vi "Civ idle3.vi"() -> ()   [LabVIEW 2013]
uses:
  <vilib>/Analysis/Matrix/Numeric/Conversions/Matrix To Array - RM.vi
  <vilib>/Analysis/Matrix/NI_Matrix.lvlib
panel:
  out "Base dissent":dbl format="%#_4g"
  out "Gold":i64 format="%^#.4g"
  out "Dissent \nmultiplication\nmodifier":dbl
  out "SP income":dbl format="%^#.3g"
  out "EP income":dbl format="%^#.3g"
  out "Land conversion rate":dbl format="%#_4e"
  out "BP income":dbl format="%^#.3g"
  in  "Ticks/s":i32
  out "Gold upkeep":dbl format="%^#_4g"
  out "Gold income/s":dbl format="%^#_4g"
  out "BP upkeep":dbl format="%^#.3g"
  out "Trading level":i32
  out "Build points":dbl format="%^#.3g"
  in  "?":T1(tab)
  out "%Hunters":dbl format="%#_3g"
  in  "%Crafters":dbl
  in  "%Engineers":dbl
  in  "%Scientists":dbl
  in  "%Builders":dbl
  in  "%Warriors":dbl
  in  "Taxes level 0":bool
  in  "Taxes level 1":bool
  in  "Taxes level 2":bool
  in  "Taxes level 3":bool
  out "Taxation\nlevel":dbl format="%#_13g"
  in  "Taxes level 4":bool
  out "Food consumption\nmultiplier":dbl
  out "Food dissent mod":dbl
  in  "Normal food\nconsumption":bool
  in  "Highest food\nconsumption":bool
  in  "Higher food\nconsumption":bool
  in  "Taxes level 5":bool
  in  "Taxes level 6":bool
  out "Military\nScience level":i32
  out "Governance\nlevel":i32
  in  "Military science":bool
  in  "Governance":bool
  in  "Physics":bool
  in  "Construction":bool
  out "Physics level":i32
  out "Construction\nlevel":i32
  out "Economics\nlevel":i32
  in  "Economics":bool
  in  "Biology":bool
  out "Biology\nlevel":i32
  out "# of level 1 sciences":i32
  out "# of level 2 sciences":i32
  out "# of level 3 sciences":i32
  out "# of level 4 sciences":i32
  out "# of level 5 sciences":i32
  out "# of level 6 sciences":i32
  out "# of level 7 sciences":i32
  out "# of level 8 sciences":i32
  out "# of level 9 sciences":i32
  out "# of level 10 sciences":i32
  out "Production\nlevel":i32
  in  "Production":bool
  out "Level 2 science price":i32 format="%^.0g"
  out "Level 1 science price":i32 format="%^.0g"
  out "Level 6 science price":i64 format="%^#.1g"
  out "Level 5 science price":i32 format="%^.0g"
  out "Level 4 science price":i32 format="%^.0g"
  out "Level 7 science price":i64 format="%^.0g"
  out "Level 3 science price":i32 format="%^#.1g"
  out "Level 8 science price":i64 format="%^.0g"
  out "Level 9 science price":i64 format="%^#.1g"
  out "Level 10 science price":i64 format="%.0g"
  out "Spear level":i32
  out "Net level":i32
  in  "Sharpened stick":bool
  in  "Net 1":bool
  in  "Net 2":bool
  in  "Stone\nspear":bool
  in  "Bronze\nSpear":bool
  in  "Iron\nSpear":bool
  out "Construction\ntools level":i32
  in  "Stone tools":bool
  in  "Basic\nmetal\ntools":bool
  in  "Advanced\nmetal\ntools":bool
  in  "Horses":bool
  in  "Selective\nbreeding":bool
  in  "Livestock":bool
  out "Animal\ndomestication\nlevel":i32
  in  "Parchment":bool
  in  "Paper":bool
  in  "Movable typeset":bool
  out "Writing level":i32
  in  "Medicine 3":bool
  in  "Medicine 2":bool
  in  "Medicine 1":bool
  out "Medicine level":i32
  in  "Medicine 4":bool
  in  "Printing\nPress":bool
  in  "Crossbow":bool
  out "Bow level":i32
  in  "Bow 1":bool
  in  "Bow 2":bool
  in  "Longbow":bool
  in  "Farming 1":bool
  out "Farming level":i32
  in  "Farming 2":bool
  out "Sword level":i32
  in  "Steel sword":bool
  in  "Iron sword":bool
  in  "Bronze sword":bool
  out "Tax method\nlevel":i32
  in  "Income tax":bool
  in  "Sales tax":bool
  in  "Tariffs":bool
  out "Siege weapon\nlevel":i32
  in  "Trebuchet":bool
  in  "Catapult":bool
  in  "Ballista":bool
  in  "Cannon":bool
  in  "Howitzer":bool
  in  "Rocket artillery":bool
  in  "Trireme":bool
  in  "Raft":bool
  out "Boat level":i32
  out "Chariot level":i32
  in  "Reinforced\nchariot":bool
  in  "Simple\nchariot":bool
  in  "Caravan":bool
  in  "Caravel":bool
  in  "Steamship":bool
  in  "Mechanical\nTelevision":bool
  out "Optics\nlevel":i32
  in  "Telescope":bool
  in  "Light bulb":bool
  in  "Camera":bool
  in  "LCD monitor":bool
  out "Electronics\nlevel":i32
  in  "Radio":bool
  in  "Computer":bool
  out "Vehicle\nlevel":i32
  in  "Steam Powered Train":bool
  in  "Internal combustion engine (cars)":bool
  in  "Aircraft":bool
  in  "Rocket":bool
  in  "Democracy":bool
  in  "Theocracy":bool
  in  "Warrior\nSociety":bool
  in  "Democracy 2":bool
  in  "Theocracy 2":bool
  in  "Warrior\nSociety 2":bool
  in  "Kingdom":bool
  in  "Republic":bool
  in  "Confederacy":bool
  in  "Senate":bool
  in  "Caste system":bool
  in  "Feudalism":bool
  in  "Harbor level 0":bool
  in  "Harbor level 3":bool
  in  "Harbor level 2":bool
  in  "Harbor level 1":bool
  out "Brick house level":i32
  out "Road level":i32
  out "Hut level":i32
  in  "Hut level 0":bool
  in  "Hut level 1":bool
  in  "Hut level 2":bool
  in  "Hut level 3":bool
  out "Road invested points":dbl
  out "Hut invested points":dbl
  in  "Road level 0":bool
  in  "Road level 3":bool
  in  "Road level 2":bool
  in  "Road level 1":bool
  out "Aqueduct level":i32
  out "Circus\ninvested points":dbl
  out "Circus/arena level":i32
  out "Aqueduct\ninvested points":dbl
  out "Harbor\ninvested points":dbl
  out "Harbor level":i32
  in  "Aqueduct\nlevel 1":bool
  in  "Aqueduct\nlevel 4":bool
  in  "Aqueduct\nlevel 3":bool
  in  "Aqueduct\nlevel 2":bool
  out "School invested points":dbl
  in  "School\nlevel 1":bool
  in  "School\nlevel 2":bool
  in  "School\nlevel 3":bool
  in  "School\nlevel 0":bool
  out "School level":i32
  in  "Wall level 1":bool
  in  "Wall level 2":bool
  in  "Wall level 3":bool
  in  "Wall level 0":bool
  out "Barracks level":i32
  out "Walls level":i32
  out "Wall invested points":dbl
  out "Barracks\ninvested points":dbl
  in  "Barracks\nlevel 3":bool
  in  "Barracks\nlevel 1":bool
  in  "Barracks\nlevel 0":bool
  in  "Barracks\nlevel 2":bool
  out "University level":i32
  in  "University\nlevel 0":bool
  in  "University\nlevel 3":bool
  in  "University\nlevel 2":bool
  in  "University\nlevel 1":bool
  out "University\ninvested points":dbl
  out "Mansion level":i32
  out "Temple level":i32
  out "Mansion\ninvested points":dbl
  out "Temple\ninvested points":dbl
  in  "Temple\nlevel 0":bool
  in  "Temple\nlevel 3":bool
  in  "Temple\nlevel 2":bool
  in  "Temple\nlevel 1":bool
  in  "Make Tier 2\nproducts":bool
  out "Tier 2\nproducts\nupkeep":dbl format="%#_13g"
  out "Tier 3\nproducts\nupkeep":dbl format="%#_13g"
  out "Tier 4\nproducts\nupkeep":dbl format="%#_13g"
  out "Tier 1\nproducts":dbl format="%#_4p"
  out "Tier 2\nproducts":dbl format="%#_13g"
  out "Tier 3\nproducts":dbl format="%#_13g"
  out "Tier 4\nproducts":dbl format="%#_13g"
  out "Tier 1\nproducts\nupkeep":dbl format="%#_13g"
  in  "Make Tier3\nproducts":bool
  in  "Make Tier 4\nproducts":bool
  out "hunting b":dbl
  out "hunting a":dbl
  out "warrior a":dbl
  out "warrior b":dbl
  out "warrior c":dbl
  out "1-Dissent/100":dbl format="%#_13g"
  out "Land conv mult":dbl
  out "Warrior b Gov mult":dbl
  out "Gov Economy\nbuildings mod":dbl
  out "Dissent mult per\nmilitary building":dbl
  out "Temp land change/s":dbl
  out "Year":i32
  out "Day":i32
  out "Military Modifier":dbl format="%#_13g"
  out "Taxation\nModifier":dbl format="%#_13g"
  out "Non-land production multiplier":dbl
  out "Hut non-land prod mod":dbl
  out "Hut upkeep":dbl
  out "Hut dissent mod":dbl
  out "Road land prod mod":dbl
  out "Road upkeep":dbl
  out "Road expansion bonus":dbl
  out "Trading level no mod":i32
  out "Taxes dissent mod":dbl
  out "Barracks military bonus":dbl
  out "Barracks upkeep":dbl
  out "Wall upkeep":dbl
  out "Wall dissent mod":dbl
  out "Construction multiplier":dbl
  out "Wall warrior % equivalent":dbl
  out "Gov building\nupkeep mod":dbl
  out "School dissent mod":dbl
  out "School upkeep":dbl
  out "School engineer equivalent":dbl
  out "School SP/EP multiplier":dbl
  out "Medicine dissent mod":dbl
  out "Gov populist\nbuildings mod":dbl
  out "Gov elitist\nbuildings mod":dbl
  out "University SP multiplier":dbl
  out "University dissent mod":dbl
  out "University upkeep":dbl
  out "University scientist equivalent":dbl
  out "Food income":dbl
  out "Gold dbl":dbl format="%#_13g"
  out "Aqueduct dissent mod":dbl
  out "Aqueduct upkeep":dbl
  out "Mansion dissent mod":dbl
  out "Mansion upkeep":dbl
  out "Harbor expansion bonus":dbl
  out "Harbor upkeep":dbl
  out "Circus dissent mod":dbl
  out "Circus upkeep":dbl
  out "Temple dissent mod":dbl
  out "Temple upkeep":dbl
  out "Harbor military mod":dbl
  out "SP/EP multiplier":dbl
  out "Temple SP/EP multiplier":dbl
  out "Aqueduct food multiplier":dbl
  out "Government":string
  out "Dissent":dbl format="%#_4g"
  out "SP":dbl format="%^#.3g"
  out "EP":dbl format="%^#.3g"
  in  "Percentage or absolute":bool
  out "Engineers":i32 format="%^#.3g"
  out "Crafters":i32 format="%^#.3g"
  out "Scientists":i32 format="%^#.3g"
  in  "#Merchants":dbl
  in  "Assign Merchant":bool
  in  "#Engineers":dbl
  in  "Assign Engineer":bool
  in  "#Scientists":dbl
  in  "Assign Scientist":bool
  out "Warriors":i32 format="%^#.3g"
  in  "Assign Builder":bool
  in  "#Builders":dbl
  out "Builders":i32 format="%^#.3g"
  in  "Assign Warrior":bool
  in  "#Warriors":dbl
  out "Unassigned workers":i32
  in  "Assign Hunters":bool
  in  "#Hunters":dbl
  in  "# people":i32
  in  "Increase\nPopulation":bool
  out "Conquered\nland":dbl format="%^#.3g"
  out "Max hunters":i32 format="%^#.3g"
  out "Hunters":i32 format="%^#.3g"
  out "Food/s":dbl format="%^#_5g"
  out "Permanent\nland":dbl format="%^#.3g"
  out "People":i64 format="%^#.3g"
  in  "Stop Loop":bool
  out "Food":dbl format="%^#_5g"
  # "Produces food, but your permanent land cannot support too many hunters"
  # "Unlock after population hits 25"
  # "Conquers land, starting at 1km^2 per warrior, but has diminishing returns"
  # "Unlock after construction 1"
  # "Produces 1 BP/tick, needed for buildings\nand for building upkeep"
  # "Unlock after population hits 100"
  # "Produces 0.1 SP/tick, used for abstract research which unlock upgrades and provide bonuses"
  # "Unlock after population hits 50"
  # "Produces 0.1 EP/tick, used for designing useful tools and upgrades"
  # "Produces Products, used mostly for late game upgrades.  Production scales with permanent land"
  # "Not yet implemented"
  # "Small income from population, 8% dissent before modifiers"
  # "Medium income from population, 15% dissent before modifiers"
  # "Higher  income from population, 25% dissent before modifiers"
  # "Higher  income from population, 40% dissent before modifiers"
  # "Highest  income from population, 60% dissent before modifiers"
  # "No income from population, no dissent added"
  # "Lowest income from population, 3% dissent before modifiers"
  # "Requires Economics 1"
  # "2 food/s/person,\n-20% dissent"
  # "1 food/s/person, no dissent mod"
  # "1.5 food/s/person,\n-10% dissent"
  # "Requires Governance 2"
  # "Each level costs 1000 *10^current level SP"
  # "Reduces diminishing returns \nfrom military size, unlocks \nnew weapons/tactics"
  # "-5% dissent per level,\nunlocks new governments"
  # "Increases EP and SP generation, \nunlocks various upgrades"
  # "Decreases building upkeep costs,\nunlocks buildings"
  # "Increase gold generation,\nunlocks gold and taxation"
  # "Increase food production,\nunlocks farming and medicine"
  # "Increases production by 20%\nper tier per level"
  # "Costs 2M EP\nRequires military 4,\nWarriors are more effective"
  # "Costs 250EP\nHunters and warriors are more effective"
  # "Costs 3000EP\nRequires military 1,\nHunters and warriors are more effective"
  # "Costs 50k EP\nRequires military 2,\nWarriors are more effective"
  # "Costs 3k EP\nRequires biology 1,\nreduces dissent by 3%"
  # "Costs 30k EP\nRequires biology 2,\nreduces dissent by another 2% (5% total)"
  # "Costs 3M EP\nRequires biology 4,\nreduces dissent by another 5% (10% total)"
  # "Costs 300M EP\nRequires biology 6,\nreduces dissent by another 5% (15% total)"
  # "Costs 10k EP\nHunters can produce more food"
  # "Costs 100k EP\nHunters can produce more food"
  # "Costs 10k EP\nImproves EP and SP production by 10%"
  # "Costs 1M EP\nImproves EP and SP production by 10%"
  # "Costs 100M EP\nImproves EP and SP production by 10%"
  # "Costs 10B EP\nImproves EP and SP production by 10%"
  # "Costs 30k EP\nRequires physics 2, construction 2\nBuilders produce 0.5 more BP/tick"
  # "Costs 500k EP\nRequires physics 3,\nconstruction 3,Builders produce 0.5 more BP/tick"
  # "Costs 200M EP\nRequires physics 5,\nconstruction 5,Builders produce 1 more BP/tick"
  # "Costs 30M EP\nRequires Biology 3\nImproves warrior effectiveness,  builder BP/tick by 0.5"
  # "Costs 30k EP\nRequires Biology 1\nImproves hunter food production"
  # "Costs 1M EP\nRequires Biology 2\nImproves warrior effectiveness,  builder BP/tick by 0.5"
  # "Costs 100k EP\nRequires military 3,\nWarriors are much more effective, hunters can produce more food"
  # "Costs 300k EP\nRequires military 3, physics 3\nWarriors and Hunters are more effective"
  # "Costs 30M EP\nRequires military 5, physics 4\nWarriors are more effective"
  # "Costs 1B EP\nRequires military 6, physics 5\nWarriors are more effective"
  # "Costs 300k EP\nRequires physics 3,\nImproves trade and hunting"
  # "Costs 3M EP\nRequires physics 4, military 3\nImproves trade and warriors"
  # "Costs 10B EP\nRequires physics 7\nIncreases trade level by 2 and improves warriors"
  # "Costs 100B EP\nRequires physics 8, military 8\nIncreases trade level by 2 and improves warriors"
  # "Costs 500k EP\nRequires Military 3, Physics 3, Improves warrior effectiveness"
  # "Costs 5M EP\nRequires Military 3, Physics 4, Improves warrior effectiveness"
  # "Costs 10M EP\nRequires Economics 4, Physics 4, Increases trade level"
  # "Costs 1M EP\nRequires Military 3\nImproves warrior effectiveness"
  # "Costs 30M EP\nRequires Military 4\nImproves warrior effectiveness"
  # "Costs 1B EP\nRequires Military 6\nImproves warrior effectiveness"
  # "Costs 1M EP\nRequires Economics 3\nImproves taxation effectiveness by 50%"
  # "Costs 30M EP\nRequires Economics 4\nImproves taxation effectiveness by 50%"
  # "Costs 1B EP\nRequires Economics 6\nImproves taxation effectiveness by 50%"
  # "Costs 10M EP\nRequires Biology 3\nRenames hunters to farmers, massive improvements to food production, increases food from tribute"
  # "Costs 100M EP\nRequires Biology 4\nLarge improvements to food production, increases food from tribute"
  # "Costs 5M EP\nRequires Military 3, Physics 4, Improves\nwarrior effectiveness"
  # "Costs 30M EP\nRequires Military 3, Physics 5, Improves\nwarrior effectiveness"
  # "Costs 300M EP\nRequires Military 4, Physics 6, Improves\nwarrior effectiveness"
  # "Costs 3B EP\nRequires Military 6, Physics 7, Improves\nwarrior effectiveness"
  # "Costs 300B EP\nRequires Military 8, Physics 9, Improves\nwarrior effectiveness"
  # "Costs 3T EP\nRequires Military 9, Physics 9, Improves\nwarrior effectiveness"
  # "Internet, not sure if invention or building"
  # "Unlock sattelite network structure"
  # "Requires Governance 1"
  # "Costs 100k SP\nRequires Governance 2"
  # "Costs 5M SP\nRequires Governance 4"
  # "Reduces dissent by 5,10,15%\nImproves non-land production by 10,20,30%\nRequires Construction 1"
  # "Upkeep:        0                          0.01BP                0.03BP              0.15BP"
  # "Cost:             0                          10k   BP              30k BP            150k BP"
  # "Increases trade level by 1,2,3\nImproves land production\n by 10,20,30%\nImproves land conversion\nrate by 20,50,100%\nRequires Construction 1"
  # "Upkeep:        0                          0.02BP                0.06BP              0.2BP"
  # "Cost:             0                          50k BP              150k BP             500k BP"
  # "Improves food output\n by 10,20,30%\nReduced dissent by 2,4,6%\nRequires Construction 3"
  # "Upkeep:              0                       0.01BP                0.03BP               0.15BP"
  # "Cost:                   0                       500k BP             1.5M BP             5M BP"
  # "Increases trade level by 1,2,3\nIncreases military effectiveness (b) by 10,20,30%\nImproves land conversion\nrate by 10,25,50%\nRequires Boat level 1"
  # "Upkeep:        0                          0.04BP                0.12BP              0.4BP"
  # "Cost:             0                          500k BP              1.5M BP           5M BP"
  # "Increases military effectiveness (b) by 10,20,30%\nRequires Construction 2, Military 2"
  # "Upkeep:        0                          0.001GP             0.003GP             0.01GP"
  # "Cost:             0                          100k BP             300k BP              1M BP"
  # "Adds to the base strength of your military, giving the equivalent of 2,4,6% of your population as warriors\nReduces dissent by 5,10,15%\nRequires Construction 3, Military 2"
  # "Upkeep:        0                          0.002GP            0.006GP            0.02GP"
  # "Cost:             0                          1M BP              3M BP               10M BP"
  # "Provides a 5,10,15% bonus to SP/EP production, reduces dissent by 2,4,6%, adds 1,2,3% of population to base  engineers\nRequires Construction 2, Governance 2"
  # "Upkeep:        0                          0.001GP             0.003GP           0.01GP"
  # "Cost:             0                          200k BP             600k BP            2M BP"
  # "Provides a 15,30,45% bonus to SP production, reduces dissent by 2,4,6%, adds 2,4,6% of population to base  scientists\nRequires Construction 2, Governance 2"
  # "Upkeep:        0                          0.005GP             0.015GP          0.05GP"
  # "Cost:             0                          600k BP             2M BP             5M BP"
  # "Reduces dissent by 3,6,9%,\nRequires Construction 1"
  # "Upkeep:        0                          0.001GP             0.003GP           0.01GP"
  # "Cost:             0                          500 GP               10k GP             500k GP"
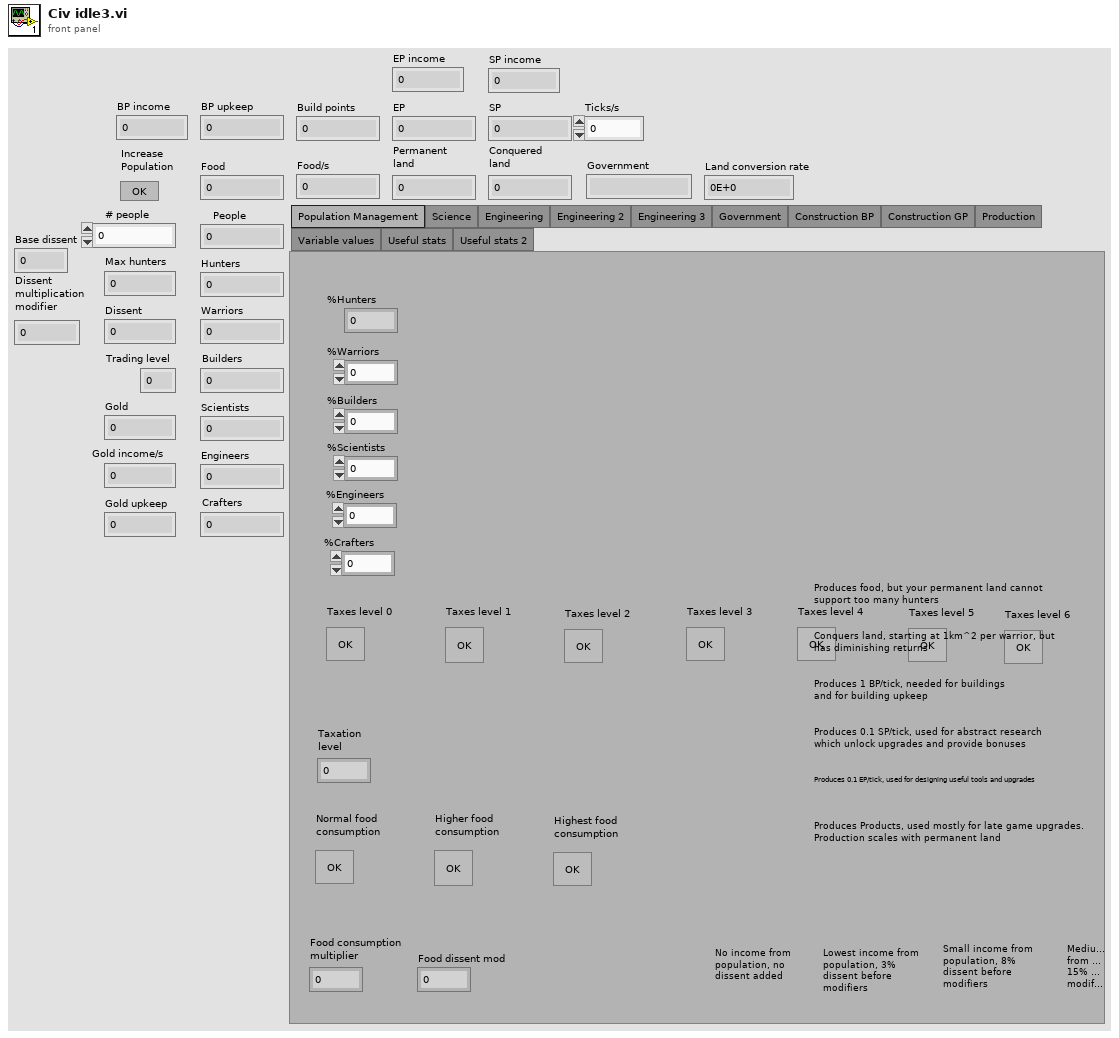
[diagram p1: front panel]
types:
  T1 = enum32{"Population Management", "Science", "Engineering", "Engineering 2", "Engineering 3", "Government", "Construction BP", "Construction GP", "Production", "Variable values", "Useful stats", "Useful stats 2"}
  T2 = typedef "NI_Matrix.lvlib/RealMatrix.ctl" = dbl[][]
diagram:
  n1 = while {
    i -> [w1979]
    stop <- "Stop Loop" stop-if-true
    w157 = 30000000 ("y")
    w166 = 30000000 ("y")
    w183 = 30000000 ("y")
    w192 = 30000000 ("y")
    w209 = 30000000 ("y")
    w224 = 30000000 ("y")
    w243 = 300000000 ("y")
    w254 = 300000000 ("y")
    w281 = 300000000 ("y")
    w292 = 30000000 ("y")
    w301 = 5000000 ("y")
    w332 = 3000000 ("y")
    w321 = 300000 ("y")
    w347 = 100000000 ("y")
    w358 = 300000000 ("y")
    w313 = 1000000000 ("y")
    w396 = 6 ("y")
    w399 = 5 ("y")
    w459 = 0 ("y")
    w458 = 3 ("y")
    w441 = 2 ("y")
    w440 = 1 ("y")
    w485 = 0 ("y")
    w486 = 3 ("y")
    w503 = 2 ("y")
    w504 = 1 ("y")
    w593 = 0 ("y")
    w592 = 3 ("y")
    w575 = 2 ("y")
    w574 = 1 ("y")
    w632 = i64 3000000000000 ("y")
    w643 = i64 300000000000 ("y")
    w664 = i64 3000000000 ("y")
    w701 = 300000000 ("y")
    w690 = 30000000 ("y")
    w681 = 5000000 ("y")
    w734 = 10000000 ("y")
    w745 = 5000000 ("y")
    w754 = 500000 ("y")
    w770 = 1000000000 ("y")
    w781 = 30000000 ("y")
    w790 = 1000000 ("y")
    w848 = 1000000000 ("y")
    w837 = 30000000 ("y")
    w828 = 1000000 ("y")
    w857 = 30000000 ("y")
    w868 = 1000000 ("y")
    w877 = 30000 ("y")
    w908 = 100000000 ("y")
    w897 = 1000000 ("y")
    w888 = 10000 ("y")
    w936 = 1 ("y")
    w928 = 2 ("y")
    w927 = 1.5 ("y")
    w971 = 0 ("y")
    w972 = 3 ("y")
    w991 = 2 ("y")
    w992 = 1 ("y")
    w1031 = 30000000 ("y")
    w1047 = 500000 ("y")
    w1065 = 3000000 ("y")
    w1076 = 30000 ("y")
    w1091 = 3000 ("y")
    w1148 = 0 ("y")
    w1147 = 3 ("y")
    w1128 = 2 ("y")
    w1127 = 1 ("y")
    w1174 = "Senate" ("y")
    w1198 = "Caste system" ("y")
    w1211 = "Feudalism" ("y")
    w1249 = "Kingdom" ("y")
    w1225 = "Republic" ("y")
    w1212 = "Confederacy" ("y")
    w1264 = 4 ("y")
    w1281 = 500000 ("y")
    w1292 = 30000 ("y")
    w1340 = 0 ("y")
    w1341 = 3 ("y")
    w1360 = 2 ("y")
    w1361 = 1 ("y")
    w1404 = 0 ("y")
    w1405 = 3 ("y")
    w1424 = 2 ("y")
    w1425 = 1 ("y")
    w1467 = 0 ("y")
    w1468 = 3 ("y")
    w1483 = 2 ("y")
    w1484 = 1 ("y")
    w1589 = 3 ("y")
    w1600 = 2 ("y")
    w1638 = 0 ("y")
    w1637 = 3 ("y")
    w1618 = 2 ("y")
    w1617 = 1 ("y")
    w1658 = 0 ("y")
    w1659 = 1 ("y")
    w1671 = 100000000 ("y")
    w1698 = 10000000 ("y")
    w1721 = 3000000 ("y")
    w1732 = 300000 ("y")
    w1764 = 300000 ("y")
    w1790 = 100000 ("y")
    w1793 = 2000000 ("y")
    w1792 = 50000 ("y")
    w1856 = "Warrior Society 2" ("y")
    w1880 = "Theocracy 2" ("y")
    w1893 = "Democracy 2" ("y")
    w1899 = "Warrior Society" ("y")
    w1912 = "Theocracy" ("y")
    w1926 = "Democracy" ("y")
    w1949 = 250 ("y")
    # "Constructions initial build"
    # "SCIENCES"
    # "GOVERNMENTS"
    # "ENGINEERING"
    n2 = local read "Food consumption\nmultiplier"() -> (w937:dbl)
    n3 = local read "Barracks\ninvested points"() -> (w1499:dbl)
    n4 = local read "Wall invested points"() -> (w1384:dbl)
    n5 = local read "Aqueduct\ninvested points"() -> (w418:dbl)
    n6 = local read "Food consumption\nmultiplier"() -> (w929:dbl)
    n7 = local read "Governance\nlevel"() -> (w934:i32)
    n8 = local read "Military\nScience level"() -> (w1326:i32)
    n9 = local read "Governance\nlevel"() -> (w942:i32)
    n10 = local read "Construction\nlevel"() -> (w1649:i32)
    n11 = local read "Construction\nlevel"() -> (w1352:i32)
    n12 = local read "Construction\nlevel"() -> (w1626:i32)
    n13 = local read "Construction\nlevel"() -> (w448:i32)
    n14 = local read "Gold dbl"() -> (w385:dbl)
    n15 = local read "Military\nScience level"() -> (w1313:i32)
    n16 = local read "Construction\nlevel"() -> (w1329:i32)
    n17 = local read "Build points"() -> (w1380:dbl)
    n18 = local read "Barracks level"() -> (w1644:i32)
    n19 = local read "Build points"() -> (w1503:dbl)
    n20 = local read "Military\nScience level"() -> (w1307:i32)
    n21 = local read "Walls level"() -> (w1334:i32)
    n22 = local read "Build points"() -> (w1643:dbl)
    n23 = local read "Build points"() -> (w1335:dbl)
    n24 = local read "Walls level"() -> (w1357:i32)
    n25 = local read "Barracks level"() -> (w1621:i32)
    n26 = local read "Build points"() -> (w422:dbl)
    n27 = Subtract(x=3000000 ("y"), y=w1384) -> (x-y=w1377:dbl)
    n28 = local read "Construction\nlevel"() -> (w469:i32)
    n29 = local read "Aqueduct level"() -> (w444:i32)
    n30 = local read "Aqueduct level"() -> (w465:i32)
    n31 = Subtract(x=300000 ("y"), y=w1499) -> (x-y=w1506:dbl)
    n32 = Greater Or Equal?(x=w942, y=2) -> (x >= y?=w944:bool)
    n33 = And(x="Normal food\nconsumption", y=w944) -> (x .and. y?=w940:bool)
    n34 = Subtract(x=10000 ("y"), y=w418) -> (x-y=w425:dbl)
    n35 = local read "Build points"() -> (w464:dbl)
    n36 = Greater Or Equal?(x=w934, y=2) -> (x >= y?=w946:bool)
    n37 = And(x="Highest food\nconsumption", y=w946) -> (x .and. y?=w932:bool)
    n38 = local read "Food consumption\nmultiplier"() -> (w918:dbl)
    n39 = local read "Ticks/s"() -> (w1255:i32)
    n40 = Not Equal?(x=w937, y=w936) -> (x != y?=w939:bool)
    n41 = And(x=w939, y=w940) -> (x .and. y?=w938:bool)
    n42 = Max & Min(x=w1377, y=0.0) -> (max(x,y)=w1382:dbl)  [unwired: 1 out]
    n43 = Greater Or Equal?(x=w1326, y=2) -> (x >= y?=w1324:bool)
    n44 = Not Equal?(x=w929, y=w928) -> (x != y?=w931:bool)
    n45 = And(x=w931, y=w932) -> (x .and. y?=w930:bool)
    n46 = local read "Aqueduct food multiplier"() -> (w471:dbl)
    n47 = Max & Min(x=w1506, y=0.0) -> (max(x,y)=w1501:dbl)  [unwired: 1 out]
    n48 = Greater Or Equal?(x=w1380, y=w1382) -> (x >= y?=w1381:bool)
    n49 = local write "Gold"(w385) -> ()
    n50 = Max & Min(x=w425, y=0.0) -> (max(x,y)=w420:dbl)  [unwired: 1 out]
    n51 = Greater Or Equal?(x=w422, y=w420) -> (x >= y?=w421:bool)
    n52 = local read "Military\nScience level"() -> (w1320:i32)
    n53 = Greater Or Equal?(x=w448, y=3) -> (x >= y?=w443:bool)
    n54 = Greater Or Equal?(x=w469, y=3) -> (x >= y?=w461:bool)
    n55 = Greater Or Equal?(x=w464, y=0) -> (x >= y?=w462:bool)
    n56 = Greater Or Equal?(x=w1503, y=w1501) -> (x >= y?=w1502:bool)
    n57 = Greater Or Equal?(x=w1649, y=2) -> (x >= y?=w1640:bool)
    n58 = Greater Or Equal?(x=w1329, y=3) -> (x >= y?=w1338:bool)
    n59 = Greater Or Equal?(x=w1643, y=0) -> (x >= y?=w1641:bool)
    n60 = Greater Or Equal?(x=w1335, y=0) -> (x >= y?=w1337:bool)
    n61 = Greater Or Equal?(x=w1352, y=3) -> (x >= y?=w1358:bool)
    n62 = Greater Or Equal?(x=w1313, y=2) -> (x >= y?=w1312:bool)
    n63 = Greater Or Equal?(x=w1626, y=2) -> (x >= y?=w1620:bool)
    n64 = Not Equal?(x=w444, y=w441) -> (x != y?=w446:bool)
    n65 = Not Equal?(x=w1644, y=w1638) -> (x != y?=w1646:bool)
    n66 = Not Equal?(x=w1334, y=w1340) -> (x != y?=w1332:bool)
    n67 = Not Equal?(x=w465, y=w459) -> (x != y?=w467:bool)
    n68 = Greater Or Equal?(x=w1307, y=2) -> (x >= y?=w1306:bool)
    n69 = Not Equal?(x=w1357, y=w1360) -> (x != y?=w1355:bool)
    n70 = Not Equal?(x=w1621, y=w1618) -> (x != y?=w1623:bool)
    n71 = for {
      N: 1 -> [_]
      tunnel: [w2874] -> w1607 mode=indexing
      n72 = local read "Production\nlevel"() -> (w2870:i32)
      n73 = local read "Permanent\nland"() -> (w2871:dbl)
      n74 = local read "Construction multiplier"() -> (w2900:dbl)
      n75 = local read "University scientist equivalent"() -> (w2887:dbl)
      n76 = local read "Taxation\nlevel"() -> (w2936:dbl)
      n77 = local read "1-Dissent/100"() -> (w2869:dbl)
      n78 = local read "Conquered\nland"() -> (w2951:dbl)
      n79 = local read "Non-land production multiplier"() -> (w2845:dbl)
      n80 = local read "Tier 2\nproducts"() -> (w2860:dbl)
      n81 = local read "Government"() -> (w2954:string)
      n82 = local read "University SP multiplier"() -> (w2884:dbl)
      n83 = local read "Economics\nlevel"() -> (w2937:i32)
      n84 = local read "SP/EP multiplier"() -> (w2893:dbl)
      n85 = local read "People"() -> (w2874:i64)
      n86 = local read "Conquered\nland"() -> (w2940:dbl)
      n87 = local read "Crafters"() -> (w2875:i32)
      n88 = local read "Economics\nlevel"() -> (w2942:i32)
      n89 = local read "Trading level"() -> (w2941:i32)
      n90 = local read "Taxation\nModifier"() -> (w2934:dbl)
      n91 = local read "Tax method\nlevel"() -> (w2878:i32)
      n92 = local read "Non-land production multiplier"() -> (w2925:dbl)
      n93 = local read "School engineer equivalent"() -> (w2896:dbl)
      n94 = local read "1-Dissent/100"() -> (w2927:dbl)
      n95 = local read "Physics level"() -> (w2928:i32)
      n96 = local read "Tier 2\nproducts\nupkeep"() -> (w2851:dbl)
      n97 = case shown="\"Imperialism\"" w2954 {
        tunnel: w2874 -> [w3002 w3009 w3029 w3047 w3055 w3074 w3085 w3107 w3122 w3144 w3157 w3177 w3190 w3219 w3231 w3244 _ _ _ _ _ _ _ _ _ _ _ _]
        tunnel: w2871 -> [_ w3019 w3030 _ _ _ _ w3112 w3121 _ w3162 _ w3192 _ _ w3246 _ _ _ _ _ _ _ _ _ _ _ _]
        tunnel: [w3005 w3016 w3022 w3044 w3058 w3067 w3087 w3104 w3120 w3133 w3150 w3171 w3186 w3207 w3227 w3239 _ _ _ _ _ _ _ _ _ _ _ _] -> w2952
        tunnel: w2951 -> [_ _ _ _ _ w3078 w3086 w3111 _ _ w3161 w3180 _ w3215 _ _ _ _ _ _ _ _ _ _ _ _ _ _]
        tunnel: [1 0.85 0.7 1 1 2 3 1.5 ("y") 1.0 ("y") 2.0 ("y") 3.0 ("y") 6.0 ("y") 0.7 ("y") 8.0 ("y") 2.0 ("y") 0.8 ("y") _ _ _ _ _ _ _ _ _ _ _ _] -> w2950
        tunnel: [1.0 2.0 4.0 1.0 1.0 0.1 0.025 1.5 ("y") 3.0 ("y") 1.0 ("y") 0.1 ("y") 0.025 ("y") 8.0 ("y") 0.015 ("y") 1.0 ("y") 8.0 ("y") _ _ _ _ _ _ _ _ _ _ _ _] -> w2949
        tunnel: [1 1 1 0.5 0.333 1 1 1.0 ("y") 0.5 ("y") 0.5 ("y") 1.0 ("y") 1.0 ("y") 1.0 ("y") 1.0 ("y") 0.5 ("y") 1.0 ("y") _ _ _ _ _ _ _ _ _ _ _ _] -> w2908
        tunnel: [1.0 ("y") 1.25 ("y") 1.5 ("y") 0.75 ("y") 0.5 ("y") 0.8 ("y") 0.7 ("y") 1.25 ("y") 2.0 ("y") 1.0 ("y") 0.5 ("y") 0.5 ("y") 2.5 ("y") 0.5 ("y") 1.0 ("y") 2.5 ("y") _ _ _ _ _ _ _ _ _ _ _ _] -> w2899
        tunnel: [1.0 ("y") 0.75 ("y") 0.5 ("y") 1.5 ("y") 2.0 ("y") 1.5 ("y") 1.5 ("y") 1.25 ("y") 0.5 ("y") 1.0 ("y") 1.5 ("y") 2.0 ("y") 0.5 ("y") 2.0 ("y") 1.0 ("y") 0.5 ("y") _ _ _ _ _ _ _ _ _ _ _ _] -> w2892
        tunnel: [1.0 ("y") 1.0 ("y") 1.0 ("y") 0.98 ("y") 0.98 ("y") 0.96 ("y") 0.96 ("y") 0.96 ("y") 1.0 ("y") 0.98 ("y") 0.96 ("y") 1.0 ("y") 1.0 ("y") 1.0 ("y") 0.98 ("y") 1.0 ("y") _ _ _ _ _ _ _ _ _ _ _ _] -> w2891
        tunnel: [1.0 ("y") _ _ _ _ _ _ 1.25 ("y") 1.5 ("y") 0.7 ("y") 0.5 ("y") 0.5 ("y") 1.0 ("y") 0.5 ("y") 0.7 ("y") 2.0 ("y") _ _ _ _ _ _ _ _ _ _ _ _] -> w2890
        frame "Tribe", Default {
          n98 = Divide(x=w3002, y=i64 4) -> (x/y=w3000:dbl)
          n99 = Subtract(x=w3000, y=i64 25) -> (x-y=w3005:dbl)
        }
        frame "Democracy" {
          n100 = Power Of X(1:w3009, 2:1.1 ("y")) -> (0:w3007:dbl)
          n101 = Square Root(x=w3019) -> (sqrt(x)=w3018:dbl)
          n102 = Divide(x=w3007, y=w3018) -> (x/y=w3017:dbl)
          n103 = Square Root(x=w3017) -> (sqrt(x)=w3021:dbl)
          n104 = Multiply(x=2, y=w3021) -> (x*y=w3016:dbl)
        }
        frame "Democracy 2" {
          n105 = Square Root(x=w3030) -> (sqrt(x)=w3034:dbl)
          n106 = Divide(x=w3029, y=w3034) -> (x/y=w3033:dbl)
          n107 = Square Root(x=w3033) -> (sqrt(x)=w3024:dbl)
          n108 = Multiply(x=w3024, y=1.9) -> (x*y=w3022:dbl)
        }
        frame "Theocracy" {
          n109 = Y-th Root of X(1:w3047, 2:i64 3 ("y")) -> (0:w3037:dbl)
          n110 = Multiply(x=w3037, y=2.0) -> (x*y=w3035:dbl)
          n111 = Add(x=w3035, y=10.0) -> (x+y=w3044:dbl)
        }
        frame "Theocracy 2" {
          n112 = Y-th Root of X(1:w3055, 2:3.5 ("y")) -> (0:w3049:dbl)
          n113 = Multiply(x=w3049, y=1.5) -> (x*y=w3050:dbl)
          n114 = Add(x=w3050, y=10.0) -> (x+y=w3058:dbl)
        }
        frame "Warrior Society" {
          n115 = Y-th Root of X(1:w3074, 2:i64 3 ("y")) -> (0:w3071:dbl)
          n116 = Y-th Root of X(1:w3078, 2:3.0 ("y")) -> (0:w3077:dbl)
          n117 = Multiply(x=3.5, y=w3071) -> (x*y=w3070:dbl)
          n118 = Add(x=w3070, y=5.0) -> (x+y=w3069:dbl)
          n119 = Multiply(x=w3077, y=2.0) -> (x*y=w3068:dbl)
          n120 = Subtract(x=w3069, y=w3068) -> (x-y=w3067:dbl)
        }
        frame "Warrior Society 2" {
          n121 = Y-th Root of X(1:w3085, 2:i64 3 ("y")) -> (0:w3095:dbl)
          n122 = Y-th Root of X(1:w3086, 2:3.0 ("y")) -> (0:w3091:dbl)
          n123 = Multiply(x=2.2, y=w3095) -> (x*y=w3096:dbl)
          n124 = Add(x=w3096, y=5.0) -> (x+y=w3097:dbl)
          n125 = Multiply(x=w3091, y=2.0) -> (x*y=w3098:dbl)
          n126 = Subtract(x=w3097, y=w3098) -> (x-y=w3087:dbl)
        }
        frame "Senate" {
          n127 = Multiply(x=w3112, y=w3111) -> (x*y=w3110:dbl)
          n128 = Power Of X(1:w3110, 2:0.3 ("y")) -> (0:w3108:dbl)
          n129 = Divide(x=w3107, y=w3108) -> (x/y=w3106:dbl)
          n130 = Y-th Root of X(1:w3106, 2:2.0 ("y")) -> (0:w3102:dbl)
          n131 = Multiply(x=1.5, y=w3102) -> (x*y=w3104:dbl)
        }
        frame "Republic" {
          n132 = Power Of X(1:w3121, 2:0.6 ("y")) -> (0:w3127:dbl)
          n133 = Divide(x=w3122, y=w3127) -> (x/y=w3126:dbl)
          n134 = Y-th Root of X(1:w3126, 2:2.0 ("y")) -> (0:w3123:dbl)
          n135 = Multiply(x=1.5, y=w3123) -> (x*y=w3120:dbl)
        }
        frame "Kingdom" {
          n136 = Power Of X(1:w3144, 2:0.25 ("y")) -> (0:w3135:dbl)
          n137 = Multiply(x=2.0, y=w3135) -> (x*y=w3133:dbl)
        }
        frame "Feudalism" {
          n138 = Multiply(x=w3162, y=w3161) -> (x*y=w3160:dbl)
          n139 = Y-th Root of X(1:w3157, 2:3.0 ("y")) -> (0:w3156:dbl)
          n140 = Y-th Root of X(1:w3160, 2:7.0 ("y")) -> (0:w3151:dbl)
          n141 = Divide(x=w3156, y=2.0) -> (x/y=w3154:dbl)
          n142 = Add(x=w3154, y=5.0) -> (x+y=w3152:dbl)
          n143 = Subtract(x=w3152, y=w3151) -> (x-y=w3150:dbl)
        }
        frame "Caste system" {
          n144 = Y-th Root of X(1:w3180, 2:3.5 ("y")) -> (0:w3167:dbl)
          n145 = Y-th Root of X(1:w3177, 2:3.5 ("y")) -> (0:w3176:dbl)
          n146 = Multiply(x=w3176, y=2.5) -> (x*y=w3174:dbl)
          n147 = Multiply(x=w3167, y=2.0) -> (x*y=w3166:dbl)
          n148 = Add(x=w3174, y=5.0) -> (x+y=w3172:dbl)
          n149 = Subtract(x=w3172, y=w3166) -> (x-y=w3171:dbl)
        }
        frame "Confederacy" {
          n150 = Power Of X(1:w3192, 2:0.55 ("y")) -> (0:w3189:dbl)
          n151 = Divide(x=w3190, y=w3189) -> (x/y=w3188:dbl)
          n152 = Square Root(x=w3188) -> (sqrt(x)=w3187:dbl)
          n153 = Multiply(x=1.7, y=w3187) -> (x*y=w3186:dbl)
        }
        frame "Imperialism" {
          n154 = Y-th Root of X(1:w3219, 2:3.75 ("y")) -> (0:w3217:dbl)
          n155 = Y-th Root of X(1:w3215, 2:3.75 ("y")) -> (0:w3213:dbl)
          n156 = Multiply(x=w3217, y=2.5) -> (x*y=w3211:dbl)
          n157 = Multiply(x=w3213, y=2.2) -> (x*y=w3210:dbl)
          n158 = Subtract(x=w3211, y=w3210) -> (x-y=w3209:dbl)
          n159 = Add(x=w3209, y=5.0) -> (x+y=w3207:dbl)
        }
        frame "Empire" {
          n160 = Y-th Root of X(1:w3231, 2:4.1 ("y")) -> (0:w3229:dbl)
          n161 = Multiply(x=w3229, y=1.5) -> (x*y=w3227:dbl)
        }
        frame "Free market capitalism" {
          n162 = Power Of X(1:w3246, 2:0.55 ("y")) -> (0:w3243:dbl)
          n163 = Divide(x=w3244, y=w3243) -> (x/y=w3242:dbl)
          n164 = Square Root(x=w3242) -> (sqrt(x)=w3241:dbl)
          n165 = Multiply(x=1.3, y=w3241) -> (x*y=w3239:dbl)
        }
        frame "Corporatism" {
        }
        frame "Fascism" {
        }
        frame "Communist dictatorship" {
        }
        frame "Socialism" {
        }
        frame "Advanced democracy?" {
        }
        frame "Advanced imperialism?" {
        }
        frame "Meritocracy" {
        }
        frame "Genetically optimized workforce" {
        }
        frame "Future democracy?" {
        }
        frame "Hivemind" {
        }
        frame "AI overlord" {
        }
        frame "Robots do all work" {
        }
      }
      n166 = Power Of X(1:w2874, 2:-0.5 ("y")) -> (0:w2872:dbl)
      n167 = Power Of X(1:1.2 ("x"), 2:w2870) -> (0:w2859:dbl)
      n168 = local read "Build points"() -> (w2902:dbl)
      n169 = local read "Build points"() -> (w2909:dbl)
      n170 = Compound Arithmetic op=MULTIPLY(w2875, w2845, w2872, w2871, w2859, w2869, 0.001 ("x")) -> (w2867:dbl)
      n171 = local read "Builders"() -> (w2911:i32)
      n172 = local read "Tier 3\nproducts"() -> (w2857:dbl)
      n173 = local read "Tier 1\nproducts"() -> (w2866:dbl)
      n174 = local read "Tier 1\nproducts\nupkeep"() -> (w2863:dbl)
      n175 = Add(x=w2867, y=w2866) -> (x+y=w2864:dbl)
      n176 = local read "Dissent"() -> (w2946:dbl)
      n177 = local read "Tier 3\nproducts\nupkeep"() -> (w2849:dbl)
      n178 = Power Of X(1:1.5 ("x"), 2:w2878) -> (0:w2876:dbl)
      n179 = local read "Tier 4\nproducts\nupkeep"() -> (w2848:dbl)
      n180 = Compound Arithmetic op=MULTIPLY(w2942, w2941, w2940, 0.001 ("value")) -> (w2907:dbl)
      n181 = local write "Dissent mult per\nmilitary building"(w2891) -> ()
      n182 = local read "Gold dbl"() -> (w2938:dbl)
      n183 = Compound Arithmetic op=MULTIPLY(w2874, w2937, w2936, w2934, 0.0005 ("value"), w2876) -> (w2906:dbl)
      n184 = local write "Gov populist\nbuildings mod"(w2899) -> ()
      n185 = local write "Gov elitist\nbuildings mod"(w2892) -> ()
      n186 = Power Of X(1:1.1 ("x"), 2:w2928) -> (0:w2913:dbl)
      n187 = Subtract(x=w2864, y=w2863) -> (x-y=w2844:dbl)
      n188 = Divide(x=w2902, y=10.0) -> (x/y=w2901:dbl)
      n189 = Compound Arithmetic op=ADD(w2938, w2907, w2906) -> (w2929:dbl)
      n190 = Divide(x=w2946, y=100.0) -> (x/y=w2948:dbl)
      n191 = local read "Dissent \nmultiplication\nmodifier"() -> (w2922:dbl)
      n192 = Compound Arithmetic op=MULTIPLY(w2913, w2927, 0.1, w2925, w2893) -> (w2914:dbl)
      n193 = Divide(x=w2914, y=w2913) -> (x/y=w2912:dbl)
      n194 = Compound Arithmetic op=MULTIPLY(w2912, 10.0 ("value"), w2911, w2900, w2893) -> (w2898:dbl)
      n195 = Add(x=w2898, y=w2909) -> (x+y=w2910:dbl)
      n196 = Less?(x=w2929, y=-50.0) -> (x < y?=w2932:bool)
      n197 = local read "Tier 4\nproducts"() -> (w2854:dbl)
      n198 = Greater?(x=w2844, y=0.0) -> (0:w2842:bool)
      n199 = Subtract(x=1.0, y=w2948) -> (x-y=w2944:dbl)
      n200 = Add(x=w2907, y=w2906) -> (x+y=w2905:dbl)
      n201 = local read "Engineers"() -> (w2895:i32)
      n202 = And(x="Make Tier 2\nproducts", y=w2842) -> (x .and. y?=w2840:bool)
      n203 = local write "Build points"(w2910) -> ()
      n204 = local write "Gold dbl"(w2929) -> ()
      n205 = local write "Gold income/s"(w2905) -> ()
      n206 = case shown="True" w2932 {
        tunnel: w2929 -> [_ w2990]
        tunnel: w2874 -> [_ w2994]
        tunnel: [0 w2991] -> w2919
        frame False {
        }
        frame True {
          n207 = Negate(x=w2990) -> (-x=w2989:dbl)
          n208 = Divide(x=w2989, y=w2994) -> (x/y=w2993:dbl)
          n209 = Max & Min(x=w2993, y=20.0) -> (min(x,y)=w2991:dbl)  [unwired: 1 out]
        }
      }
      n210 = local read "Scientists"() -> (w2888:i32)
      n211 = Less?(x=w2901, y=-50.0) -> (x < y?=w2921:bool)
      n212 = local write "1-Dissent/100"(w2944) -> ()
      n213 = local read "Taxes dissent mod"() -> (w2953:dbl)
      n214 = local write "Warrior b Gov mult"(w2950) -> ()
      n215 = Add(x=w2952, y=w2953) -> (x+y=w2829:dbl)
      n216 = case shown="True" w2840 {
        tunnel: w2844 -> [w2974 w2980]
        tunnel: w2859 -> [_ w2977]
        tunnel: [w2974 w2976] -> w2865
        tunnel: [0.0 w2975] -> w2861
        frame False {
        }
        frame True {
          n217 = Divide(x=100.0 ("y"), y=w2977) -> (x/y=w2979:dbl)
          n218 = Quotient & Remainder(x=w2980, y=w2979) -> (x-y*floor(x/y)=w2976:dbl, floor(x/y)=w2975:dbl)
        }
      }
      n219 = Add(x=w2861, y=w2860) -> (x+y=w2852:dbl)
      n220 = Subtract(x=w2852, y=w2851) -> (x-y=w2838:dbl)
      n221 = Greater?(x=w2838, y=0.0) -> (0:w2837:bool)
      n222 = And(x="Make Tier3\nproducts", y=w2837) -> (x .and. y?=w2835:bool)
      n223 = case shown="True" w2835 {
        tunnel: w2838 -> [w2966 w2972]
        tunnel: w2859 -> [_ w2969]
        tunnel: [w2966 w2968] -> w2858
        tunnel: [0.0 w2967] -> w2856
        frame False {
        }
        frame True {
          n224 = Divide(x=100.0 ("y"), y=w2969) -> (x/y=w2971:dbl)
          n225 = Quotient & Remainder(x=w2972, y=w2971) -> (x-y*floor(x/y)=w2968:dbl, floor(x/y)=w2967:dbl)
        }
      }
      n226 = local write "Tier 2\nproducts"(w2858) -> ()
      n227 = Add(x=w2856, y=w2857) -> (x+y=w2850:dbl)
      n228 = Subtract(x=w2850, y=w2849) -> (x-y=w2830:dbl)
      n229 = Greater?(x=w2830, y=0.0) -> (0:w2834:bool)
      n230 = And(x="Make Tier 4\nproducts", y=w2834) -> (x .and. y?=w2831:bool)
      n231 = case shown="True" w2831 {
        tunnel: w2830 -> [w2958 w2964]
        tunnel: w2859 -> [_ w2962]
        tunnel: [w2958 w2961] -> w2855
        tunnel: [0.0 w2960] -> w2847
        frame False {
        }
        frame True {
          n232 = Divide(x=100.0 ("y"), y=w2962) -> (x/y=w2959:dbl)
          n233 = Quotient & Remainder(x=w2964, y=w2959) -> (x-y*floor(x/y)=w2961:dbl, floor(x/y)=w2960:dbl)
        }
      }
      n234 = local write "Land conv mult"(w2949) -> ()
      n235 = Multiply(x=w2874, y=w2887) -> (x*y=w2886:dbl)
      n236 = case shown="True" w2921 {
        tunnel: w2874 -> [_ w2987]
        tunnel: [0 w2984] -> w2915
        tunnel: w2901 -> [_ w2982]
        frame False {
        }
        frame True {
          n237 = Negate(x=w2982) -> (-x=w2983:dbl)
          n238 = Divide(x=w2983, y=w2987) -> (x/y=w2986:dbl)
          n239 = Max & Min(x=w2986, y=20.0) -> (min(x,y)=w2984:dbl)  [unwired: 1 out]
        }
      }
      n240 = Add(x=w2919, y=w2915) -> (x+y=w2918:dbl)
      n241 = Multiply(x=w2829, y=w2922) -> (x*y=w2923:dbl)
      n242 = local read "EP"() -> (w2956:dbl)
      n243 = Multiply(x=w2896, y=w2874) -> (x*y=w2897:dbl)
      n244 = Subtract(x=w2847, y=w2848) -> (x-y=w2846:dbl)
      n245 = Add(x=w2846, y=w2854) -> (x+y=w2853:dbl)
      n246 = local read "SP"() -> (w2889:dbl)
      n247 = local write "Gov Economy\nbuildings mod"(w2890) -> ()
      n248 = Add(x=w2895, y=w2897) -> (x+y=w2894:dbl)
      n249 = Multiply(x=w2914, y=w2894) -> (x*y=w2883:dbl)
      n250 = local write "Gov building\nupkeep mod"(w2908) -> ()
      n251 = Max & Min(x=0.0, y=w2923) -> (max(x,y)=w2930:dbl)  [unwired: 1 out]
      n252 = Add(x=w2886, y=w2888) -> (x+y=w2885:dbl)
      n253 = Compound Arithmetic op=MULTIPLY(w2914, w2884, w2885) -> (w2882:dbl)
      n254 = Max & Min(x=w2918, y=20.0) -> (min(x,y)=w2916:dbl)  [unwired: 1 out]
      n255 = Add(x=w2916, y=w2930) -> (x+y=w2881:dbl)
      n256 = Add(x=w2956, y=w2883) -> (x+y=w2955:dbl)
      n257 = Add(x=w2889, y=w2882) -> (x+y=w2924:dbl)
      n258 = local write "Tier 3\nproducts"(w2855) -> ()
      n259 = Max & Min(x=99.0, y=w2881) -> (min(x,y)=w2879:dbl)  [unwired: 1 out]
      n260 = local write "Tier 4\nproducts"(w2853) -> ()
      n261 = local write "Tier 1\nproducts"(w2865) -> ()
      n262 = local write "BP income"(w2898) -> ()
      n263 = local write "EP"(w2955) -> ()
      n264 = local write "SP"(w2924) -> ()
      n265 = local write "SP income"(w2882) -> ()
      n266 = local write "EP income"(w2883) -> ()
      n267 = local write "Dissent"(w2879) -> ()
      n268 = Max & Min(x=w2829, y=0.0) -> (max(x,y)=→"Base dissent":dbl)  [unwired: 1 out]
    }
    n269 = case shown="True" w938 {
      tunnel: w936 -> [_ w2264]
      frame False {
      }
      frame True {
        n270 = local write "Food consumption\nmultiplier"(w2264) -> ()
        n271 = local write "Food dissent mod"(1.0 ("Taxes dissent add mod")) -> ()
      }
    }
    n272 = case shown="True" w930 {
      tunnel: w928 -> [_ w2266]
      frame False {
      }
      frame True {
        n273 = local write "Food consumption\nmultiplier"(w2266) -> ()
        n274 = local write "Food dissent mod"(0.8 ("Taxes dissent add mod")) -> ()
      }
    }
    n275 = local read "Road land prod mod"() -> (w1584:dbl)
    n276 = Max & Min(x=w1255, y=0.1) -> (max(x,y)=w1254:dbl)  [unwired: 1 out]
    n277 = local read "People"() -> (w919:i64)
    n278 = local read "hunting b"() -> (w2000:dbl)
    n279 = local read "hunting b"() -> (w1999:dbl)
    n280 = local read "Biology\nlevel"() -> (w1683:i32)
    n281 = And(x=w443, y=w421) -> (x .and. y?=w442:bool)
    n282 = And(x="Aqueduct\nlevel 3", y=w442) -> (x .and. y?=w447:bool)
    n283 = And(x=w446, y=w447) -> (x .and. y?=w445:bool)
    n284 = And(x=w461, y=w462) -> (x .and. y?=w460:bool)
    n285 = And(x="Aqueduct\nlevel 1", y=w460) -> (x .and. y?=w468:bool)
    n286 = And(x=w467, y=w468) -> (x .and. y?=w466:bool)
    n287 = case shown="True" w466 {
      tunnel: w459 -> [_ w2076]
      frame False {
      }
      frame True {
        n288 = local write "Aqueduct level"(w2076) -> ()
        n289 = local write "Aqueduct food multiplier"(1.0 ("Hut dissent add mod")) -> ()
        n290 = local write "Aqueduct dissent mod"(1.0 ("Aqueduct dissent mod")) -> ()
        n291 = local write "Aqueduct upkeep"(0.0 ("Hut non-land prod mod")) -> ()
      }
    }
    n292 = Compound Arithmetic op=AND(w1640, w1641, w1324) -> (w1639:bool)
    n293 = And(x="Barracks\nlevel 0", y=w1639) -> (x .and. y?=w1647:bool)
    n294 = And(x=w1646, y=w1647) -> (x .and. y?=w1645:bool)
    n295 = Compound Arithmetic op=AND(w1338, w1337, w1312) -> (w1339:bool)
    n296 = And(x="Wall level 0", y=w1339) -> (x .and. y?=w1331:bool)
    n297 = And(x=w1332, y=w1331) -> (x .and. y?=w1333:bool)
    n298 = Compound Arithmetic op=AND(w1358, w1381, w1306) -> (w1359:bool)
    n299 = And(x="Wall level 2", y=w1359) -> (x .and. y?=w1354:bool)
    n300 = And(x=w1355, y=w1354) -> (x .and. y?=w1356:bool)
    n301 = case shown="True" w445 {
      tunnel: w441 -> [_ w2094]
      tunnel: w420 -> [_ w2087]
      tunnel: w418 -> [_ w2086]
      frame False {
      }
      frame True {
        n302 = local read "Build points"() -> (w2093:dbl)
        n303 = Add(x=w2087, y=w2086) -> (x+y=w2089:dbl)
        n304 = local write "Aqueduct level"(w2094) -> ()
        n305 = local write "Aqueduct food multiplier"(1.2 ("Hut dissent add mod")) -> ()
        n306 = local write "Aqueduct dissent mod"(0.96 ("Hut dissent add mod")) -> ()
        n307 = local write "Aqueduct\ninvested points"(w2089) -> ()
        n308 = local write "Aqueduct upkeep"(0.03 ("Hut non-land prod mod")) -> ()
        n309 = Subtract(x=w2093, y=w2087) -> (x-y=w2092:dbl)
        n310 = local write "Build points"(w2092) -> ()
      }
    }
    n311 = local read "1-Dissent/100"() -> (w1848:dbl)
    n312 = case shown="True" w1356 {
      tunnel: w1360 -> [_ w2433]
      tunnel: w1382 -> [_ w2429]
      tunnel: w1384 -> [_ w2428]
      frame False {
      }
      frame True {
        n313 = local read "Build points"() -> (w2432:dbl)
        n314 = Add(x=w2429, y=w2428) -> (x+y=w2430:dbl)
        n315 = local write "Wall warrior % equivalent"(4.0 ("Hut dissent add mod")) -> ()
        n316 = local write "Walls level"(w2433) -> ()
        n317 = local write "Wall dissent mod"(0.9 ("Hut non-land prod mod")) -> ()
        n318 = local write "Wall invested points"(w2430) -> ()
        n319 = local write "Wall upkeep"(0.006 ("Hut non-land prod mod")) -> ()
        n320 = Subtract(x=w2432, y=w2429) -> (x-y=w2431:dbl)
        n321 = local write "Build points"(w2431) -> ()
      }
    }
    n322 = case shown="True" w1645 {
      tunnel: w1638 -> [_ w2557]
      frame False {
      }
      frame True {
        n323 = local write "Barracks level"(w2557) -> ()
        n324 = local write "Barracks military bonus"(1.0 ("Hut dissent add mod")) -> ()
        n325 = local write "Barracks upkeep"(0.0 ("Hut non-land prod mod")) -> ()
      }
    }
    n326 = case shown="True" w1333 {
      tunnel: w1340 -> [_ w2415]
      frame False {
      }
      frame True {
        n327 = local write "Wall warrior % equivalent"(0.0 ("Hut dissent add mod")) -> ()
        n328 = local write "Walls level"(w2415) -> ()
        n329 = local write "Wall dissent mod"(1.0 ("Hut non-land prod mod")) -> ()
        n330 = local write "Wall upkeep"(0.0 ("Hut non-land prod mod")) -> ()
      }
    }
    n331 = case shown="False" "Percentage or absolute" {
      frame False {
        n332 = Max & Min(x="%Scientists", y=0.0) -> (max(x,y)=w3253:dbl)  [unwired: 1 out]
        n333 = Max & Min(x="%Engineers", y=0.0) -> (max(x,y)=w3250:dbl)  [unwired: 1 out]
        n334 = Max & Min(x="%Crafters", y=0.0) -> (max(x,y)=w3247:dbl)  [unwired: 1 out]
        n335 = Max & Min(x="%Warriors", y=0.0) -> (max(x,y)=w3259:dbl)  [unwired: 1 out]
        n336 = Max & Min(x="%Builders", y=0.0) -> (max(x,y)=w3256:dbl)  [unwired: 1 out]
        n337 = Compound Arithmetic op=ADD(w3259, w3256, w3253, w3250, w3247) -> (w3262:dbl)
        n338 = Less Or Equal?(x=w3262, y=100.0) -> (x <= y?=w3264:bool)
        n339 = case shown="True" w3264 {
          tunnel: w3259 -> [_ w3292]
          tunnel: w3256 -> [_ w3291]
          tunnel: w3253 -> [_ w3290]
          tunnel: w3250 -> [_ w3289]
          tunnel: w3247 -> [_ w3288]
          frame False {
          }
          frame True {
            n340 = local read "People"() -> (w3284:i64)
            n341 = Divide(x=w3284, y=100.0) -> (x/y=w3286:dbl)
            n342 = local read "Max hunters"() -> (w3271:i32)
            n343 = Multiply(x=w3291, y=w3286) -> (x*y=w3279:dbl)
            n344 = Multiply(x=w3292, y=w3286) -> (x*y=w3268:dbl)
            n345 = Multiply(x=w3286, y=w3290) -> (x*y=w3278:dbl)
            n346 = Multiply(x=w3286, y=w3289) -> (x*y=w3277:dbl)
            n347 = Multiply(x=w3286, y=w3288) -> (x*y=w3281:dbl)
            n348 = local write "Scientists"(w3278) -> ()
            n349 = local write "Builders"(w3279) -> ()
            n350 = local write "Engineers"(w3277) -> ()
            n351 = local write "Crafters"(w3281) -> ()
            n352 = To Long Integer(number=w3277) -> (32bit integer=w3276:i32)
            n353 = To Long Integer(number=w3279) -> (32bit integer=w3274:i32)
            n354 = To Long Integer(number=w3278) -> (32bit integer=w3275:i32)
            n355 = To Long Integer(number=w3268) -> (32bit integer=w3273:i32)
            n356 = To Long Integer(number=w3281) -> (32bit integer=w3280:i32)
            n357 = Compound Arithmetic op=ADD(w3273, w3274, w3275, w3276, w3280) -> (w3285:i32)
            n358 = Subtract(x=w3284, y=w3285) -> (x-y=w3270:i64)
            n359 = Greater?(x=w3270, y=w3271) -> (0:w3272:bool)
            n360 = case shown="True" w3272 {
              tunnel: w3271 -> [_ w3297]
              tunnel: w3270 -> [w3294 w3296]
              tunnel: [w3294 w3297] -> w3265
              tunnel: [i64 0 w3295] -> w3266
              frame False {
              }
              frame True {
                n361 = Subtract(x=w3296, y=w3297) -> (x-y=w3295:i64)
              }
            }
            n362 = Divide(x=w3265, y=w3284) -> (x/y=w3283:dbl)
            n363 = Multiply(x=w3283, y=100.0) -> (x*y=→"%Hunters":dbl)
            n364 = Add(x=w3266, y=w3268) -> (x+y=w3267:dbl)
            n365 = local write "Warriors"(w3267) -> ()
            n366 = local write "Hunters"(w3265) -> ()
          }
        }
      }
      frame True {
        n367 = local read "Unassigned workers"() -> (w3361:i32)
        n368 = local read "Unassigned workers"() -> (w3370:i32)
        n369 = local read "Unassigned workers"() -> (w3335:i32)
        n370 = local read "Unassigned workers"() -> (w3325:i32)
        n371 = local read "Unassigned workers"() -> (w3354:i32)
        n372 = local read "Unassigned workers"() -> (w3315:i32)
        n373 = local read "Hunters"() -> (w3338:i32)
        n374 = local read "Scientists"() -> (w3326:i32)
        n375 = local read "Engineers"() -> (w3316:i32)
        n376 = local read "Warriors"() -> (w3340:i32)
        n377 = local read "Builders"() -> (w3339:i32)
        n378 = local read "Crafters"() -> (w3306:i32)
        n379 = Greater Or Equal?(x="#Hunters", y=0.0) -> (x >= y?=w3367:bool)
        n380 = Greater Or Equal?(x="#Scientists", y=0.0) -> (x >= y?=w3332:bool)
        n381 = Greater Or Equal?(x="#Warriors", y=0.0) -> (x >= y?=w3358:bool)
        n382 = Greater Or Equal?(x="#Engineers", y=0.0) -> (x >= y?=w3322:bool)
        n383 = Greater Or Equal?(x="#Builders", y=0.0) -> (x >= y?=w3351:bool)
        n384 = Greater Or Equal?(x="#Merchants", y=0.0) -> (x >= y?=w3312:bool)
        n385 = Add(x=w3370, y=w3338) -> (x+y=w3369:i32)
        n386 = Add(x=w3335, y=w3326) -> (x+y=w3334:i32)
        n387 = Add(x=w3361, y=w3340) -> (x+y=w3360:i32)
        n388 = Add(x=w3325, y=w3316) -> (x+y=w3324:i32)
        n389 = Add(x=w3354, y=w3339) -> (x+y=w3353:i32)
        n390 = Add(x=w3315, y=w3306) -> (x+y=w3314:i32)
        n391 = Greater Or Equal?(x=w3369, y="#Hunters") -> (x >= y?=w3366:bool)
        n392 = Greater Or Equal?(x=w3334, y="#Scientists") -> (x >= y?=w3331:bool)
        n393 = Greater Or Equal?(x=w3360, y="#Warriors") -> (x >= y?=w3357:bool)
        n394 = Greater Or Equal?(x=w3324, y="#Engineers") -> (x >= y?=w3321:bool)
        n395 = Greater Or Equal?(x=w3353, y="#Builders") -> (x >= y?=w3350:bool)
        n396 = Greater Or Equal?(x=w3314, y="#Merchants") -> (x >= y?=w3311:bool)
        n397 = And(x=w3366, y=w3367) -> (x .and. y?=w3365:bool)
        n398 = And(x=w3331, y=w3332) -> (x .and. y?=w3330:bool)
        n399 = And(x=w3357, y=w3358) -> (x .and. y?=w3356:bool)
        n400 = And(x=w3321, y=w3322) -> (x .and. y?=w3320:bool)
        n401 = And(x=w3350, y=w3351) -> (x .and. y?=w3349:bool)
        n402 = And(x=w3311, y=w3312) -> (x .and. y?=w3310:bool)
        n403 = And(x=w3365, y="Assign Hunters") -> (x .and. y?=w3363:bool)
        n404 = And(x=w3330, y="Assign Scientist") -> (x .and. y?=w3328:bool)
        n405 = And(x=w3356, y="Assign Warrior") -> (x .and. y?=w3355:bool)
        n406 = And(x=w3320, y="Assign Engineer") -> (x .and. y?=w3318:bool)
        n407 = And(x=w3349, y="Assign Builder") -> (x .and. y?=w3348:bool)
        n408 = And(x=w3310, y="Assign Merchant") -> (x .and. y?=w3308:bool)
        n409 = case shown="True" w3363 {
          tunnel: "#Hunters" -> [_ w3382]
          tunnel: [w3381 w3382] -> w3346
          tunnel: w3338 -> [w3381 _]
          frame False {
          }
          frame True {
            n410 = local write "Hunters"(w3382) -> ()
          }
        }
        n411 = case shown="True" w3328 {
          tunnel: "#Scientists" -> [_ w3376]
          tunnel: [w3375 w3376] -> w3303
          tunnel: w3326 -> [w3375 _]
          frame False {
          }
          frame True {
            n412 = local write "Scientists"(w3376) -> ()
          }
        }
        n413 = case shown="True" w3355 {
          tunnel: "#Warriors" -> [_ w3380]
          tunnel: [w3379 w3380] -> w3341
          tunnel: w3340 -> [w3379 _]
          frame False {
          }
          frame True {
            n414 = local write "Warriors"(w3380) -> ()
          }
        }
        n415 = case shown="True" w3318 {
          tunnel: "#Engineers" -> [_ w3374]
          tunnel: [w3373 w3374] -> w3302
          tunnel: w3316 -> [w3373 _]
          frame False {
          }
          frame True {
            n416 = local write "Engineers"(w3374) -> ()
          }
        }
        n417 = case shown="True" w3348 {
          tunnel: "#Builders" -> [_ w3378]
          tunnel: [w3377 w3378] -> w3304
          tunnel: w3339 -> [w3377 _]
          frame False {
          }
          frame True {
            n418 = local write "Builders"(w3378) -> ()
          }
        }
        n419 = case shown="True" w3308 {
          tunnel: "#Merchants" -> [_ w3372]
          tunnel: [w3371 w3372] -> w3301
          tunnel: w3306 -> [w3371 _]
          frame False {
          }
          frame True {
            n420 = local write "Crafters"(w3372) -> ()
          }
        }
        n421 = local read "People"() -> (w3343:i64)
        n422 = Add(x=w3302, y=w3301) -> (x+y=w3300:dbl)
        n423 = Add(x=w3304, y=w3303) -> (x+y=w3299:dbl)
        n424 = Add(x=w3346, y=w3341) -> (x+y=w3345:dbl)
        n425 = Add(x=w3299, y=w3300) -> (x+y=w3298:dbl)
        n426 = Add(x=w3345, y=w3298) -> (x+y=w3344:dbl)
        n427 = Subtract(x=w3343, y=w3344) -> (x-y=w3342:dbl)
        n428 = local write "Unassigned workers"(w3342) -> ()
      }
    }
    n429 = Reciprocal(x=w1254) -> (1/x=w1251:dbl)
    n430 = local read "Military\nScience level"() -> (w1309:i32)
    n431 = Multiply(x=w919, y=w918) -> (x*y=w916:dbl)
    n432 = local read "Permanent\nland"() -> (w1713:dbl)
    n433 = Greater Or Equal?(x=w1320, y=2) -> (x >= y?=w1318:bool)
    n434 = Compound Arithmetic op=AND(w1620, w1502, w1318) -> (w1619:bool)
    n435 = And(x="Barracks\nlevel 2", y=w1619) -> (x .and. y?=w1624:bool)
    n436 = And(x=w1623, y=w1624) -> (x .and. y?=w1622:bool)
    n437 = case shown="True" w1622 {
      tunnel: w1618 -> [_ w2573]
      tunnel: w1501 -> [_ w2569]
      tunnel: w1499 -> [_ w2568]
      frame False {
      }
      frame True {
        n438 = local read "Build points"() -> (w2572:dbl)
        n439 = Add(x=w2569, y=w2568) -> (x+y=w2570:dbl)
        n440 = local write "Barracks level"(w2573) -> ()
        n441 = local write "Barracks military bonus"(1.2 ("Hut dissent add mod")) -> ()
        n442 = local write "Barracks\ninvested points"(w2570) -> ()
        n443 = local write "Barracks upkeep"(0.003 ("Hut non-land prod mod")) -> ()
        n444 = Subtract(x=w2572, y=w2569) -> (x-y=w2571:dbl)
        n445 = local write "Build points"(w2571) -> ()
      }
    }
    n446 = local read "Food"() -> (w1998:dbl)
    n447 = local read "Hunters"() -> (w1849:i32)
    n448 = Multiply(x=w1251, y=1000.0) -> (x*y=w1253:dbl)
    n449 = local read "hunting a"() -> (w1997:dbl)
    n450 = local read "Military\nScience level"() -> (w1322:i32)
    n451 = local read "Barracks\ninvested points"() -> (w1500:dbl)
    n452 = Power Of X(1:1.05 ("x"), 2:w1683) -> (0:w473:dbl)
    n453 = local read "Wall invested points"() -> (w1383:dbl)
    n454 = Wait (ms)(milliseconds to wait=w1253) -> ()  [unwired: 1 out]
    n455 = local read "Aqueduct\ninvested points"() -> (w419:dbl)
    n456 = Greater Or Equal?(x=w1309, y=2) -> (x >= y?=w1310:bool)
    n457 = Compound Arithmetic op=MULTIPLY(w1849, w1584, w1848) -> (w1847:dbl)
    n458 = Multiply(x=w473, y=w471) -> (x*y=w472:dbl)
    n459 = local read "1-Dissent/100"() -> (w1854:dbl)
    n460 = local read "hunting a"() -> (w1855:dbl)
    n461 = local read "Barracks\ninvested points"() -> (w1492:dbl)
    n462 = local read "Wall invested points"() -> (w1391:dbl)
    n463 = local read "Aqueduct\ninvested points"() -> (w411:dbl)
    n464 = Multiply(x=w1713, y=w2000) -> (x*y=w2016:dbl)
    n465 = local read "Governance\nlevel"() -> (w921:i32)
    n466 = local read "Construction\nlevel"() -> (w1369:i32)
    n467 = Multiply(x=w1997, y=w1847) -> (x*y=w2009:dbl)
    n468 = local read "Food consumption\nmultiplier"() -> (w926:dbl)
    n469 = Multiply(x=w2016, y=5) -> (x*y=w2014:dbl)
    n470 = local read "Build points"() -> (w1509:dbl)
    n471 = local read "Build points"() -> (w1374:dbl)
    n472 = local read "Construction\nlevel"() -> (w1609:i32)
    n473 = local read "Construction\nlevel"() -> (w433:i32)
    n474 = Multiply(x=w2009, y=0.1 ("x")) -> (x*y=w2019:dbl)
    n475 = Subtract(x=100000 ("y"), y=w1500) -> (x-y=w1512:dbl)
    n476 = Subtract(x=1000000 ("y"), y=w1383) -> (x-y=w1371:dbl)
    n477 = local read "Build points"() -> (w428:dbl)
    n478 = local read "Wall warrior % equivalent"() -> (w1267:dbl)
    n479 = Multiply(x=w1855, y=w1854) -> (x*y=w1853:dbl)
    n480 = Quotient & Remainder(x=w2014, y=w1853) -> (floor(x/y)=→"Max hunters":dbl)  [unwired: 1 out]
    n481 = local read "Construction\nlevel"() -> (w1349:i32)
    n482 = Subtract(x=500 ("y"), y=w419) -> (x-y=w431:dbl)
    n483 = local read "Construction\nlevel"() -> (w1629:i32)
    n484 = local read "Build points"() -> (w1385:dbl)
    n485 = local read "Barracks level"() -> (w1614:i32)
    n486 = Divide(x=w2019, y=w1713) -> (x/y=w2018:dbl)
    n487 = local read "Walls level"() -> (w1344:i32)
    n488 = local read "Barracks level"() -> (w1634:i32)
    n489 = local read "Construction\nlevel"() -> (w451:i32)
    n490 = local read "Build points"() -> (w1498:dbl)
    n491 = local read "Walls level"() -> (w1364:i32)
    n492 = local read "Aqueduct level"() -> (w455:i32)
    n493 = Greater Or Equal?(x=w1322, y=2) -> (x >= y?=w1321:bool)
    n494 = local read "Build points"() -> (w417:dbl)
    n495 = Greater Or Equal?(x=w1609, y=2) -> (x >= y?=w1615:bool)
    n496 = Subtract(x=10000000 ("y"), y=w1391) -> (x-y=w1388:dbl)
    n497 = local read "Aqueduct level"() -> (w437:i32)
    n498 = Max & Min(x=w1512, y=0.0) -> (max(x,y)=w1507:dbl)  [unwired: 1 out]
    n499 = Max & Min(x=w1371, y=0.0) -> (max(x,y)=w1376:dbl)  [unwired: 1 out]
    n500 = Multiply(x=100, y="# people") -> (x*y=w1984:i32)
    n501 = Subtract(x=1000000 ("y"), y=w1492) -> (x-y=w1495:dbl)
    n502 = Subtract(x=w1999, y=w2018) -> (x-y=w2017:dbl)
    n503 = local read "Conquered\nland"() -> (w1712:dbl)
    n504 = Greater Or Equal?(x=w1509, y=w1507) -> (x >= y?=w1508:bool)
    n505 = Greater Or Equal?(x=w1374, y=w1376) -> (x >= y?=w1375:bool)
    n506 = Multiply(x=w2009, y=w2017) -> (x*y=w2008:dbl)
    n507 = Subtract(x=500000 ("y"), y=w411) -> (x-y=w414:dbl)
    n508 = local read "Farming level"() -> (w1681:i32)
    n509 = local read "Trading level"() -> (w1582:i32)
    n510 = Max & Min(x=w431, y=0.0) -> (max(x,y)=w426:dbl)  [unwired: 1 out]
    n511 = Greater Or Equal?(x=w428, y=w426) -> (x >= y?=w427:bool)
    n512 = local read "Road land prod mod"() -> (w1583:dbl)
    n513 = Max & Min(x=w1388, y=0.0) -> (max(x,y)=w1390:dbl)  [unwired: 1 out]
    n514 = Greater Or Equal?(x=w921, y=2) -> (x >= y?=w945:bool)
    n515 = And(x="Higher food\nconsumption", y=w945) -> (x .and. y?=w923:bool)
    n516 = Max & Min(x=w1495, y=0.0) -> (max(x,y)=w1493:dbl)  [unwired: 1 out]
    n517 = Greater Or Equal?(x=w1385, y=w1390) -> (x >= y?=w1389:bool)
    n518 = Greater Or Equal?(x=w1349, y=3) -> (x >= y?=w1343:bool)
    n519 = Max & Min(x=w414, y=0.0) -> (max(x,y)=w412:dbl)  [unwired: 1 out]
    n520 = Greater Or Equal?(x=w1498, y=w1493) -> (x >= y?=w1494:bool)
    n521 = Greater Or Equal?(x=w1369, y=3) -> (x >= y?=w1363:bool)
    n522 = Compound Arithmetic op=AND(w1615, w1508, w1321) -> (w1616:bool)
    n523 = And(x="Barracks\nlevel 1", y=w1616) -> (x .and. y?=w1611:bool)
    n524 = Compound Arithmetic op=AND(w1363, w1375, w1310) -> (w1362:bool)
    n525 = And(x="Wall level 1", y=w1362) -> (x .and. y?=w1367:bool)
    n526 = Greater Or Equal?(x=w1629, y=2) -> (x >= y?=w1635:bool)
    n527 = Greater Or Equal?(x=w417, y=w412) -> (x >= y?=w413:bool)
    n528 = Not Equal?(x=w926, y=w927) -> (x != y?=w924:bool)
    n529 = And(x=w924, y=w923) -> (x .and. y?=w925:bool)
    n530 = Greater Or Equal?(x=w451, y=3) -> (x >= y?=w456:bool)
    n531 = Not Equal?(x=w1344, y=w1341) -> (x != y?=w1346:bool)
    n532 = Not Equal?(x=w1614, y=w1617) -> (x != y?=w1612:bool)
    n533 = And(x=w1612, y=w1611) -> (x .and. y?=w1613:bool)
    n534 = Not Equal?(x=w1364, y=w1361) -> (x != y?=w1366:bool)
    n535 = And(x=w1366, y=w1367) -> (x .and. y?=w1365:bool)
    n536 = Greater Or Equal?(x=w433, y=3) -> (x >= y?=w438:bool)
    n537 = And(x=w438, y=w427) -> (x .and. y?=w439:bool)
    n538 = And(x="Aqueduct\nlevel 2", y=w439) -> (x .and. y?=w434:bool)
    n539 = Not Equal?(x=w1634, y=w1637) -> (x != y?=w1632:bool)
    n540 = Greater?(x="# people", y=0.0) -> (0:w605:bool)
    n541 = Not Equal?(x=w455, y=w458) -> (x != y?=w453:bool)
    n542 = And(x=w456, y=w413) -> (x .and. y?=w457:bool)
    n543 = And(x="Aqueduct\nlevel 4", y=w457) -> (x .and. y?=w452:bool)
    n544 = And(x=w453, y=w452) -> (x .and. y?=w454:bool)
    n545 = Not Equal?(x=w437, y=w440) -> (x != y?=w435:bool)
    n546 = And(x=w435, y=w434) -> (x .and. y?=w436:bool)
    n547 = case shown="True" w454 {
      tunnel: w458 -> [_ w2085]
      tunnel: w412 -> [_ w2078]
      tunnel: w411 -> [_ w2077]
      frame False {
      }
      frame True {
        n548 = local read "Build points"() -> (w2084:dbl)
        n549 = Add(x=w2078, y=w2077) -> (x+y=w2079:dbl)
        n550 = local write "Aqueduct level"(w2085) -> ()
        n551 = local write "Aqueduct food multiplier"(1.3 ("Hut dissent add mod")) -> ()
        n552 = local write "Aqueduct dissent mod"(0.94 ("Hut dissent add mod")) -> ()
        n553 = local write "Aqueduct\ninvested points"(w2079) -> ()
        n554 = local write "Aqueduct upkeep"(0.15 ("Hut non-land prod mod")) -> ()
        n555 = Subtract(x=w2084, y=w2078) -> (x-y=w2083:dbl)
        n556 = local write "Build points"(w2083) -> ()
      }
    }
    n557 = case shown="True" w925 {
      tunnel: w927 -> [_ w2268]
      frame False {
      }
      frame True {
        n558 = local write "Food consumption\nmultiplier"(w2268) -> ()
        n559 = local write "Food dissent mod"(0.9 ("Taxes dissent add mod")) -> ()
      }
    }
    n560 = local read "1-Dissent/100"() -> (w1851:dbl)
    n561 = local read "Military\nScience level"() -> (w1305:i32)
    n562 = Multiply(x=w1582, y=0.5) -> (x*y=w1581:dbl)
    n563 = Increment(x=w1681) -> (x+1=w1679:i32)
    n564 = local read "Military\nScience level"() -> (w1316:i32)
    n565 = case shown="True" w1613 {
      tunnel: w1617 -> [_ w2581]
      tunnel: w1500 -> [_ w2578]
      tunnel: w1507 -> [_ w2576]
      frame False {
      }
      frame True {
        n566 = local read "Build points"() -> (w2580:dbl)
        n567 = Add(x=w2576, y=w2578) -> (x+y=w2577:dbl)
        n568 = local write "Barracks level"(w2581) -> ()
        n569 = local write "Barracks military bonus"(1.1 ("Hut dissent add mod")) -> ()
        n570 = local write "Barracks\ninvested points"(w2577) -> ()
        n571 = local write "Barracks upkeep"(0.001 ("Hut non-land prod mod")) -> ()
        n572 = Subtract(x=w2580, y=w2576) -> (x-y=w2579:dbl)
        n573 = local write "Build points"(w2579) -> ()
      }
    }
    n574 = case shown="True" w1365 {
      tunnel: w1361 -> [_ w2442]
      tunnel: w1383 -> [_ w2439]
      tunnel: w1376 -> [_ w2437]
      frame False {
      }
      frame True {
        n575 = local read "Build points"() -> (w2441:dbl)
        n576 = Add(x=w2437, y=w2439) -> (x+y=w2438:dbl)
        n577 = local write "Walls level"(w2442) -> ()
        n578 = local write "Wall warrior % equivalent"(2.0 ("Hut dissent add mod")) -> ()
        n579 = local write "Wall invested points"(w2438) -> ()
        n580 = local write "Wall dissent mod"(0.95 ("Hut non-land prod mod")) -> ()
        n581 = Subtract(x=w2441, y=w2437) -> (x-y=w2440:dbl)
        n582 = local write "Wall upkeep"(0.002 ("Hut non-land prod mod")) -> ()
        n583 = local write "Build points"(w2440) -> ()
      }
    }
    n584 = local read "Warriors"() -> (w1270:i32)
    n585 = Increment(x=w1581) -> (x+1=w1680:dbl)
    n586 = local read "warrior a"() -> (w1852:dbl)
    n587 = case shown="True" w436 {
      tunnel: w440 -> [_ w2103]
      tunnel: w419 -> [_ w2097]
      tunnel: w426 -> [_ w2095]
      frame False {
      }
      frame True {
        n588 = local read "Build points"() -> (w2102:dbl)
        n589 = Add(x=w2095, y=w2097) -> (x+y=w2096:dbl)
        n590 = local write "Aqueduct level"(w2103) -> ()
        n591 = local write "Aqueduct food multiplier"(1.1 ("Hut dissent add mod")) -> ()
        n592 = local write "Aqueduct\ninvested points"(w2096) -> ()
        n593 = local write "Aqueduct dissent mod"(0.98 ("Hut dissent add mod")) -> ()
        n594 = local write "Aqueduct upkeep"(0.01 ("Hut non-land prod mod")) -> ()
        n595 = Subtract(x=w2102, y=w2095) -> (x-y=w2101:dbl)
        n596 = local write "Build points"(w2101) -> ()
      }
    }
    n597 = Compound Arithmetic op=MULTIPLY(w1712, w1679, w1680) -> (w915:dbl)
    n598 = Add(x=w2008, y=w915) -> (x+y=w914:dbl)
    n599 = Multiply(x=w472, y=w914) -> (x*y=w913:dbl)
    n600 = Subtract(x=w913, y=w916) -> (x-y=w917:dbl)
    "Food/s" <- w917
    n601 = Add(x=w1998, y=w917) -> (x+y=w1983:dbl)
    n602 = Greater?(x=w1983, y=w1984) -> (0:w1987:bool)
    n603 = Compound Arithmetic op=AND(w1987, w605, "Increase\nPopulation") -> (w1986:bool)
    n604 = case shown="False" w1986 {
      tunnel: w919 -> [_ w3426]
      tunnel: w1984 -> [_ w3424]
      tunnel: w1983 -> [w3408 w3423]
      tunnel: [w3407 w3422] -> w1981
      tunnel: "# people" -> [_ w3421]
      frame False {
        n605 = Less?(x=w3408, y=-100.0) -> (x < y?=w3410:bool)
        n606 = case shown="True" w3410 {
          tunnel: w3408 -> [w3411 w3415]
          tunnel: [w3411 w3412] -> w3407
          frame False {
          }
          frame True {
            n607 = local read "People"() -> (w3413:i64)
            n608 = Quotient & Remainder(x=w3415, y=100.0) -> (floor(x/y)=w3419:dbl)  [unwired: 1 out]
            n609 = Increment(x=w3419) -> (x+1=w3416:dbl)
            n610 = Add(x=w3413, y=w3416) -> (x+y=w3418:dbl)
            n611 = local write "People"(w3418) -> ()
            n612 = Multiply(x=w3416, y=-50.0) -> (x*y=w3414:dbl)
            n613 = Add(x=w3414, y=w3415) -> (x+y=w3412:dbl)
          }
        }
      }
      frame True {
        n614 = Add(x=w3426, y=w3421) -> (x+y=w3425:i64)
        n615 = Subtract(x=w3423, y=w3424) -> (x-y=w3422:dbl)
        n616 = local write "People"(w3425) -> ()
      }
    }
    n617 = Compound Arithmetic op=MULTIPLY(w919, 0.01 ("value"), w1267) -> (w1266:dbl)
    n618 = local write "Food income"(w913) -> ()
    n619 = Greater Or Equal?(x=w1305, y=2) -> (x >= y?=w1303:bool)
    n620 = Compound Arithmetic op=AND(w1343, w1389, w1303) -> (w1342:bool)
    n621 = And(x="Wall level 3", y=w1342) -> (x .and. y?=w1347:bool)
    n622 = And(x=w1346, y=w1347) -> (x .and. y?=w1345:bool)
    n623 = case shown="True" w1345 {
      tunnel: w1341 -> [_ w2424]
      tunnel: w1390 -> [_ w2420]
      tunnel: w1391 -> [_ w2419]
      frame False {
      }
      frame True {
        n624 = local read "Build points"() -> (w2423:dbl)
        n625 = Add(x=w2420, y=w2419) -> (x+y=w2421:dbl)
        n626 = local write "Walls level"(w2424) -> ()
        n627 = local write "Wall warrior % equivalent"(6.0 ("Hut dissent add mod")) -> ()
        n628 = local write "Wall invested points"(w2421) -> ()
        n629 = local write "Wall dissent mod"(0.85 ("Hut non-land prod mod")) -> ()
        n630 = Subtract(x=w2423, y=w2420) -> (x-y=w2422:dbl)
        n631 = local write "Wall upkeep"(0.02 ("Hut non-land prod mod")) -> ()
        n632 = local write "Build points"(w2422) -> ()
      }
    }
    n633 = Add(x=w1266, y=w1270) -> (x+y=w1269:dbl)
    n634 = Compound Arithmetic op=MULTIPLY(w1852, w1583, w1851) -> (w1850:dbl)
    n635 = Multiply(x=w1269, y=w1850) -> (x*y=w2013:dbl)
    n636 = local read "School invested points"() -> (w1104:dbl)
    n637 = Greater Or Equal?(x=w1316, y=2) -> (x >= y?=w1315:bool)
    n638 = Compound Arithmetic op=AND(w1635, w1494, w1315) -> (w1636:bool)
    n639 = And(x="Barracks\nlevel 3", y=w1636) -> (x .and. y?=w1631:bool)
    n640 = And(x=w1632, y=w1631) -> (x .and. y?=w1633:bool)
    n641 = case shown="True" w1633 {
      tunnel: w1637 -> [_ w2565]
      tunnel: w1493 -> [_ w2561]
      tunnel: w1492 -> [_ w2560]
      frame False {
      }
      frame True {
        n642 = local read "Build points"() -> (w2564:dbl)
        n643 = Add(x=w2561, y=w2560) -> (x+y=w2562:dbl)
        n644 = local write "Barracks level"(w2565) -> ()
        n645 = local write "Barracks\ninvested points"(w2562) -> ()
        n646 = local write "Barracks military bonus"(1.3 ("Hut dissent add mod")) -> ()
        n647 = local write "Barracks upkeep"(0.01 ("Hut non-land prod mod")) -> ()
        n648 = Subtract(x=w2564, y=w2561) -> (x-y=w2563:dbl)
        n649 = local write "Build points"(w2563) -> ()
      }
    }
    n650 = local read "Construction\nlevel"() -> (w1136:i32)
    n651 = local read "Construction\nlevel"() -> (w1159:i32)
    n652 = local read "Hut invested points"() -> (w1521:dbl)
    n653 = local read "School level"() -> (w1154:i32)
    n654 = for {
      tunnel: w1607 -> [w2683] mode=indexing
      # "Science prices"
      # "Construction upkeep"
      n655 = local read "# of level 1 sciences"() -> (w2637:i32)
      n656 = local read "Aqueduct upkeep"() -> (w2646:dbl)
      n657 = local read "# of level 2 sciences"() -> (w2631:i32)
      n658 = local read "# of level 3 sciences"() -> (w2629:i32)
      n659 = local read "Harbor upkeep"() -> (w2652:dbl)
      n660 = local read "Road upkeep"() -> (w2688:dbl)
      n661 = local read "Gov building\nupkeep mod"() -> (w2684:dbl)
      n662 = local read "Hut upkeep"() -> (w2689:dbl)
      n663 = local read "Barracks upkeep"() -> (w2682:dbl)
      n664 = local read "University upkeep"() -> (w2662:dbl)
      n665 = local read "School upkeep"() -> (w2663:dbl)
      n666 = local read "Temple upkeep"() -> (w2649:dbl)
      n667 = local read "Construction\nlevel"() -> (w2693:i32)
      n668 = local read "Wall upkeep"() -> (w2681:dbl)
      n669 = local read "Build points"() -> (w2699:dbl)
      n670 = Compound Arithmetic op=ADD(w2689, w2688, w2652, w2646) -> (w2687:dbl)
      n671 = Power Of 2(x=w2637) -> (2^x=w2636:dbl)
      n672 = Power Of 2(x=w2631) -> (2^x=w2632:dbl)
      n673 = Power Of 2(x=w2629) -> (2^x=w2628:dbl)
      n674 = Compound Arithmetic op=ADD(w2682, w2681, w2663, w2662, w2649) -> (w2680:dbl)
      n675 = Multiply(x=w2683, y=w2687) -> (x*y=w2686:dbl)
      n676 = Multiply(x=0.05, y=w2693) -> (x*y=w2692:dbl)
      n677 = Multiply(x=w2683, y=w2680) -> (x*y=w2679:dbl)
      n678 = Multiply(x=w2636, y=1000.0) -> (x*y=→"Level 1 science price":dbl)
      n679 = Multiply(x=w2632, y=10000.0) -> (x*y=→"Level 2 science price":dbl)
      n680 = Multiply(x=w2628, y=100000.0) -> (x*y=→"Level 3 science price":dbl)
      n681 = Subtract(x=1.0, y=w2692) -> (x-y=w2685:dbl)
      n682 = Compound Arithmetic op=MULTIPLY(w2686, w2685, w2684) -> (w2672:dbl)
      n683 = Subtract(x=w2699, y=w2672) -> (x-y=w2691:dbl)
      n684 = local read "Gold dbl"() -> (w2678:dbl)
      n685 = Compound Arithmetic op=MULTIPLY(w2685, w2684, w2679) -> (w2676:dbl)
      n686 = local write "Build points"(w2691) -> ()
      n687 = local write "BP upkeep"(w2672) -> ()
      n688 = local write "Gold upkeep"(w2676) -> ()
      n689 = Subtract(x=w2678, y=w2676) -> (x-y=w2677:dbl)
      n690 = local read "# of level 6 sciences"() -> (w2615:i32)
      n691 = local read "# of level 5 sciences"() -> (w2621:i32)
      n692 = local write "Gold dbl"(w2677) -> ()
      n693 = local read "# of level 4 sciences"() -> (w2623:i32)
      n694 = local read "Dissent mult per\nmilitary building"() -> (w2640:dbl)
      n695 = local read "School dissent mod"() -> (w2671:dbl)
      n696 = local read "Temple dissent mod"() -> (w2648:dbl)
      n697 = local read "Governance\nlevel"() -> (w2643:i32)
      n698 = local read "Barracks level"() -> (w2668:i32)
      n699 = local read "Harbor level"() -> (w2651:i32)
      n700 = local read "Walls level"() -> (w2669:i32)
      n701 = local read "Gov elitist\nbuildings mod"() -> (w2665:dbl)
      n702 = local read "University dissent mod"() -> (w2667:dbl)
      n703 = local read "Aqueduct dissent mod"() -> (w2645:dbl)
      n704 = local read "Hut dissent mod"() -> (w2690:dbl)
      n705 = local read "Gov populist\nbuildings mod"() -> (w2675:dbl)
      n706 = Power Of 2(x=w2615) -> (2^x=w2616:dbl)
      n707 = Power Of 2(x=w2621) -> (2^x=w2620:dbl)
      n708 = local read "Medicine dissent mod"() -> (w2658:dbl)
      n709 = Power Of 2(x=w2623) -> (2^x=w2624:dbl)
      n710 = Multiply(x=w2616, y=100000000.0) -> (x*y=→"Level 6 science price":dbl)
      n711 = Multiply(x=w2620, y=10000000.0) -> (x*y=→"Level 5 science price":dbl)
      n712 = Multiply(x=w2624, y=1000000.0) -> (x*y=→"Level 4 science price":dbl)
      n713 = local read "Wall dissent mod"() -> (w2670:dbl)
      n714 = Compound Arithmetic op=MULTIPLY(w2648, w2667) -> (w2666:dbl)
      n715 = Compound Arithmetic op=ADD(w2669, w2668, w2651) -> (w2639:i32)
      n716 = Compound Arithmetic op=MULTIPLY(w2690, w2671) -> (w2644:dbl)
      n717 = Power Of X(1:0.95 ("x"), 2:w2643) -> (0:w2641:dbl)
      n718 = Power Of X(1:w2666, 2:w2665) -> (0:w2664:dbl)
      n719 = Power Of X(1:w2640, 2:w2639) -> (0:w2638:dbl)
      n720 = Power Of X(1:w2644, 2:w2675) -> (0:w2674:dbl)
      n721 = local read "# of level 10 sciences"() -> (w2599:i32)
      n722 = local read "# of level 8 sciences"() -> (w2607:i32)
      n723 = local read "# of level 9 sciences"() -> (w2605:i32)
      n724 = local read "# of level 7 sciences"() -> (w2613:i32)
      n725 = local read "Writing level"() -> (w2654:i32)
      n726 = local read "Temple SP/EP multiplier"() -> (w2647:dbl)
      n727 = local read "School SP/EP multiplier"() -> (w2657:dbl)
      n728 = local read "Trading level no mod"() -> (w2698:i32)
      n729 = local read "Food dissent mod"() -> (w2661:dbl)
      n730 = Compound Arithmetic op=MULTIPLY(w2674, w2658, w2661, w2641, w2645, w2670, w2638, w2664) -> (w2673:dbl)
      n731 = local read "Hut non-land prod mod"() -> (w2660:dbl)
      n732 = local read "Harbor level"() -> (w2650:i32)
      n733 = local read "Road level"() -> (w2697:i32)
      n734 = Power Of 2(x=w2599) -> (2^x=w2600:dbl)
      n735 = Power Of 2(x=w2607) -> (2^x=w2608:dbl)
      n736 = Power Of 2(x=w2605) -> (2^x=w2604:dbl)
      n737 = local write "Dissent \nmultiplication\nmodifier"(w2673) -> ()
      n738 = Power Of 2(x=w2613) -> (2^x=w2612:dbl)
      n739 = Power Of X(1:1.1 ("x"), 2:w2654) -> (0:w2653:dbl)
      n740 = Multiply(x=w2600, y=1000000000000.0) -> (x*y=→"Level 10 science price":dbl)
      n741 = Multiply(x=w2608, y=10000000000.0) -> (x*y=→"Level 8 science price":dbl)
      n742 = Multiply(x=w2604, y=100000000000.0) -> (x*y=→"Level 9 science price":dbl)
      n743 = Multiply(x=w2612, y=1000000000.0) -> (x*y=→"Level 7 science price":dbl)
      n744 = Compound Arithmetic op=ADD(w2698, w2697, w2650) -> (w2696:i32)
      n745 = Compound Arithmetic op=MULTIPLY(w2657, w2647, w2653) -> (w2656:dbl)
      n746 = Compound Arithmetic op=ADD(w2660) -> (w2659:dbl)
      n747 = local write "Non-land production multiplier"(w2659) -> ()
      n748 = local write "SP/EP multiplier"(w2656) -> ()
      n749 = local write "Trading level"(w2696) -> ()
    }
    n750 = local read "Build points"() -> (w1108:dbl)
    n751 = local read "Road invested points"() -> (w1448:dbl)
    n752 = local read "Governance\nlevel"() -> (w1162:i32)
    n753 = local read "School level"() -> (w1131:i32)
    n754 = local read "Build points"() -> (w1153:dbl)
    n755 = Subtract(x=600000 ("y"), y=w1104) -> (x-y=w1111:dbl)
    n756 = local read "Governance\nlevel"() -> (w1168:i32)
    n757 = local read "Temple\ninvested points"() -> (w526:dbl)
    n758 = local read "Barracks military bonus"() -> (w1327:dbl)
    n759 = local read "Harbor military mod"() -> (w540:dbl)
    n760 = local read "warrior c"() -> (w1993:dbl)
    n761 = local read "Harbor\ninvested points"() -> (w552:dbl)
    n762 = local read "Warrior b Gov mult"() -> (w1778:dbl)
    n763 = local read "Economics\nlevel"() -> (w1477:i32)
    n764 = local read "Construction\nlevel"() -> (w1416:i32)
    n765 = local read "Construction\nlevel"() -> (w1652:i32)
    n766 = Max & Min(x=w1111, y=0.0) -> (max(x,y)=w1106:dbl)  [unwired: 1 out]
    n767 = local read "Construction\nlevel"() -> (w1596:i32)
    n768 = Multiply(x=w1981, y=0.999) -> (x*y=w1980:dbl)
    n769 = Add(x=w2013, y=50.0) -> (x+y=w2011:dbl)
    n770 = Greater Or Equal?(x=w1159, y=2) -> (x >= y?=w1150:bool)
    n771 = Greater Or Equal?(x=w1108, y=w1106) -> (x >= y?=w1107:bool)
    n772 = local read "Build points"() -> (w1523:dbl)
    n773 = local read "Taxation\nlevel"() -> (w1466:dbl)
    n774 = local read "Economics\nlevel"() -> (w1461:i32)
    n775 = local read "Construction\nlevel"() -> (w496:i32)
    n776 = local read "Hut level"() -> (w1657:i32)
    n777 = local read "Hut level"() -> (w1599:i32)
    n778 = Greater Or Equal?(x=w1153, y=0) -> (x >= y?=w1151:bool)
    n779 = local read "Taxation\nlevel"() -> (w1482:dbl)
    n780 = Greater Or Equal?(x=w1136, y=3) -> (x >= y?=w1130:bool)
    n781 = local write "Food"(w1980) -> ()
    n782 = Not Equal?(x=w1154, y=w1148) -> (x != y?=w1156:bool)
    n783 = Greater Or Equal?(x=w1162, y=2) -> (x >= y?=w1163:bool)
    n784 = local read "Build points"() -> (w1444:dbl)
    n785 = local read "Construction\nlevel"() -> (w1393:i32)
    n786 = Subtract(x=30000 ("y"), y=w1521) -> (x-y=w1526:dbl)
    n787 = Reciprocal(x=w1993) -> (1/x=w387:dbl)
    n788 = Greater Or Equal?(x=w1168, y=2) -> (x >= y?=w1169:bool)
    n789 = local read "Road level"() -> (w1421:i32)
    n790 = Not Equal?(x=w1131, y=w1128) -> (x != y?=w1133:bool)
    n791 = local read "Road level"() -> (w1398:i32)
    n792 = Subtract(x=150000 ("y"), y=w1448) -> (x-y=w1441:dbl)
    n793 = local read "Build points"() -> (w1399:dbl)
    n794 = local read "Construction\nlevel"() -> (w475:i32)
    n795 = local read "Conquered\nland"() -> (w381:dbl)
    n796 = local read "warrior b"() -> (w1779:dbl)
    n797 = local read "Temple level"() -> (w500:i32)
    n798 = Power Of X(1:w2011, 2:w387) -> (0:w2010:dbl)
    n799 = local read "Gold dbl"() -> (w522:dbl)
    n800 = local read "Boat level"() -> (w582:i32)
    n801 = local read "Temple level"() -> (w479:i32)
    n802 = Subtract(x=10000 ("y"), y=w526) -> (x-y=w519:dbl)
    n803 = Compound Arithmetic op=AND(w1150, w1151, w1163) -> (w1149:bool)
    n804 = And(x="School\nlevel 0", y=w1149) -> (x .and. y?=w1157:bool)
    n805 = And(x=w1156, y=w1157) -> (x .and. y?=w1155:bool)
    n806 = case shown="True" w1155 {
      tunnel: w1148 -> [_ w2336]
      frame False {
      }
      frame True {
        n807 = local write "School engineer equivalent"(0.0 ("Hut dissent add mod")) -> ()
        n808 = local write "School level"(w2336) -> ()
        n809 = local write "School SP/EP multiplier"(1.0 ("Hut non-land prod mod")) -> ()
        n810 = local write "School dissent mod"(1.0 ("Hut non-land prod mod")) -> ()
        n811 = local write "School upkeep"(0.0 ("Hut non-land prod mod")) -> ()
      }
    }
    n812 = Max & Min(x=w1526, y=0.0) -> (max(x,y)=w1520:dbl)  [unwired: 1 out]
    n813 = local read "Build points"() -> (w556:dbl)
    n814 = local read "Gold dbl"() -> (w480:dbl)
    n815 = Power Of X(1:50.0 ("x"), 2:w387) -> (0:w386:dbl)
    n816 = Greater Or Equal?(x=w1652, y=1) -> (x >= y?=w1606:bool)
    n817 = Greater Or Equal?(x=w1523, y=w1520) -> (x >= y?=w1522:bool)
    n818 = And(x="Hut level 0", y=w1606) -> (x .and. y?=w1654:bool)
    n819 = local read "Harbor level"() -> (w578:i32)
    n820 = local read "Harbor level"() -> (w599:i32)
    n821 = Greater Or Equal?(x=w1596, y=1) -> (x >= y?=w1602:bool)
    n822 = Compound Arithmetic op=AND(w1130, w1107, w1169) -> (w1129:bool)
    n823 = And(x="School\nlevel 2", y=w1129) -> (x .and. y?=w1134:bool)
    n824 = And(x=w1133, y=w1134) -> (x .and. y?=w1132:bool)
    n825 = Max & Min(x=w1441, y=0.0) -> (max(x,y)=w1446:dbl)  [unwired: 1 out]
    n826 = Subtract(x=1500000 ("y"), y=w552) -> (x-y=w559:dbl)
    n827 = Greater Or Equal?(x=w1461, y=1) -> (x >= y?=w1459:bool)
    n828 = local read "Build points"() -> (w598:dbl)
    n829 = And(x="Taxes level 0", y=w1459) -> (x .and. y?=w1463:bool)
    n830 = Greater Or Equal?(x=w1444, y=w1446) -> (x >= y?=w1445:bool)
    n831 = local read "Boat level"() -> (w603:i32)
    n832 = Not Equal?(x=w1657, y=w1658) -> (x != y?=w1655:bool)
    n833 = And(x=w1655, y=w1654) -> (x .and. y?=w1656:bool)
    n834 = Greater Or Equal?(x=w1477, y=1) -> (x >= y?=w1456:bool)
    n835 = And(x="Taxes level 2", y=w1456) -> (x .and. y?=w1479:bool)
    n836 = Not Equal?(x=w1599, y=w1600) -> (x != y?=w1597:bool)
    n837 = Subtract(x=w2010, y=w386) -> (x-y=w1775:dbl)
    n838 = Compound Arithmetic op=AND(w1597, "Hut level 2", w1602, w1522) -> (w1598:bool)
    n839 = Quotient & Remainder(x=w1979, y=365.0) -> (x-y*floor(x/y)=→"Day":dbl, floor(x/y)=→"Year":dbl)
    n840 = Greater Or Equal?(x=w1416, y=1) -> (x >= y?=w1422:bool)
    n841 = Not Equal?(x=w1466, y=w1467) -> (x != y?=w1464:bool)
    n842 = And(x=w1464, y=w1463) -> (x .and. y?=w1465:bool)
    n843 = Max & Min(x=w519, y=0.0) -> (max(x,y)=w524:dbl)  [unwired: 1 out]
    n844 = Greater Or Equal?(x=w1393, y=1) -> (x >= y?=w1402:bool)
    n845 = Greater Or Equal?(x=w1399, y=0) -> (x >= y?=w1401:bool)
    n846 = local read "Military Modifier"() -> (w1777:dbl)
    n847 = local read "Governance\nlevel"() -> (w1166:i32)
    n848 = Greater Or Equal?(x=w522, y=w524) -> (x >= y?=w523:bool)
    n849 = local read "Gov populist\nbuildings mod"() -> (w1025:dbl)
    n850 = Not Equal?(x=w1482, y=w1483) -> (x != y?=w1480:bool)
    n851 = And(x=w1480, y=w1479) -> (x .and. y?=w1481:bool)
    n852 = case shown="True" w1598 {
      tunnel: w1600 -> [_ w2554]
      tunnel: w1521 -> [_ w2549]
      tunnel: w1520 -> [_ w2548]
      tunnel: w1025 -> [_ w2544]
      frame False {
      }
      frame True {
        n853 = local read "Build points"() -> (w2553:dbl)
        n854 = Multiply(x=w2544, y=0.2) -> (x*y=w2546:dbl)
        n855 = Add(x=w2548, y=w2549) -> (x+y=w2550:dbl)
        n856 = local write "Hut level"(w2554) -> ()
        n857 = Increment(x=w2546) -> (x+1=w2547:dbl)
        n858 = local write "Hut upkeep"(0.03 ("Hut dissent add mod")) -> ()
        n859 = local write "Hut non-land prod mod"(w2547) -> ()
        n860 = Subtract(x=w2553, y=w2548) -> (x-y=w2552:dbl)
        n861 = local write "Hut invested points"(w2550) -> ()
        n862 = local write "Hut dissent mod"(0.9 ("Hut dissent add mod")) -> ()
        n863 = local write "Build points"(w2552) -> ()
      }
    }
    n864 = Greater Or Equal?(x=w496, y=1) -> (x >= y?=w501:bool)
    n865 = Max & Min(x=w559, y=0.0) -> (max(x,y)=w554:dbl)  [unwired: 1 out]
    n866 = Not Equal?(x=w1421, y=w1424) -> (x != y?=w1419:bool)
    n867 = Greater Or Equal?(x=w475, y=1) -> (x >= y?=w483:bool)
    n868 = case shown="True" w1656 {
      tunnel: w1658 -> [_ w2585]
      frame False {
      }
      frame True {
        n869 = local write "Hut non-land prod mod"(1.0 ("Hut non-land prod mod")) -> ()
        n870 = local write "Hut dissent mod"(1.0 ("Hut dissent add mod")) -> ()
        n871 = local write "Hut level"(w2585) -> ()
        n872 = local write "Hut upkeep"(0.0 ("Hut dissent add mod")) -> ()
      }
    }
    n873 = Greater Or Equal?(x=w480, y=0) -> (x >= y?=w482:bool)
    n874 = Not Equal?(x=w1398, y=w1404) -> (x != y?=w1396:bool)
    n875 = Greater Or Equal?(x=w556, y=w554) -> (x >= y?=w555:bool)
    n876 = local read "Gov populist\nbuildings mod"() -> (w1024:dbl)
    n877 = case shown="True" w1132 {
      tunnel: w1128 -> [_ w2362]
      tunnel: w1106 -> [_ w2358]
      tunnel: w1104 -> [_ w2357]
      tunnel: w1024 -> [_ w2350]
      frame False {
      }
      frame True {
        n878 = Multiply(x=w2350, y=0.1) -> (x*y=w2353:dbl)
        n879 = Increment(x=w2353) -> (x+1=w2352:dbl)
        n880 = local read "Build points"() -> (w2361:dbl)
        n881 = Add(x=w2358, y=w2357) -> (x+y=w2359:dbl)
        n882 = local write "School engineer equivalent"(0.02 ("Hut dissent add mod")) -> ()
        n883 = local write "School level"(w2362) -> ()
        n884 = local write "School dissent mod"(0.96 ("Hut non-land prod mod")) -> ()
        n885 = local write "School SP/EP multiplier"(w2352) -> ()
        n886 = local write "School invested points"(w2359) -> ()
        n887 = local write "School upkeep"(0.003 ("Hut non-land prod mod")) -> ()
        n888 = Subtract(x=w2361, y=w2358) -> (x-y=w2360:dbl)
        n889 = local write "Build points"(w2360) -> ()
      }
    }
    n890 = Greater Or Equal?(x=w582, y=1) -> (x >= y?=w577:bool)
    n891 = case shown="True" w1465 {
      tunnel: w1467 -> [_ w2475]
      frame False {
      }
      frame True {
        n892 = local write "Taxation\nlevel"(w2475) -> ()
        n893 = local write "Taxes dissent mod"(0.0 ("Taxes dissent add mod")) -> ()
      }
    }
    n894 = case shown="True" w1481 {
      tunnel: w1483 -> [_ w2479]
      frame False {
      }
      frame True {
        n895 = local write "Taxation\nlevel"(w2479) -> ()
        n896 = local write "Taxes dissent mod"(8.0 ("Taxes dissent add mod")) -> ()
      }
    }
    n897 = Not Equal?(x=w500, y=w503) -> (x != y?=w498:bool)
    n898 = Greater Or Equal?(x=w603, y=1) -> (x >= y?=w595:bool)
    n899 = Greater Or Equal?(x=w598, y=0) -> (x >= y?=w596:bool)
    n900 = Not Equal?(x=w479, y=w485) -> (x != y?=w477:bool)
    n901 = Compound Arithmetic op=MULTIPLY(w1777, w540, w1327, w1778, w1779, 0.064789, 2.0 ("y"), w1775) -> (w1776:dbl)
    n902 = Add(x=w1776, y=w381) -> (x+y=w1992:dbl)
    n903 = local read "School invested points"() -> (w1105:dbl)
    n904 = And(x=w1422, y=w1445) -> (x .and. y?=w1423:bool)
    n905 = And(x="Road level 2", y=w1423) -> (x .and. y?=w1418:bool)
    n906 = And(x=w1419, y=w1418) -> (x .and. y?=w1420:bool)
    n907 = case shown="True" w1420 {
      tunnel: w1424 -> [_ w2464]
      tunnel: w1446 -> [_ w2457]
      tunnel: w1448 -> [_ w2456]
      frame False {
      }
      frame True {
        n908 = local read "Build points"() -> (w2463:dbl)
        n909 = Add(x=w2457, y=w2456) -> (x+y=w2459:dbl)
        n910 = local write "Road level"(w2464) -> ()
        n911 = local write "Road expansion bonus"(0.5 ("Hut dissent add mod")) -> ()
        n912 = local write "Road land prod mod"(1.2 ("Hut dissent add mod")) -> ()
        n913 = local write "Road invested points"(w2459) -> ()
        n914 = local write "Road upkeep"(0.06 ("Hut non-land prod mod")) -> ()
        n915 = Subtract(x=w2463, y=w2457) -> (x-y=w2462:dbl)
        n916 = local write "Build points"(w2462) -> ()
      }
    }
    n917 = And(x=w1402, y=w1401) -> (x .and. y?=w1403:bool)
    n918 = And(x="Road level 0", y=w1403) -> (x .and. y?=w1395:bool)
    n919 = And(x=w1396, y=w1395) -> (x .and. y?=w1397:bool)
    n920 = case shown="True" w1397 {
      tunnel: w1404 -> [_ w2446]
      frame False {
      }
      frame True {
        n921 = local write "Road level"(w2446) -> ()
        n922 = local write "Road expansion bonus"(0.0 ("Hut dissent add mod")) -> ()
        n923 = local write "Road land prod mod"(1.0 ("Hut dissent add mod")) -> ()
        n924 = local write "Road upkeep"(0.0 ("Hut non-land prod mod")) -> ()
      }
    }
    n925 = Not Equal?(x=w578, y=w575) -> (x != y?=w580:bool)
    n926 = Not Equal?(x=w599, y=w593) -> (x != y?=w601:bool)
    n927 = Greater Or Equal?(x=w1166, y=2) -> (x >= y?=w1165:bool)
    n928 = And(x=w501, y=w523) -> (x .and. y?=w502:bool)
    n929 = And(x="Temple\nlevel 2", y=w502) -> (x .and. y?=w497:bool)
    n930 = And(x=w498, y=w497) -> (x .and. y?=w499:bool)
    n931 = case shown="True" w499 {
      tunnel: w503 -> [_ w2125]
      tunnel: w524 -> [_ w2118]
      tunnel: w526 -> [_ w2117]
      frame False {
      }
      frame True {
        n932 = local read "Build points"() -> (w2124:dbl)
        n933 = Add(x=w2118, y=w2117) -> (x+y=w2120:dbl)
        n934 = local write "Temple level"(w2125) -> ()
        n935 = local write "Temple SP/EP multiplier"(1.0 ("Hut dissent add mod")) -> ()
        n936 = local write "Temple dissent mod"(0.94 ("Hut dissent add mod")) -> ()
        n937 = local write "Temple\ninvested points"(w2120) -> ()
        n938 = local write "Temple upkeep"(0.003 ("Hut non-land prod mod")) -> ()
        n939 = Subtract(x=w2124, y=w2118) -> (x-y=w2123:dbl)
        n940 = local write "Build points"(w2123) -> ()
      }
    }
    n941 = And(x=w483, y=w482) -> (x .and. y?=w484:bool)
    n942 = And(x="Temple\nlevel 0", y=w484) -> (x .and. y?=w476:bool)
    n943 = And(x=w477, y=w476) -> (x .and. y?=w478:bool)
    n944 = case shown="True" w478 {
      tunnel: w485 -> [_ w2107]
      frame False {
      }
      frame True {
        n945 = local write "Temple level"(w2107) -> ()
        n946 = local write "Temple SP/EP multiplier"(1.0 ("Hut dissent add mod")) -> ()
        n947 = local write "Temple dissent mod"(1.0 ("Hut dissent add mod")) -> ()
        n948 = local write "Temple upkeep"(0.0 ("Hut non-land prod mod")) -> ()
      }
    }
    n949 = local read "School invested points"() -> (w1097:dbl)
    n950 = And(x=w577, y=w555) -> (x .and. y?=w576:bool)
    n951 = And(x="Harbor level 2", y=w576) -> (x .and. y?=w581:bool)
    n952 = And(x=w580, y=w581) -> (x .and. y?=w579:bool)
    n953 = case shown="True" w579 {
      tunnel: w575 -> [_ w2156]
      tunnel: w554 -> [_ w2149]
      tunnel: w552 -> [_ w2148]
      frame False {
      }
      frame True {
        n954 = local read "Build points"() -> (w2155:dbl)
        n955 = Add(x=w2149, y=w2148) -> (x+y=w2151:dbl)
        n956 = local write "Harbor level"(w2156) -> ()
        n957 = local write "Harbor expansion bonus"(0.25 ("Hut dissent add mod")) -> ()
        n958 = local write "Harbor military mod"(1.2 ("Hut dissent add mod")) -> ()
        n959 = local write "Harbor\ninvested points"(w2151) -> ()
        n960 = local write "Harbor upkeep"(0.12 ("Hut non-land prod mod")) -> ()
        n961 = Subtract(x=w2155, y=w2149) -> (x-y=w2154:dbl)
        n962 = local write "Build points"(w2154) -> ()
      }
    }
    n963 = local read "Permanent\nland"() -> (w2004:dbl)
    n964 = And(x=w595, y=w596) -> (x .and. y?=w594:bool)
    n965 = And(x="Harbor level 0", y=w594) -> (x .and. y?=w602:bool)
    n966 = And(x=w601, y=w602) -> (x .and. y?=w600:bool)
    n967 = case shown="True" w600 {
      tunnel: w593 -> [_ w2138]
      frame False {
      }
      frame True {
        n968 = local write "Harbor level"(w2138) -> ()
        n969 = local write "Harbor expansion bonus"(0.0 ("Hut dissent add mod")) -> ()
        n970 = local write "Harbor military mod"(1.0 ("Hut dissent add mod")) -> ()
        n971 = local write "Harbor upkeep"(0.0 ("Hut non-land prod mod")) -> ()
      }
    }
    n972 = local read "People"() -> (w2006:i64)
    n973 = local read "Construction\nlevel"() -> (w1119:i32)
    n974 = local read "Road invested points"() -> (w1447:dbl)
    n975 = local read "Build points"() -> (w1114:dbl)
    n976 = local read "Hut invested points"() -> (w1527:dbl)
    n977 = local read "Harbor expansion bonus"() -> (w539:dbl)
    n978 = Subtract(x=200000 ("y"), y=w1105) -> (x-y=w1117:dbl)
    n979 = local read "Temple\ninvested points"() -> (w525:dbl)
    n980 = local read "Road expansion bonus"() -> (w1586:dbl)
    n981 = local read "Hut invested points"() -> (w1514:dbl)
    n982 = Divide(x=w2006, y=w2004) -> (x/y=w2005:dbl)
    n983 = Divide(x=w381, y=w2004) -> (x/y=w2003:dbl)
    n984 = local read "Construction\nlevel"() -> (w1139:i32)
    n985 = local read "School level"() -> (w1124:i32)
    n986 = local read "Road invested points"() -> (w1455:dbl)
    n987 = local read "Build points"() -> (w1103:dbl)
    n988 = local read "School level"() -> (w1144:i32)
    n989 = local read "Harbor\ninvested points"() -> (w553:dbl)
    n990 = local read "Temple\ninvested points"() -> (w533:dbl)
    n991 = local read "Economics\nlevel"() -> (w1490:i32)
    n992 = Subtract(x=2000000 ("y"), y=w1097) -> (x-y=w1100:dbl)
    n993 = Square(x=w2005) -> (x^2=w2002:dbl)
    n994 = Square(x=w2003) -> (x^2=w2001:dbl)
    n995 = Max & Min(x=w1117, y=0.0) -> (max(x,y)=w1112:dbl)  [unwired: 1 out]
    n996 = Greater Or Equal?(x=w1114, y=w1112) -> (x >= y?=w1113:bool)
    n997 = local read "Construction\nlevel"() -> (w1433:i32)
    n998 = local read "Harbor\ninvested points"() -> (w545:dbl)
    n999 = local read "Land conv mult"() -> (w384:dbl)
    n1000 = local read "Build points"() -> (w1438:dbl)
    n1001 = local read "Construction\nlevel"() -> (w1664:i32)
    n1002 = local read "Economics\nlevel"() -> (w1474:i32)
    n1003 = local read "Construction\nlevel"() -> (w511:i32)
    n1004 = local read "Construction\nlevel"() -> (w1593:i32)
    n1005 = Max & Min(x=w1100, y=0.0) -> (max(x,y)=w1098:dbl)  [unwired: 1 out]
    n1006 = Subtract(x=50000 ("y"), y=w1447) -> (x-y=w1435:dbl)
    n1007 = local read "Build points"() -> (w1660:dbl)
    n1008 = Greater Or Equal?(x=w1119, y=2) -> (x >= y?=w1125:bool)
    n1009 = Compound Arithmetic op=AND(w1125, w1113, w1165) -> (w1126:bool)
    n1010 = And(x="School\nlevel 1", y=w1126) -> (x .and. y?=w1121:bool)
    n1011 = local read "Taxation\nlevel"() -> (w1485:dbl)
    n1012 = local read "Taxation\nlevel"() -> (w1469:dbl)
    n1013 = local read "Hut level"() -> (w1661:i32)
    n1014 = Greater Or Equal?(x=w1103, y=w1098) -> (x >= y?=w1099:bool)
    n1015 = local read "Build points"() -> (w1519:dbl)
    n1016 = local read "Construction\nlevel"() -> (w1413:i32)
    n1017 = Greater Or Equal?(x=w1139, y=3) -> (x >= y?=w1145:bool)
    n1018 = local read "Gold dbl"() -> (w516:dbl)
    n1019 = local read "Build points"() -> (w1449:dbl)
    n1020 = Subtract(x=10000 ("y"), y=w1527) -> (x-y=w1529:dbl)
    n1021 = Not Equal?(x=w1124, y=w1127) -> (x != y?=w1122:bool)
    n1022 = And(x=w1122, y=w1121) -> (x .and. y?=w1123:bool)
    n1023 = local read "Road level"() -> (w1408:i32)
    n1024 = Multiply(x=w2002, y=w2001) -> (x*y=w1990:dbl)
    n1025 = Subtract(x=500 ("y"), y=w525) -> (x-y=w513:dbl)
    n1026 = local read "Hut level"() -> (w1590:i32)
    n1027 = Subtract(x=150000 ("y"), y=w1514) -> (x-y=w1516:dbl)
    n1028 = Not Equal?(x=w1144, y=w1147) -> (x != y?=w1142:bool)
    n1029 = local read "Build points"() -> (w562:dbl)
    n1030 = local read "Construction\nlevel"() -> (w493:i32)
    n1031 = local read "Road level"() -> (w1428:i32)
    n1032 = Subtract(x=500000 ("y"), y=w1455) -> (x-y=w1452:dbl)
    n1033 = local read "Boat level"() -> (w567:i32)
    n1034 = local read "Temple level"() -> (w489:i32)
    n1035 = Max & Min(x=w1435, y=0.0) -> (max(x,y)=w1440:dbl)  [unwired: 1 out]
    n1036 = Subtract(x=500000 ("y"), y=w553) -> (x-y=w565:dbl)
    n1037 = local read "Gold dbl"() -> (w527:dbl)
    n1038 = local read "Temple level"() -> (w507:i32)
    n1039 = Greater Or Equal?(x=w1438, y=w1440) -> (x >= y?=w1439:bool)
    n1040 = Subtract(x=500000 ("y"), y=w533) -> (x-y=w530:dbl)
    n1041 = Y-th Root of X(1:w1992, 2:4.0 ("y")) -> (0:w1989:dbl)
    n1042 = Multiply(x=w1990, y=w1989) -> (x*y=w1925:dbl)
    n1043 = Max & Min(x=w1529, y=0.0) -> (max(x,y)=w1528:dbl)  [unwired: 1 out]
    n1044 = local read "Governance\nlevel"() -> (w1170:i32)
    n1045 = local read "Build points"() -> (w551:dbl)
    n1046 = local read "Harbor level"() -> (w589:i32)
    n1047 = Max & Min(x=w513, y=0.0) -> (max(x,y)=w518:dbl)  [unwired: 1 out]
    n1048 = Max & Min(x=w1516, y=0.0) -> (max(x,y)=w1513:dbl)  [unwired: 1 out]
    n1049 = Greater Or Equal?(x=w1660, y=w1528) -> (x >= y?=w1603:bool)
    n1050 = Greater Or Equal?(x=w1664, y=1) -> (x >= y?=w1604:bool)
    n1051 = local read "Harbor level"() -> (w571:i32)
    n1052 = Greater Or Equal?(x=w516, y=w518) -> (x >= y?=w517:bool)
    n1053 = Greater Or Equal?(x=w1519, y=w1513) -> (x >= y?=w1515:bool)
    n1054 = Max & Min(x=w1452, y=0.0) -> (max(x,y)=w1454:dbl)  [unwired: 1 out]
    n1055 = local read "Boat level"() -> (w585:i32)
    n1056 = Greater Or Equal?(x=w1593, y=1) -> (x >= y?=w1587:bool)
    n1057 = Subtract(x=5000000 ("y"), y=w545) -> (x-y=w548:dbl)
    n1058 = Greater Or Equal?(x=w1490, y=1) -> (x >= y?=w1458:bool)
    n1059 = Greater Or Equal?(x=w1474, y=1) -> (x >= y?=w1457:bool)
    n1060 = And(x="Taxes level 1", y=w1458) -> (x .and. y?=w1488:bool)
    n1061 = And(x="Taxes level 3", y=w1457) -> (x .and. y?=w1472:bool)
    n1062 = Greater Or Equal?(x=w1449, y=w1454) -> (x >= y?=w1453:bool)
    n1063 = Not Equal?(x=w1661, y=w1659) -> (x != y?=w1663:bool)
    n1064 = Increment(x=w1586) -> (x+1=w1585:dbl)
    n1065 = Max & Min(x=w565, y=0.0) -> (max(x,y)=w560:dbl)  [unwired: 1 out]
    n1066 = Compound Arithmetic op=AND(w1663, "Hut level 1", w1604, w1603) -> (w1662:bool)
    n1067 = Greater Or Equal?(x=w1413, y=1) -> (x >= y?=w1407:bool)
    n1068 = Increment(x=w539) -> (x+1=w538:dbl)
    n1069 = Compound Arithmetic op=MULTIPLY(w538, w1585, w384, w1925, 1e-05 ("y")) -> (w382:dbl)
    "Land conversion rate" <- w382
    n1070 = Add(x=w1713, y=w382) -> (x+y=w1996:dbl)
    n1071 = local write "Permanent\nland"(w1996) -> ()
    n1072 = Not Equal?(x=w1590, y=w1589) -> (x != y?=w1592:bool)
    n1073 = Compound Arithmetic op=AND(w1592, "Hut level 3", w1587, w1515) -> (w1591:bool)
    n1074 = Greater Or Equal?(x=w562, y=w560) -> (x >= y?=w561:bool)
    n1075 = Not Equal?(x=w1485, y=w1484) -> (x != y?=w1487:bool)
    n1076 = And(x=w1487, y=w1488) -> (x .and. y?=w1486:bool)
    n1077 = Not Equal?(x=w1469, y=w1468) -> (x != y?=w1471:bool)
    n1078 = And(x=w1471, y=w1472) -> (x .and. y?=w1470:bool)
    n1079 = Max & Min(x=w530, y=0.0) -> (max(x,y)=w532:dbl)  [unwired: 1 out]
    n1080 = Greater Or Equal?(x=w1433, y=1) -> (x >= y?=w1427:bool)
    n1081 = And(x=w1427, y=w1439) -> (x .and. y?=w1426:bool)
    n1082 = And(x="Road level 1", y=w1426) -> (x .and. y?=w1431:bool)
    n1083 = Greater Or Equal?(x=w527, y=w532) -> (x >= y?=w531:bool)
    n1084 = case shown="True" w1470 {
      tunnel: w1468 -> [_ w2477]
      frame False {
      }
      frame True {
        n1085 = local write "Taxation\nlevel"(w2477) -> ()
        n1086 = local write "Taxes dissent mod"(15.0 ("Taxes dissent add mod")) -> ()
      }
    }
    n1087 = case shown="True" w1123 {
      tunnel: w1127 -> [_ w2375]
      tunnel: w1105 -> [_ w2372]
      tunnel: w1112 -> [_ w2370]
      tunnel: w1024 -> [_ w2363]
      frame False {
      }
      frame True {
        n1088 = Multiply(x=w2363, y=0.05) -> (x*y=w2365:dbl)
        n1089 = Increment(x=w2365) -> (x+1=w2366:dbl)
        n1090 = local read "Build points"() -> (w2374:dbl)
        n1091 = Add(x=w2370, y=w2372) -> (x+y=w2371:dbl)
        n1092 = local write "School level"(w2375) -> ()
        n1093 = local write "School engineer equivalent"(0.01 ("Hut dissent add mod")) -> ()
        n1094 = local write "School SP/EP multiplier"(w2366) -> ()
        n1095 = local write "School invested points"(w2371) -> ()
        n1096 = local write "School dissent mod"(0.98 ("Hut non-land prod mod")) -> ()
        n1097 = Subtract(x=w2374, y=w2370) -> (x-y=w2373:dbl)
        n1098 = local write "School upkeep"(0.001 ("Hut non-land prod mod")) -> ()
        n1099 = local write "Build points"(w2373) -> ()
      }
    }
    n1100 = Not Equal?(x=w1408, y=w1405) -> (x != y?=w1410:bool)
    n1101 = Greater Or Equal?(x=w493, y=1) -> (x >= y?=w488:bool)
    n1102 = And(x=w1407, y=w1453) -> (x .and. y?=w1406:bool)
    n1103 = And(x="Road level 3", y=w1406) -> (x .and. y?=w1411:bool)
    n1104 = And(x=w1410, y=w1411) -> (x .and. y?=w1409:bool)
    n1105 = case shown="True" w1662 {
      tunnel: w1659 -> [_ w2597]
      tunnel: w1528 -> [_ w2592]
      tunnel: w1527 -> [_ w2593]
      tunnel: w1025 -> [_ w2587]
      frame False {
      }
      frame True {
        n1106 = local read "Build points"() -> (w2596:dbl)
        n1107 = Multiply(x=0.1, y=w2587) -> (x*y=w2588:dbl)
        n1108 = local write "Hut level"(w2597) -> ()
        n1109 = Add(x=w2592, y=w2593) -> (x+y=w2591:dbl)
        n1110 = Increment(x=w2588) -> (x+1=w2590:dbl)
        n1111 = local write "Hut upkeep"(0.01 ("Hut dissent add mod")) -> ()
        n1112 = Subtract(x=w2596, y=w2592) -> (x-y=w2595:dbl)
        n1113 = local write "Hut non-land prod mod"(w2590) -> ()
        n1114 = local write "Build points"(w2595) -> ()
        n1115 = local write "Hut invested points"(w2591) -> ()
        n1116 = local write "Hut dissent mod"(0.95 ("Hut dissent add mod")) -> ()
      }
    }
    n1117 = Subtract(x=w1992, y=w382) -> (x-y=w1897:dbl)
    n1118 = case shown="True" w1591 {
      tunnel: w1589 -> [_ w2542]
      tunnel: w1514 -> [_ w2537]
      tunnel: w1513 -> [_ w2536]
      tunnel: w1025 -> [_ w2532]
      frame False {
      }
      frame True {
        n1119 = Multiply(x=w2532, y=0.3) -> (x*y=w2534:dbl)
        n1120 = Increment(x=w2534) -> (x+1=w2535:dbl)
        n1121 = local read "Build points"() -> (w2541:dbl)
        n1122 = Add(x=w2536, y=w2537) -> (x+y=w2538:dbl)
        n1123 = local write "Hut non-land prod mod"(w2535) -> ()
        n1124 = local write "Hut level"(w2542) -> ()
        n1125 = local write "Hut upkeep"(0.15 ("Hut dissent add mod")) -> ()
        n1126 = Subtract(x=w2541, y=w2536) -> (x-y=w2540:dbl)
        n1127 = local write "Hut invested points"(w2538) -> ()
        n1128 = local write "Build points"(w2540) -> ()
        n1129 = local write "Hut dissent mod"(0.85 ("Hut dissent add mod")) -> ()
      }
    }
    n1130 = Max & Min(x=w548, y=0.0) -> (max(x,y)=w546:dbl)  [unwired: 1 out]
    n1131 = Not Equal?(x=w1428, y=w1425) -> (x != y?=w1430:bool)
    n1132 = And(x=w1430, y=w1431) -> (x .and. y?=w1429:bool)
    n1133 = Greater Or Equal?(x=w511, y=1) -> (x >= y?=w506:bool)
    n1134 = And(x=w506, y=w517) -> (x .and. y?=w505:bool)
    n1135 = And(x="Temple\nlevel 1", y=w505) -> (x .and. y?=w510:bool)
    n1136 = Greater Or Equal?(x=w551, y=w546) -> (x >= y?=w547:bool)
    n1137 = case shown="True" w1486 {
      tunnel: w1484 -> [_ w2481]
      frame False {
      }
      frame True {
        n1138 = local write "Taxation\nlevel"(w2481) -> ()
        n1139 = local write "Taxes dissent mod"(3.0 ("Taxes dissent add mod")) -> ()
      }
    }
    n1140 = Not Equal?(x=w489, y=w486) -> (x != y?=w491:bool)
    n1141 = Greater Or Equal?(x=w585, y=1) -> (x >= y?=w590:bool)
    n1142 = And(x=w488, y=w531) -> (x .and. y?=w487:bool)
    n1143 = And(x="Temple\nlevel 3", y=w487) -> (x .and. y?=w492:bool)
    n1144 = And(x=w491, y=w492) -> (x .and. y?=w490:bool)
    n1145 = Not Equal?(x=w507, y=w504) -> (x != y?=w509:bool)
    n1146 = And(x=w509, y=w510) -> (x .and. y?=w508:bool)
    n1147 = Greater Or Equal?(x=w1170, y=2) -> (x >= y?=w1172:bool)
    n1148 = Compound Arithmetic op=AND(w1145, w1099, w1172) -> (w1146:bool)
    n1149 = And(x="School\nlevel 3", y=w1146) -> (x .and. y?=w1141:bool)
    n1150 = And(x=w1142, y=w1141) -> (x .and. y?=w1143:bool)
    n1151 = case shown="True" w1143 {
      tunnel: w1147 -> [_ w2349]
      tunnel: w1098 -> [_ w2345]
      tunnel: w1097 -> [_ w2344]
      tunnel: w1024 -> [_ w2337]
      frame False {
      }
      frame True {
        n1152 = Multiply(x=w2337, y=0.15) -> (x*y=w2340:dbl)
        n1153 = local read "Build points"() -> (w2348:dbl)
        n1154 = Add(x=w2345, y=w2344) -> (x+y=w2346:dbl)
        n1155 = Increment(x=w2340) -> (x+1=w2339:dbl)
        n1156 = local write "School level"(w2349) -> ()
        n1157 = local write "School engineer equivalent"(0.03 ("Hut dissent add mod")) -> ()
        n1158 = local write "School invested points"(w2346) -> ()
        n1159 = local write "School SP/EP multiplier"(w2339) -> ()
        n1160 = local write "School dissent mod"(0.94 ("Hut non-land prod mod")) -> ()
        n1161 = Subtract(x=w2348, y=w2345) -> (x-y=w2347:dbl)
        n1162 = local write "School upkeep"(0.01 ("Hut non-land prod mod")) -> ()
        n1163 = local write "Build points"(w2347) -> ()
      }
    }
    n1164 = Greater Or Equal?(x=w567, y=1) -> (x >= y?=w572:bool)
    n1165 = And(x=w572, y=w561) -> (x .and. y?=w573:bool)
    n1166 = case shown="True" w1409 {
      tunnel: w1405 -> [_ w2455]
      tunnel: w1454 -> [_ w2448]
      tunnel: w1455 -> [_ w2447]
      frame False {
      }
      frame True {
        n1167 = local read "Build points"() -> (w2454:dbl)
        n1168 = Add(x=w2448, y=w2447) -> (x+y=w2449:dbl)
        n1169 = local write "Road level"(w2455) -> ()
        n1170 = local write "Road expansion bonus"(1.0 ("Hut dissent add mod")) -> ()
        n1171 = local write "Road land prod mod"(1.3 ("Hut dissent add mod")) -> ()
        n1172 = local write "Road invested points"(w2449) -> ()
        n1173 = local write "Road upkeep"(0.2 ("Hut non-land prod mod")) -> ()
        n1174 = Subtract(x=w2454, y=w2448) -> (x-y=w2453:dbl)
        n1175 = local write "Build points"(w2453) -> ()
      }
    }
    n1176 = And(x="Harbor level 1", y=w573) -> (x .and. y?=w568:bool)
    n1177 = case shown="True" w1429 {
      tunnel: w1425 -> [_ w2473]
      tunnel: w1447 -> [_ w2467]
      tunnel: w1440 -> [_ w2465]
      frame False {
      }
      frame True {
        n1178 = local read "Build points"() -> (w2472:dbl)
        n1179 = Add(x=w2465, y=w2467) -> (x+y=w2466:dbl)
        n1180 = local write "Road level"(w2473) -> ()
        n1181 = local write "Road expansion bonus"(0.2 ("Hut dissent add mod")) -> ()
        n1182 = local write "Road land prod mod"(1.1 ("Hut dissent add mod")) -> ()
        n1183 = local write "Road invested points"(w2466) -> ()
        n1184 = local write "Road upkeep"(0.02 ("Hut non-land prod mod")) -> ()
        n1185 = Subtract(x=w2472, y=w2465) -> (x-y=w2471:dbl)
        n1186 = local write "Build points"(w2471) -> ()
      }
    }
    n1187 = Not Equal?(x=w589, y=w592) -> (x != y?=w587:bool)
    n1188 = And(x=w590, y=w547) -> (x .and. y?=w591:bool)
    n1189 = And(x="Harbor level 3", y=w591) -> (x .and. y?=w586:bool)
    n1190 = And(x=w587, y=w586) -> (x .and. y?=w588:bool)
    n1191 = case shown="True" w490 {
      tunnel: w486 -> [_ w2116]
      tunnel: w532 -> [_ w2109]
      tunnel: w533 -> [_ w2108]
      frame False {
      }
      frame True {
        n1192 = local read "Build points"() -> (w2115:dbl)
        n1193 = Add(x=w2109, y=w2108) -> (x+y=w2110:dbl)
        n1194 = local write "Temple level"(w2116) -> ()
        n1195 = local write "Temple SP/EP multiplier"(1.0 ("Hut dissent add mod")) -> ()
        n1196 = local write "Temple dissent mod"(0.91 ("Hut dissent add mod")) -> ()
        n1197 = local write "Temple\ninvested points"(w2110) -> ()
        n1198 = local write "Temple upkeep"(0.01 ("Hut non-land prod mod")) -> ()
        n1199 = Subtract(x=w2115, y=w2109) -> (x-y=w2114:dbl)
        n1200 = local write "Build points"(w2114) -> ()
      }
    }
    n1201 = Not Equal?(x=w571, y=w574) -> (x != y?=w569:bool)
    n1202 = And(x=w569, y=w568) -> (x .and. y?=w570:bool)
    n1203 = case shown="True" w508 {
      tunnel: w504 -> [_ w2134]
      tunnel: w525 -> [_ w2128]
      tunnel: w518 -> [_ w2126]
      frame False {
      }
      frame True {
        n1204 = local read "Build points"() -> (w2133:dbl)
        n1205 = Add(x=w2126, y=w2128) -> (x+y=w2127:dbl)
        n1206 = local write "Temple level"(w2134) -> ()
        n1207 = local write "Temple SP/EP multiplier"(1.0 ("Hut dissent add mod")) -> ()
        n1208 = local write "Temple\ninvested points"(w2127) -> ()
        n1209 = local write "Temple dissent mod"(0.97 ("Hut dissent add mod")) -> ()
        n1210 = local write "Temple upkeep"(0.001 ("Hut non-land prod mod")) -> ()
        n1211 = Subtract(x=w2133, y=w2126) -> (x-y=w2132:dbl)
        n1212 = local write "Build points"(w2132) -> ()
      }
    }
    n1213 = Multiply(x=w1897, y=0.01) -> (x*y=w1896:dbl)
    n1214 = case shown="True" w588 {
      tunnel: w592 -> [_ w2147]
      tunnel: w546 -> [_ w2140]
      tunnel: w545 -> [_ w2139]
      frame False {
      }
      frame True {
        n1215 = local read "Build points"() -> (w2146:dbl)
        n1216 = Add(x=w2140, y=w2139) -> (x+y=w2141:dbl)
        n1217 = local write "Harbor level"(w2147) -> ()
        n1218 = local write "Harbor expansion bonus"(0.5 ("Hut dissent add mod")) -> ()
        n1219 = local write "Harbor military mod"(1.3 ("Hut dissent add mod")) -> ()
        n1220 = local write "Harbor\ninvested points"(w2141) -> ()
        n1221 = local write "Harbor upkeep"(0.4 ("Hut non-land prod mod")) -> ()
        n1222 = Subtract(x=w2146, y=w2140) -> (x-y=w2145:dbl)
        n1223 = local write "Build points"(w2145) -> ()
      }
    }
    n1224 = Multiply(x=0.99, y=w1897) -> (x*y=w1995:dbl)
    n1225 = case shown="True" w570 {
      tunnel: w574 -> [_ w2165]
      tunnel: w553 -> [_ w2159]
      tunnel: w560 -> [_ w2157]
      frame False {
      }
      frame True {
        n1226 = local read "Build points"() -> (w2164:dbl)
        n1227 = Add(x=w2157, y=w2159) -> (x+y=w2158:dbl)
        n1228 = local write "Harbor level"(w2165) -> ()
        n1229 = local write "Harbor expansion bonus"(0.1 ("Hut dissent add mod")) -> ()
        n1230 = local write "Harbor military mod"(1.1 ("Hut dissent add mod")) -> ()
        n1231 = local write "Harbor\ninvested points"(w2158) -> ()
        n1232 = local write "Harbor upkeep"(0.04 ("Hut non-land prod mod")) -> ()
        n1233 = Subtract(x=w2164, y=w2157) -> (x-y=w2163:dbl)
        n1234 = local write "Build points"(w2163) -> ()
      }
    }
    n1235 = Add(x=w1896, y=w382) -> (x+y=w1895:dbl)
    n1236 = Subtract(x=w1776, y=w1895) -> (x-y=w1894:dbl)
    n1237 = local write "Temp land change/s"(w1894) -> ()
    n1238 = local write "Conquered\nland"(w1995) -> ()
    n1239 = local read "University\ninvested points"() -> (w1015:dbl)
    n1240 = local read "Military\nScience level"() -> (w215:i32)
    n1241 = local read "Economics\nlevel"() -> (w1258:i32)
    n1242 = local read "Military\nScience level"() -> (w218:i32)
    n1243 = local read "Physics level"() -> (w231:i32)
    n1244 = local read "Military\nScience level"() -> (w310:i32)
    n1245 = local read "Taxation\nlevel"() -> (w1263:dbl)
    n1246 = local read "Physics level"() -> (w269:i32)
    n1247 = local read "Construction\nlevel"() -> (w983:i32)
    n1248 = local read "Physics level"() -> (w202:i32)
    n1249 = local read "Physics level"() -> (w150:i32)
    n1250 = local read "Construction\nlevel"() -> (w960:i32)
    n1251 = local read "University level"() -> (w965:i32)
    n1252 = local read "Build points"() -> (w1011:dbl)
    n1253 = local read "University level"() -> (w988:i32)
    n1254 = local read "Governance\nlevel"() -> (w957:i32)
    n1255 = local read "Physics level"() -> (w176:i32)
    n1256 = local read "Build points"() -> (w966:dbl)
    n1257 = local read "Physics level"() -> (w173:i32)
    n1258 = local read "Military\nScience level"() -> (w1770:i32)
    n1259 = local read "Physics level"() -> (w199:i32)
    n1260 = Subtract(x=600000 ("y"), y=w1015) -> (x-y=w1008:dbl)
    n1261 = local read "Governance\nlevel"() -> (w951:i32)
    n1262 = local read "Vehicle\nlevel"() -> (w160:i32)
    n1263 = local read "Electronics\nlevel"() -> (w221:i32)
    n1264 = local read "Electronics\nlevel"() -> (w212:i32)
    n1265 = local read "Electronics\nlevel"() -> (w295:i32)
    n1266 = Greater Or Equal?(x=w1258, y=1) -> (x >= y?=w1265:bool)
    n1267 = And(x="Taxes level 4", y=w1265) -> (x .and. y?=w1260:bool)
    n1268 = local read "Vehicle\nlevel"() -> (w186:i32)
    n1269 = local read "Vehicle\nlevel"() -> (w163:i32)
    n1270 = local read "Vehicle\nlevel"() -> (w189:i32)
    n1271 = Not Equal?(x=w1263, y=w1264) -> (x != y?=w1261:bool)
    n1272 = And(x=w1261, y=w1260) -> (x .and. y?=w1262:bool)
    n1273 = local read "Biology\nlevel"() -> (w1694:i32)
    n1274 = local read "Physics level"() -> (w1736:i32)
    n1275 = Greater Or Equal?(x=w231, y=5.0) -> (x >= y?=w232:bool)
    n1276 = Max & Min(x=w1008, y=0.0) -> (max(x,y)=w1013:dbl)  [unwired: 1 out]
    n1277 = local read "Physics level"() -> (w317:i32)
    n1278 = Greater Or Equal?(x=w202, y=5.0) -> (x >= y?=w201:bool)
    n1279 = Greater Or Equal?(x=w1011, y=w1013) -> (x >= y?=w1012:bool)
    n1280 = Greater Or Equal?(x=w269, y=5.0) -> (x >= y?=w268:bool)
    n1281 = Greater Or Equal?(x=w218, y=3.0) -> (x >= y?=w217:bool)
    n1282 = Greater Or Equal?(x=w960, y=2) -> (x >= y?=w969:bool)
    n1283 = Greater Or Equal?(x=w966, y=0) -> (x >= y?=w968:bool)
    n1284 = case shown="True" w1262 {
      tunnel: w1264 -> [_ w2401]
      frame False {
      }
      frame True {
        n1285 = local write "Taxation\nlevel"(w2401) -> ()
        n1286 = local write "Taxes dissent mod"(25.0 ("Taxes dissent add mod")) -> ()
      }
    }
    n1287 = Greater Or Equal?(x=w150, y=5.0) -> (x >= y?=w149:bool)
    n1288 = Greater Or Equal?(x=w983, y=3) -> (x >= y?=w989:bool)
    n1289 = Greater Or Equal?(x=w957, y=2) -> (x >= y?=w956:bool)
    n1290 = Greater Or Equal?(x=w215, y=3.0) -> (x >= y?=w216:bool)
    n1291 = Greater Or Equal?(x=w310, y=3.0) -> (x >= y?=w311:bool)
    n1292 = Not Equal?(x=w965, y=w971) -> (x != y?=w963:bool)
    n1293 = Greater Or Equal?(x=w951, y=2) -> (x >= y?=w950:bool)
    n1294 = Greater Or Equal?(x=w176, y=5.0) -> (x >= y?=w175:bool)
    n1295 = Not Equal?(x=w988, y=w991) -> (x != y?=w986:bool)
    n1296 = Greater Or Equal?(x=w173, y=5.0) -> (x >= y?=w174:bool)
    n1297 = local read "EP"() -> (w158:dbl)
    n1298 = Greater Or Equal?(x=w199, y=5.0) -> (x >= y?=w200:bool)
    n1299 = local read "EP"() -> (w223:dbl)
    n1300 = local read "EP"() -> (w184:dbl)
    n1301 = local read "Governance\nlevel"() -> (w1923:i32)
    n1302 = local read "EP"() -> (w165:dbl)
    n1303 = local read "# of level 10 sciences"() -> (w1553:i32)
    n1304 = local read "EP"() -> (w210:dbl)
    n1305 = local read "EP"() -> (w191:dbl)
    n1306 = local read "# of level 5 sciences"() -> (w1558:i32)
    n1307 = local read "# of level 6 sciences"() -> (w1557:i32)
    n1308 = local read "# of level 7 sciences"() -> (w1556:i32)
    n1309 = local read "# of level 8 sciences"() -> (w1555:i32)
    n1310 = local read "# of level 9 sciences"() -> (w1554:i32)
    n1311 = local read "EP"() -> (w293:dbl)
    n1312 = local read "# of level 1 sciences"() -> (w1562:i32)
    n1313 = local read "# of level 2 sciences"() -> (w1561:i32)
    n1314 = local read "# of level 3 sciences"() -> (w1560:i32)
    n1315 = local read "# of level 4 sciences"() -> (w1559:i32)
    n1316 = local read "Governance\nlevel"() -> (w1910:i32)
    n1317 = Greater Or Equal?(x=w158, y=w157) -> (x >= y?=w153:bool)
    n1318 = Compound Arithmetic op=AND(w969, w968, w956) -> (w970:bool)
    n1319 = And(x="University\nlevel 0", y=w970) -> (x .and. y?=w962:bool)
    n1320 = And(x=w963, y=w962) -> (x .and. y?=w964:bool)
    n1321 = case shown="True" w964 {
      tunnel: w971 -> [_ w2273]
      frame False {
      }
      frame True {
        n1322 = local write "University scientist equivalent"(0.0 ("Hut dissent add mod")) -> ()
        n1323 = local write "University level"(w2273) -> ()
        n1324 = local write "University SP multiplier"(1.0 ("Hut non-land prod mod")) -> ()
        n1325 = local write "University dissent mod"(1.0 ("Hut non-land prod mod")) -> ()
        n1326 = local write "University upkeep"(0.0 ("Hut non-land prod mod")) -> ()
      }
    }
    n1327 = Subtract(x=w158, y=w157) -> (x-y=w156:dbl)
    n1328 = Equal?(x=w160, y=0.0) -> (x = y?=w155:bool)
    n1329 = Compound Arithmetic op=AND(w989, w1012, w950) -> (w990:bool)
    n1330 = And(x="University\nlevel 2", y=w990) -> (x .and. y?=w985:bool)
    n1331 = And(x=w986, y=w985) -> (x .and. y?=w987:bool)
    n1332 = Compound Arithmetic op=AND(w155, "Rocket", w149, w153) -> (w152:bool)
    n1333 = Increment(x=w160) -> (x+1=w159:i32)
    n1334 = Greater Or Equal?(x=w1770, y=3.0) -> (x >= y?=w1774:bool)
    n1335 = Greater Or Equal?(x=w223, y=w224) -> (x >= y?=w228:bool)
    n1336 = Subtract(x=w223, y=w224) -> (x-y=w225:dbl)
    n1337 = Equal?(x=w221, y=1.0) -> (x = y?=w226:bool)
    n1338 = Compound Arithmetic op=AND(w226, "Radio", w217, w232, w228) -> (w229:bool)
    n1339 = Greater Or Equal?(x=w184, y=w183) -> (x >= y?=w179:bool)
    n1340 = Increment(x=w221) -> (x+1=w222:i32)
    n1341 = Greater Or Equal?(x=w165, y=w166) -> (x >= y?=w170:bool)
    n1342 = Subtract(x=w184, y=w183) -> (x-y=w182:dbl)
    n1343 = local read "Government"() -> (w1918:string)
    n1344 = Greater Or Equal?(x=w210, y=w209) -> (x >= y?=w205:bool)
    n1345 = Equal?(x=w186, y=0.0) -> (x = y?=w181:bool)
    n1346 = Subtract(x=w165, y=w166) -> (x-y=w167:dbl)
    n1347 = Greater Or Equal?(x=w191, y=w192) -> (x >= y?=w196:bool)
    n1348 = Compound Arithmetic op=AND(w181, "Internal combustion engine (cars)", w175, w179) -> (w178:bool)
    n1349 = Equal?(x=w163, y=0.0) -> (x = y?=w168:bool)
    n1350 = Greater Or Equal?(x=w293, y=w292) -> (x >= y?=w288:bool)
    n1351 = Subtract(x=w210, y=w209) -> (x-y=w208:dbl)
    n1352 = Increment(x=w186) -> (x+1=w185:i32)
    n1353 = Compound Arithmetic op=AND(w168, "Aircraft", w174, w170) -> (w171:bool)
    n1354 = local read "Government"() -> (w1905:string)
    n1355 = Subtract(x=w191, y=w192) -> (x-y=w193:dbl)
    n1356 = Equal?(x=w212, y=2.0) -> (x = y?=w207:bool)
    n1357 = Increment(x=w163) -> (x+1=w164:i32)
    n1358 = Subtract(x=w293, y=w292) -> (x-y=w291:dbl)
    n1359 = Compound Arithmetic op=AND(w207, "Computer", w216, w201, w205) -> (w204:bool)
    n1360 = Equal?(x=w189, y=0.0) -> (x = y?=w194:bool)
    n1361 = Compound Arithmetic op=AND(w194, "Steam Powered Train", w200, w196) -> (w197:bool)
    n1362 = And(x="Bow 1", y=w1774) -> (x .and. y?=w1772:bool)
    n1363 = Equal?(x=w295, y=0.0) -> (x = y?=w290:bool)
    n1364 = Increment(x=w212) -> (x+1=w211:i32)
    n1365 = local read "Farming level"() -> (w1701:i32)
    n1366 = Compound Arithmetic op=AND(w290, "Light bulb", w311, w268, w288) -> (w287:bool)
    n1367 = Increment(x=w189) -> (x+1=w190:i32)
    n1368 = Increment(x=w295) -> (x+1=w294:i32)
    n1369 = Greater Or Equal?(x=w1694, y=3.0) -> (x >= y?=w1693:bool)
    n1370 = Greater Or Equal?(x=w1736, y=3.0) -> (x >= y?=w1737:bool)
    n1371 = local read "Governance\nlevel"() -> (w953:i32)
    n1372 = local read "Bow level"() -> (w1787:i32)
    n1373 = local read "Boat level"() -> (w1729:i32)
    n1374 = local read "Governance\nlevel"() -> (w1945:i32)
    n1375 = Greater Or Equal?(x=w317, y=3.0) -> (x >= y?=w316:bool)
    n1376 = local read "Boat level"() -> (w324:i32)
    n1377 = local read "Government"() -> (w1932:string)
    n1378 = local read "Spear level"() -> (w1966:i32)
    n1379 = local read "SP"() -> (w1917:dbl)
    n1380 = local read "SP"() -> (w1904:dbl)
    n1381 = case shown="True" w152 {
      tunnel: w159 -> [_ w2022]
      tunnel: w156 -> [_ w2021]
      frame False {
      }
      frame True {
        n1382 = local write "EP"(w2021) -> ()
        n1383 = local write "Vehicle\nlevel"(w2022) -> ()
      }
    }
    n1384 = local read "Net level"() -> (w1959:i32)
    n1385 = case shown="True" w229 {
      tunnel: w222 -> [_ w2032]
      tunnel: w225 -> [_ w2031]
      frame False {
      }
      frame True {
        n1386 = local write "EP"(w2031) -> ()
        n1387 = local write "Electronics\nlevel"(w2032) -> ()
      }
    }
    n1388 = local read "EP"() -> (w1789:dbl)
    n1389 = local read "EP"() -> (w1699:dbl)
    n1390 = local read "EP"() -> (w1731:dbl)
    n1391 = local read "SP"() -> (w1931:dbl)
    n1392 = case shown="True" w178 {
      tunnel: w185 -> [_ w2026]
      tunnel: w182 -> [_ w2025]
      frame False {
      }
      frame True {
        n1393 = local write "EP"(w2025) -> ()
        n1394 = local write "Vehicle\nlevel"(w2026) -> ()
      }
    }
    n1395 = local read "EP"() -> (w322:dbl)
    n1396 = case shown="True" w171 {
      tunnel: w164 -> [_ w2024]
      tunnel: w167 -> [_ w2023]
      frame False {
      }
      frame True {
        n1397 = local write "EP"(w2023) -> ()
        n1398 = local write "Vehicle\nlevel"(w2024) -> ()
      }
    }
    n1399 = local read "EP"() -> (w1973:dbl)
    n1400 = local read "Gov elitist\nbuildings mod"() -> (w1023:dbl)
    n1401 = case shown="True" w987 {
      tunnel: w991 -> [_ w2299]
      tunnel: w1013 -> [_ w2295]
      tunnel: w1015 -> [_ w2294]
      tunnel: w1023 -> [_ w2287]
      frame False {
      }
      frame True {
        n1402 = Multiply(x=w2287, y=0.3) -> (x*y=w2290:dbl)
        n1403 = Increment(x=w2290) -> (x+1=w2289:dbl)
        n1404 = local read "Build points"() -> (w2298:dbl)
        n1405 = Add(x=w2295, y=w2294) -> (x+y=w2296:dbl)
        n1406 = local write "University scientist equivalent"(0.04 ("Hut dissent add mod")) -> ()
        n1407 = local write "University level"(w2299) -> ()
        n1408 = local write "University dissent mod"(0.96 ("Hut non-land prod mod")) -> ()
        n1409 = local write "University\ninvested points"(w2296) -> ()
        n1410 = local write "University upkeep"(0.015 ("Hut non-land prod mod")) -> ()
        n1411 = local write "University SP multiplier"(w2289) -> ()
        n1412 = Subtract(x=w2298, y=w2295) -> (x-y=w2297:dbl)
        n1413 = local write "Build points"(w2297) -> ()
      }
    }
    n1414 = case shown="True" w204 {
      tunnel: w211 -> [_ w2030]
      tunnel: w208 -> [_ w2029]
      frame False {
      }
      frame True {
        n1415 = local write "EP"(w2029) -> ()
        n1416 = local write "Electronics\nlevel"(w2030) -> ()
      }
    }
    n1417 = case shown="True" w197 {
      tunnel: w190 -> [_ w2028]
      tunnel: w193 -> [_ w2027]
      frame False {
      }
      frame True {
        n1418 = local write "EP"(w2027) -> ()
        n1419 = local write "Vehicle\nlevel"(w2028) -> ()
      }
    }
    n1420 = local read "University\ninvested points"() -> (w1014:dbl)
    n1421 = local read "EP"() -> (w1950:dbl)
    n1422 = case shown="True" w287 {
      tunnel: w294 -> [_ w2040]
      tunnel: w291 -> [_ w2039]
      frame False {
      }
      frame True {
        n1423 = local write "EP"(w2039) -> ()
        n1424 = local write "Electronics\nlevel"(w2040) -> ()
      }
    }
    n1425 = Greater Or Equal?(x=w1923, y=1) -> (x >= y?=w1914:bool)
    n1426 = Greater Or Equal?(x=w1917, y=0) -> (x >= y?=w1915:bool)
    n1427 = Greater Or Equal?(x=w1910, y=1) -> (x >= y?=w1901:bool)
    n1428 = Greater Or Equal?(x=w1904, y=0) -> (x >= y?=w1902:bool)
    n1429 = Not Equal?(x=w1918, y=w1912) -> (x != y?=w1920:bool)
    n1430 = Greater Or Equal?(x=w1789, y=w1790) -> (x >= y?=w1782:bool)
    n1431 = Greater Or Equal?(x=w1699, y=w1698) -> (x >= y?=w1692:bool)
    n1432 = Greater Or Equal?(x=w1731, y=w1732) -> (x >= y?=w1738:bool)
    n1433 = Greater Or Equal?(x=w1973, y=10000) -> (x >= y?=w1975:bool)
    n1434 = Subtract(x=w1789, y=w1790) -> (x-y=w1791:dbl)
    n1435 = Subtract(x=w1699, y=w1698) -> (x-y=w1697:dbl)
    n1436 = And(x="Net 1", y=w1975) -> (x .and. y?=w1962:bool)
    n1437 = Subtract(x=w1731, y=w1732) -> (x-y=w1733:dbl)
    n1438 = Not Equal?(x=w1905, y=w1899) -> (x != y?=w1907:bool)
    n1439 = Equal?(x=w1787, y=0.0) -> (x = y?=w1785:bool)
    n1440 = And(x=w1785, y=w1772) -> (x .and. y?=w1786:bool)
    n1441 = And(x=w1786, y=w1782) -> (x .and. y?=w1783:bool)
    n1442 = Equal?(x=w1701, y=0.0) -> (x = y?=w1696:bool)
    n1443 = Equal?(x=w1729, y=0.0) -> (x = y?=w1734:bool)
    n1444 = Compound Arithmetic op=AND(w1696, "Farming 1", w1693, w1692) -> (w1691:bool)
    n1445 = Greater Or Equal?(x=w953, y=2) -> (x >= y?=w954:bool)
    n1446 = Compound Arithmetic op=AND(w1734, "Raft", w1737, w1738) -> (w1739:bool)
    n1447 = Greater Or Equal?(x=w322, y=w321) -> (x >= y?=w315:bool)
    n1448 = Increment(x=w1787) -> (x+1=w1788:i32)
    n1449 = Increment(x=w1701) -> (x+1=w1700:i32)
    n1450 = Greater Or Equal?(x=w1945, y=1) -> (x >= y?=w1928:bool)
    n1451 = Increment(x=w1729) -> (x+1=w1730:i32)
    n1452 = Subtract(x=w322, y=w321) -> (x-y=w320:dbl)
    n1453 = Greater Or Equal?(x=w1931, y=0) -> (x >= y?=w1929:bool)
    n1454 = Equal?(x=w324, y=2.0) -> (x = y?=w319:bool)
    n1455 = local read "University\ninvested points"() -> (w1022:dbl)
    n1456 = Greater Or Equal?(x=w1950, y=w1949) -> (x >= y?=w1972:bool)
    n1457 = Compound Arithmetic op=AND(w319, "Caravel", w316, w315) -> (w314:bool)
    n1458 = Increment(x=w324) -> (x+1=w323:i32)
    n1459 = Subtract(x=w1950, y=w1949) -> (x-y=w1948:dbl)
    n1460 = Equal?(x=w1966, y=0.0) -> (x = y?=w1969:bool)
    n1461 = And(x=w1969, y="Sharpened stick") -> (x .and. y?=w1967:bool)
    n1462 = And(x=w1967, y=w1972) -> (x .and. y?=w1971:bool)
    n1463 = Build Array(0, w1562, w1561, w1560, w1559, w1558, w1557, w1556, w1555, w1554, w1553) -> (w1552:T2)
    n1464 = local read "Economics\nlevel"() -> (w405:i32)
    n1465 = Increment(x=w1966) -> (x+1=w1965:i32)
    n1466 = Equal?(x=w1959, y=0.0) -> (x = y?=w1961:bool)
    n1467 = And(x=w1961, y=w1962) -> (x .and. y?=w1960:bool)
    n1468 = case shown="True" w1739 {
      tunnel: w1730 -> [_ w2741]
      tunnel: w1733 -> [_ w2740]
      frame False {
      }
      frame True {
        n1469 = local read "Trading level no mod"() -> (w2739:i32)
        n1470 = local read "hunting b"() -> (w2736:dbl)
        n1471 = local write "EP"(w2740) -> ()
        n1472 = local write "Boat level"(w2741) -> ()
        n1473 = Increment(x=w2739) -> (x+1=w2738:i32)
        n1474 = local write "Trading level no mod"(w2738) -> ()
        n1475 = Add(x=0.25, y=w2736) -> (x+y=w2737:dbl)
        n1476 = local write "hunting b"(w2737) -> ()
      }
    }
    n1477 = Not Equal?(x=w1932, y=w1926) -> (x != y?=w1942:bool)
    n1478 = case shown="True" w314 {
      tunnel: w323 -> [_ w2058]
      tunnel: w320 -> [_ w2057]
      frame False {
      }
      frame True {
        n1479 = local read "Trading level no mod"() -> (w2056:i32)
        n1480 = local read "hunting b"() -> (w2054:dbl)
        n1481 = local write "EP"(w2057) -> ()
        n1482 = local write "Boat level"(w2058) -> ()
        n1483 = Increment(x=w2056) -> (x+1=w2052:i32)
        n1484 = Add(x=0.25, y=w2054) -> (x+y=w2055:dbl)
        n1485 = Increment(x=w2052) -> (x+1=w2051:i32)
        n1486 = local write "Trading level no mod"(w2051) -> ()
        n1487 = local write "hunting b"(w2055) -> ()
      }
    }
    n1488 = And(x=w1914, y=w1915) -> (x .and. y?=w1913:bool)
    n1489 = And(x="Theocracy", y=w1913) -> (x .and. y?=w1921:bool)
    n1490 = And(x=w1920, y=w1921) -> (x .and. y?=w1919:bool)
    n1491 = case shown="True" w1919 {
      tunnel: w1912 -> [_ w2815]
      frame False {
      }
      frame True {
        n1492 = local read "SP"() -> (w2812:dbl)
        n1493 = local write "Government"(w2815) -> ()
        n1494 = Subtract(x=w2812, y=0) -> (x-y=w2814:dbl)
        n1495 = local write "SP"(w2814) -> ()
      }
    }
    n1496 = local read "Taxation\nlevel"() -> (w400:dbl)
    n1497 = And(x=w1901, y=w1902) -> (x .and. y?=w1900:bool)
    n1498 = And(x="Warrior\nSociety", y=w1900) -> (x .and. y?=w1908:bool)
    n1499 = And(x=w1907, y=w1908) -> (x .and. y?=w1906:bool)
    n1500 = case shown="True" w1783 {
      tunnel: w1788 -> [_ w2760]
      tunnel: w1791 -> [_ w2759]
      frame False {
      }
      frame True {
        w2764 = 0.25
        n1501 = local read "Military Modifier"() -> (w2763:dbl)
        n1502 = local write "EP"(w2759) -> ()
        n1503 = local read "hunting b"() -> (w2765:dbl)
        n1504 = local write "Bow level"(w2760) -> ()
        n1505 = Add(x=w2764, y=w2765) -> (x+y=w2761:dbl)
        n1506 = Add(x=w2764, y=w2763) -> (x+y=w2762:dbl)
        n1507 = local write "Military Modifier"(w2762) -> ()
        n1508 = local write "hunting b"(w2761) -> ()
      }
    }
    n1509 = case shown="True" w1691 {
      tunnel: w1700 -> [_ w2720]
      tunnel: w1697 -> [_ w2719]
      frame False {
      }
      frame True {
        n1510 = local read "hunting b"() -> (w2717:dbl)
        n1511 = local read "hunting a"() -> (w2714:dbl)
        n1512 = local write "EP"(w2719) -> ()
        n1513 = local write "Farming level"(w2720) -> ()
        n1514 = Add(x=1.5, y=w2714) -> (x+y=w2713:dbl)
        n1515 = Add(x=1.5, y=w2717) -> (x+y=w2718:dbl)
        n1516 = local write "hunting b"(w2718) -> ()
        n1517 = local write "hunting a"(w2713) -> ()
      }
    }
    n1518 = case shown="True" w1906 {
      tunnel: w1899 -> [_ w2811]
      frame False {
      }
      frame True {
        n1519 = local read "SP"() -> (w2810:dbl)
        n1520 = local write "Government"(w2811) -> ()
        n1521 = Subtract(x=w2810, y=0) -> (x-y=w2808:dbl)
        n1522 = local write "SP"(w2808) -> ()
      }
    }
    n1523 = Increment(x=w1959) -> (x+1=w1958:i32)
    n1524 = case shown="True" w1971 {
      tunnel: w1965 -> [_ w3401]
      tunnel: w1948 -> [_ w3400]
      frame False {
      }
      frame True {
        w3405 = 0.25
        n1525 = local write "EP"(w3400) -> ()
        n1526 = local read "warrior a"() -> (w3404:dbl)
        n1527 = local read "hunting a"() -> (w3406:dbl)
        n1528 = local write "Spear level"(w3401) -> ()
        n1529 = Add(x=w3405, y=w3404) -> (x+y=w3403:dbl)
        n1530 = Add(x=w3405, y=w3406) -> (x+y=w3402:dbl)
        n1531 = local write "warrior a"(w3403) -> ()
        n1532 = local write "hunting a"(w3402) -> ()
      }
    }
    n1533 = case shown="True" w1960 {
      tunnel: w1973 -> [_ w3395]
      tunnel: w1958 -> [_ w3393]
      frame False {
      }
      frame True {
        n1534 = local read "hunting b"() -> (w3398:dbl)
        n1535 = local write "Net level"(w3393) -> ()
        n1536 = Subtract(x=w3395, y=10000.0) -> (x-y=w3394:dbl)
        n1537 = local write "EP"(w3394) -> ()
        n1538 = Add(x=w3398, y=0.25) -> (x+y=w3397:dbl)
        n1539 = local write "hunting b"(w3397) -> ()
      }
    }
    n1540 = And(x=w1928, y=w1929) -> (x .and. y?=w1927:bool)
    n1541 = And(x="Democracy", y=w1927) -> (x .and. y?=w1943:bool)
    n1542 = And(x=w1942, y=w1943) -> (x .and. y?=w1941:bool)
    n1543 = call-poly <vilib>:"Matrix To Array.vi"("Real Matrix"=w1552) -> ("Real 2D Array"=w1551:dbl[][])
    n1544 = case shown="True" w1941 {
      tunnel: w1926 -> [_ w2826]
      frame False {
      }
      frame True {
        n1545 = local write "Government"(w2826) -> ()
        n1546 = local read "SP"() -> (w2825:dbl)
        n1547 = Subtract(x=w2825, y=0) -> (x-y=w2823:dbl)
        n1548 = local write "SP"(w2823) -> ()
      }
    }
    n1549 = local read "Construction\nlevel"() -> (w1000:i32)
    n1550 = local read "Build points"() -> (w1005:dbl)
    n1551 = Index Array(array=w1551, index (row)=0) -> (element=w608:dbl[])  [unwired: 1 in]
    n1552 = local read "Military\nScience level"() -> (w1947:i32)
    n1553 = Greater Or Equal?(x=w405, y=1) -> (x >= y?=w398:bool)
    n1554 = And(x="Taxes level 5", y=w398) -> (x .and. y?=w403:bool)
    n1555 = Subtract(x=200000 ("y"), y=w1014) -> (x-y=w1002:dbl)
    n1556 = Not Equal?(x=w400, y=w399) -> (x != y?=w402:bool)
    n1557 = And(x=w402, y=w403) -> (x .and. y?=w401:bool)
    n1558 = local read "Construction\nlevel"() -> (w980:i32)
    n1559 = local read "University level"() -> (w975:i32)
    n1560 = local read "University level"() -> (w995:i32)
    n1561 = local read "Build points"() -> (w1016:dbl)
    n1562 = local read "Governance\nlevel"() -> (w1933:i32)
    n1563 = Subtract(x=2000000 ("y"), y=w1022) -> (x-y=w1019:dbl)
    n1564 = Max & Min(x=w1002, y=0.0) -> (max(x,y)=w1007:dbl)  [unwired: 1 out]
    n1565 = case shown="True" w401 {
      tunnel: w399 -> [_ w2072]
      frame False {
      }
      frame True {
        n1566 = local write "Taxation\nlevel"(w2072) -> ()
        n1567 = local write "Taxes dissent mod"(40.0 ("Taxes dissent add mod")) -> ()
      }
    }
    n1568 = Greater Or Equal?(x=w1005, y=w1007) -> (x >= y?=w1006:bool)
    n1569 = local read "Military\nScience level"() -> (w1823:i32)
    n1570 = Max & Min(x=w1019, y=0.0) -> (max(x,y)=w1021:dbl)  [unwired: 1 out]
    n1571 = Greater Or Equal?(x=w1016, y=w1021) -> (x >= y?=w1020:bool)
    n1572 = Greater Or Equal?(x=w980, y=3) -> (x >= y?=w974:bool)
    n1573 = Greater Or Equal?(x=w1000, y=2) -> (x >= y?=w994:bool)
    n1574 = Compound Arithmetic op=AND(w994, w1006, w954) -> (w993:bool)
    n1575 = And(x="University\nlevel 1", y=w993) -> (x .and. y?=w998:bool)
    n1576 = local read "Governance\nlevel"() -> (w1869:i32)
    n1577 = local read "Governance\nlevel"() -> (w1867:i32)
    n1578 = local read "Physics level"() -> (w262:i32)
    n1579 = local read "Physics level"() -> (w235:i32)
    n1580 = local read "Military\nScience level"() -> (w260:i32)
    n1581 = local read "Military\nScience level"() -> (w237:i32)
    n1582 = Not Equal?(x=w975, y=w972) -> (x != y?=w977:bool)
    n1583 = local read "Physics level"() -> (w273:i32)
    n1584 = local read "Physics level"() -> (w267:i32)
    n1585 = local read "Military\nScience level"() -> (w275:i32)
    n1586 = Not Equal?(x=w995, y=w992) -> (x != y?=w997:bool)
    n1587 = And(x=w997, y=w998) -> (x .and. y?=w996:bool)
    n1588 = local read "Military\nScience level"() -> (w307:i32)
    n1589 = local read "SP"() -> (w1952:dbl)
    n1590 = Increment(x=w1947) -> (x+1=w1549:i32)
    n1591 = Index Array(array=w608, index=w1549) -> (element=w1547:dbl)
    n1592 = Power Of 10(x=w1947) -> (10^x=w1956:dbl)
    n1593 = local read "SP"() -> (w1935:dbl)
    n1594 = local read "Governance\nlevel"() -> (w1882:i32)
    n1595 = Power Of 10(x=w1933) -> (10^x=w1939:dbl)
    n1596 = Power Of 2(x=w1547) -> (2^x=w1548:dbl)
    n1597 = local read "Government"() -> (w1887:string)
    n1598 = local read "Governance\nlevel"() -> (w949:i32)
    n1599 = local read "Government"() -> (w1874:string)
    n1600 = local read "Government"() -> (w1862:string)
    n1601 = local read "Net level"() -> (w1842:i32)
    n1602 = Compound Arithmetic op=MULTIPLY(w1956, 1000, w1548) -> (w1951:dbl)
    n1603 = local read "Military\nScience level"() -> (w1579:i32)
    n1604 = case shown="True" w996 {
      tunnel: w992 -> [_ w2312]
      tunnel: w1014 -> [_ w2309]
      tunnel: w1007 -> [_ w2307]
      tunnel: w1023 -> [_ w2300]
      frame False {
      }
      frame True {
        n1605 = Multiply(x=w2300, y=0.15) -> (x*y=w2302:dbl)
        n1606 = Increment(x=w2302) -> (x+1=w2303:dbl)
        n1607 = local read "Build points"() -> (w2311:dbl)
        n1608 = Add(x=w2307, y=w2309) -> (x+y=w2308:dbl)
        n1609 = local write "University level"(w2312) -> ()
        n1610 = local write "University scientist equivalent"(0.02 ("Hut dissent add mod")) -> ()
        n1611 = local write "University\ninvested points"(w2308) -> ()
        n1612 = local write "University SP multiplier"(w2303) -> ()
        n1613 = local write "University dissent mod"(0.98 ("Hut non-land prod mod")) -> ()
        n1614 = local write "University upkeep"(0.005 ("Hut non-land prod mod")) -> ()
        n1615 = Subtract(x=w2311, y=w2307) -> (x-y=w2310:dbl)
        n1616 = local write "Build points"(w2310) -> ()
      }
    }
    n1617 = local read "Military\nScience level"() -> (w340:i32)
    n1618 = local read "EP"() -> (w1836:dbl)
    n1619 = local read "Military\nScience level"() -> (w1769:i32)
    n1620 = Greater?(x=w1952, y=w1951) -> (0:w1954:bool)
    n1621 = And(x="Military science", y=w1954) -> (x .and. y?=w1953:bool)
    n1622 = local read "SP"() -> (w1888:dbl)
    n1623 = local read "SP"() -> (w1875:dbl)
    n1624 = local read "SP"() -> (w1861:dbl)
    n1625 = local read "Physics level"() -> (w1744:i32)
    n1626 = local read "Physics level"() -> (w1717:i32)
    n1627 = Greater Or Equal?(x=w1836, y=100000) -> (x >= y?=w1834:bool)
    n1628 = local read "Physics level"() -> (w336:i32)
    n1629 = local read "Biology\nlevel"() -> (w1675:i32)
    n1630 = And(x="Net 2", y=w1834) -> (x .and. y?=w1839:bool)
    n1631 = Greater Or Equal?(x=w1823, y=1.0) -> (x >= y?=w1822:bool)
    n1632 = case shown="True" w1953 {
      selector: w1953 -> [w3383 w3386]
      tunnel: w1952 -> [_ w3389]
      tunnel: w1951 -> [_ w3388]
      tunnel: w1549 -> [_ w3385]
      tunnel: [w3383 w3386] -> w1564
      tunnel: [0 w3385] -> w1575
      frame False {
      }
      frame True {
        n1633 = local read "warrior c"() -> (w3392:dbl)
        n1634 = Subtract(x=w3389, y=w3388) -> (x-y=w3387:dbl)
        n1635 = local write "SP"(w3387) -> ()
        n1636 = Subtract(x=w3392, y=0.03) -> (x-y=w3391:dbl)
        n1637 = local write "Military\nScience level"(w3385) -> ()
        n1638 = local write "warrior c"(w3391) -> ()
      }
    }
    n1639 = Increment(x=w1933) -> (x+1=w1544:i32)
    n1640 = Index Array(array=w608, index=w1544) -> (element=w1546:dbl)
    n1641 = Power Of 2(x=w1546) -> (2^x=w1545:dbl)
    n1642 = Compound Arithmetic op=MULTIPLY(w1939, 1000, w1545) -> (w1934:dbl)
    n1643 = Greater?(x=w1935, y=w1934) -> (0:w1937:bool)
    n1644 = And(x="Governance", y=w1937) -> (x .and. y?=w1936:bool)
    n1645 = case shown="True" w1936 {
      selector: w1936 -> [w2816 w2819]
      tunnel: w1935 -> [_ w2822]
      tunnel: w1934 -> [_ w2821]
      tunnel: w1544 -> [_ w2818]
      tunnel: [w2816 w2819] -> w1565
      tunnel: [0 w2818] -> w1574
      frame False {
      }
      frame True {
        n1646 = Subtract(x=w2822, y=w2821) -> (x-y=w2820:dbl)
        n1647 = local write "SP"(w2820) -> ()
        n1648 = local write "Governance\nlevel"(w2818) -> ()
      }
    }
    n1649 = Greater Or Equal?(x=w1882, y=2) -> (x >= y?=w1891:bool)
    n1650 = Greater Or Equal?(x=w1888, y=100000) -> (x >= y?=w1890:bool)
    n1651 = local read "Optics\nlevel"() -> (w257:i32)
    n1652 = Greater Or Equal?(x=w1869, y=2) -> (x >= y?=w1878:bool)
    n1653 = Equal?(x=w1842, y=1.0) -> (x = y?=w1840:bool)
    n1654 = And(x=w1840, y=w1839) -> (x .and. y?=w1841:bool)
    n1655 = local read "Optics\nlevel"() -> (w240:i32)
    n1656 = Greater Or Equal?(x=w1867, y=2) -> (x >= y?=w1858:bool)
    n1657 = Greater Or Equal?(x=w1875, y=100000) -> (x >= y?=w1877:bool)
    n1658 = Greater Or Equal?(x=w1861, y=100000) -> (x >= y?=w1859:bool)
    n1659 = And(x="Stone\nspear", y=w1822) -> (x .and. y?=w1820:bool)
    n1660 = local read "Optics\nlevel"() -> (w278:i32)
    n1661 = Greater Or Equal?(x=w949, y=2) -> (x >= y?=w947:bool)
    n1662 = Compound Arithmetic op=AND(w974, w1020, w947) -> (w973:bool)
    n1663 = And(x="University\nlevel 3", y=w973) -> (x .and. y?=w978:bool)
    n1664 = And(x=w977, y=w978) -> (x .and. y?=w976:bool)
    n1665 = case shown="True" w976 {
      tunnel: w972 -> [_ w2286]
      tunnel: w1021 -> [_ w2282]
      tunnel: w1022 -> [_ w2281]
      tunnel: w1023 -> [_ w2274]
      frame False {
      }
      frame True {
        n1666 = Multiply(x=w2274, y=0.45) -> (x*y=w2277:dbl)
        n1667 = local read "Build points"() -> (w2285:dbl)
        n1668 = Add(x=w2282, y=w2281) -> (x+y=w2283:dbl)
        n1669 = Increment(x=w2277) -> (x+1=w2276:dbl)
        n1670 = local write "University level"(w2286) -> ()
        n1671 = local write "University scientist equivalent"(0.06 ("Hut dissent add mod")) -> ()
        n1672 = local write "University\ninvested points"(w2283) -> ()
        n1673 = local write "University dissent mod"(0.94 ("Hut non-land prod mod")) -> ()
        n1674 = local write "University SP multiplier"(w2276) -> ()
        n1675 = local write "University upkeep"(0.05 ("Hut non-land prod mod")) -> ()
        n1676 = Subtract(x=w2285, y=w2282) -> (x-y=w2284:dbl)
        n1677 = local write "Build points"(w2284) -> ()
      }
    }
    n1678 = local read "Economics\nlevel"() -> (w390:i32)
    n1679 = Not Equal?(x=w1887, y=w1893) -> (x != y?=w1885:bool)
    n1680 = local read "Optics\nlevel"() -> (w298:i32)
    n1681 = Not Equal?(x=w1874, y=w1880) -> (x != y?=w1872:bool)
    n1682 = Not Equal?(x=w1862, y=w1856) -> (x != y?=w1864:bool)
    n1683 = local read "Spear level"() -> (w1826:i32)
    n1684 = Greater Or Equal?(x=w262, y=6.0) -> (x >= y?=w264:bool)
    n1685 = Increment(x=w1842) -> (x+1=w1843:i32)
    n1686 = Greater Or Equal?(x=w235, y=6.0) -> (x >= y?=w233:bool)
    n1687 = local read "Taxation\nlevel"() -> (w395:dbl)
    n1688 = Greater Or Equal?(x=w273, y=4.0) -> (x >= y?=w271:bool)
    n1689 = Greater Or Equal?(x=w267, y=6.0) -> (x >= y?=w265:bool)
    n1690 = case shown="True" w1841 {
      tunnel: w1836 -> [_ w2791]
      tunnel: w1843 -> [_ w2789]
      frame False {
      }
      frame True {
        n1691 = local read "hunting b"() -> (w2794:dbl)
        n1692 = local write "Net level"(w2789) -> ()
        n1693 = Subtract(x=w2791, y=10000.0) -> (x-y=w2790:dbl)
        n1694 = local write "EP"(w2790) -> ()
        n1695 = Add(x=w2794, y=0.25) -> (x+y=w2793:dbl)
        n1696 = local write "hunting b"(w2793) -> ()
      }
    }
    n1697 = And(x=w1891, y=w1890) -> (x .and. y?=w1892:bool)
    n1698 = And(x="Democracy 2", y=w1892) -> (x .and. y?=w1884:bool)
    n1699 = And(x=w1885, y=w1884) -> (x .and. y?=w1886:bool)
    n1700 = local read "EP"() -> (w1831:dbl)
    n1701 = case shown="True" w1886 {
      tunnel: w1893 -> [_ w2807]
      frame False {
      }
      frame True {
        n1702 = local write "Government"(w2807) -> ()
        n1703 = local read "SP"() -> (w2804:dbl)
        n1704 = Subtract(x=w2804, y=100000) -> (x-y=w2806:dbl)
        n1705 = local write "SP"(w2806) -> ()
      }
    }
    n1706 = And(x=w1878, y=w1877) -> (x .and. y?=w1879:bool)
    n1707 = And(x="Theocracy 2", y=w1879) -> (x .and. y?=w1871:bool)
    n1708 = And(x=w1872, y=w1871) -> (x .and. y?=w1873:bool)
    n1709 = And(x=w1858, y=w1859) -> (x .and. y?=w1857:bool)
    n1710 = And(x="Warrior\nSociety 2", y=w1857) -> (x .and. y?=w1865:bool)
    n1711 = And(x=w1864, y=w1865) -> (x .and. y?=w1863:bool)
    n1712 = Greater Or Equal?(x=w260, y=4.0) -> (x >= y?=w261:bool)
    n1713 = case shown="True" w1873 {
      tunnel: w1880 -> [_ w2803]
      frame False {
      }
      frame True {
        n1714 = local write "Government"(w2803) -> ()
        n1715 = local read "SP"() -> (w2802:dbl)
        n1716 = Subtract(x=w2802, y=100000) -> (x-y=w2800:dbl)
        n1717 = local write "SP"(w2800) -> ()
      }
    }
    n1718 = Greater Or Equal?(x=w237, y=4.0) -> (x >= y?=w236:bool)
    n1719 = case shown="True" w1863 {
      tunnel: w1856 -> [_ w2799]
      frame False {
      }
      frame True {
        n1720 = local write "Government"(w2799) -> ()
        n1721 = local read "SP"() -> (w2796:dbl)
        n1722 = Subtract(x=w2796, y=100000) -> (x-y=w2798:dbl)
        n1723 = local write "SP"(w2798) -> ()
      }
    }
    n1724 = Greater Or Equal?(x=w275, y=4.0) -> (x >= y?=w274:bool)
    n1725 = Greater Or Equal?(x=w307, y=3.0) -> (x >= y?=w312:bool)
    n1726 = Greater Or Equal?(x=w1831, y=3000) -> (x >= y?=w1833:bool)
    n1727 = And(x=w1820, y=w1833) -> (x .and. y?=w1829:bool)
    n1728 = local read "EP"() -> (w255:dbl)
    n1729 = local read "EP"() -> (w242:dbl)
    n1730 = local read "EP"() -> (w300:dbl)
    n1731 = local read "EP"() -> (w280:dbl)
    n1732 = Equal?(x=w1826, y=1.0) -> (x = y?=w1828:bool)
    n1733 = And(x=w1828, y=w1829) -> (x .and. y?=w1827:bool)
    n1734 = Greater Or Equal?(x=w1744, y=3.0) -> (x >= y?=w1742:bool)
    n1735 = local read "Bow level"() -> (w1767:i32)
    n1736 = local read "Farming level"() -> (w1668:i32)
    n1737 = Greater Or Equal?(x=w1717, y=4.0) -> (x >= y?=w1716:bool)
    n1738 = local read "Boat level"() -> (w1724:i32)
    n1739 = Greater Or Equal?(x=w1579, y=3.0) -> (x >= y?=w1577:bool)
    n1740 = Greater Or Equal?(x=w336, y=4.0) -> (x >= y?=w337:bool)
    n1741 = Greater Or Equal?(x=w1675, y=4.0) -> (x >= y?=w1676:bool)
    n1742 = Greater Or Equal?(x=w390, y=1) -> (x >= y?=w397:bool)
    n1743 = local read "Boat level"() -> (w329:i32)
    n1744 = And(x="Taxes level 6", y=w397) -> (x .and. y?=w392:bool)
    n1745 = Greater Or Equal?(x=w340, y=3.0) -> (x >= y?=w342:bool)
    n1746 = Greater Or Equal?(x=w1769, y=3.0) -> (x >= y?=w1743:bool)
    n1747 = Increment(x=w1826) -> (x+1=w1825:i32)
    n1748 = Not Equal?(x=w395, y=w396) -> (x != y?=w393:bool)
    n1749 = And(x=w393, y=w392) -> (x .and. y?=w394:bool)
    n1750 = Greater Or Equal?(x=w255, y=w254) -> (x >= y?=w250:bool)
    n1751 = Greater Or Equal?(x=w242, y=w243) -> (x >= y?=w247:bool)
    n1752 = Subtract(x=w255, y=w254) -> (x-y=w253:dbl)
    n1753 = Subtract(x=w242, y=w243) -> (x-y=w244:dbl)
    n1754 = Equal?(x=w257, y=2.0) -> (x = y?=w252:bool)
    n1755 = Greater Or Equal?(x=w300, y=w301) -> (x >= y?=w305:bool)
    n1756 = Compound Arithmetic op=AND(w252, "Mechanical\nTelevision", w261, w264, w250) -> (w249:bool)
    n1757 = Equal?(x=w240, y=3.0) -> (x = y?=w245:bool)
    n1758 = Compound Arithmetic op=AND(w245, "LCD monitor", w236, w233, w247) -> (w248:bool)
    n1759 = local read "EP"() -> (w1765:dbl)
    n1760 = Greater Or Equal?(x=w280, y=w281) -> (x >= y?=w285:bool)
    n1761 = Increment(x=w257) -> (x+1=w256:i32)
    n1762 = Subtract(x=w300, y=w301) -> (x-y=w302:dbl)
    n1763 = Increment(x=w240) -> (x+1=w241:i32)
    n1764 = Equal?(x=w298, y=0.0) -> (x = y?=w303:bool)
    n1765 = Subtract(x=w280, y=w281) -> (x-y=w282:dbl)
    n1766 = Compound Arithmetic op=AND(w303, "Telescope", w312, w271, w305) -> (w306:bool)
    n1767 = local read "EP"() -> (w1722:dbl)
    n1768 = Equal?(x=w278, y=1.0) -> (x = y?=w283:bool)
    n1769 = Compound Arithmetic op=AND(w283, "Camera", w274, w265, w285) -> (w286:bool)
    n1770 = case shown="True" w1827 {
      tunnel: w1831 -> [_ w2787]
      tunnel: w1825 -> [_ w2785]
      frame False {
      }
      frame True {
        w2781 = 0.25
        n1771 = local read "warrior a"() -> (w2782:dbl)
        n1772 = local read "hunting a"() -> (w2780:dbl)
        n1773 = local write "Spear level"(w2785) -> ()
        n1774 = Subtract(x=w2787, y=3000.0) -> (x-y=w2786:dbl)
        n1775 = local write "EP"(w2786) -> ()
        n1776 = Add(x=w2781, y=w2782) -> (x+y=w2783:dbl)
        n1777 = Add(x=w2781, y=w2780) -> (x+y=w2784:dbl)
        n1778 = local write "warrior a"(w2783) -> ()
        n1779 = local write "hunting a"(w2784) -> ()
      }
    }
    n1780 = Increment(x=w278) -> (x+1=w279:i32)
    n1781 = local read "EP"() -> (w331:dbl)
    n1782 = local read "EP"() -> (w1670:dbl)
    n1783 = Increment(x=w298) -> (x+1=w299:i32)
    n1784 = case shown="True" w394 {
      tunnel: w396 -> [_ w2070]
      frame False {
      }
      frame True {
        n1785 = local write "Taxation\nlevel"(w2070) -> ()
        n1786 = local write "Taxes dissent mod"(60.0 ("Taxes dissent add mod")) -> ()
      }
    }
    n1787 = Greater Or Equal?(x=w1765, y=w1764) -> (x >= y?=w1741:bool)
    n1788 = Subtract(x=w1765, y=w1764) -> (x-y=w1763:dbl)
    n1789 = Equal?(x=w1767, y=1.0) -> (x = y?=w1748:bool)
    n1790 = Greater Or Equal?(x=w1722, y=w1721) -> (x >= y?=w1715:bool)
    n1791 = Compound Arithmetic op=AND(w1748, "Bow 2", w1743, w1742, w1741) -> (w1740:bool)
    n1792 = Increment(x=w1767) -> (x+1=w1766:i32)
    n1793 = Subtract(x=w1722, y=w1721) -> (x-y=w1720:dbl)
    n1794 = case shown="True" w306 {
      tunnel: w299 -> [_ w2042]
      tunnel: w302 -> [_ w2041]
      frame False {
      }
      frame True {
        n1795 = local write "EP"(w2041) -> ()
        n1796 = local write "Optics\nlevel"(w2042) -> ()
      }
    }
    n1797 = Equal?(x=w1724, y=1.0) -> (x = y?=w1719:bool)
    n1798 = Compound Arithmetic op=AND(w1719, "Trireme", w1716, w1577, w1715) -> (w1714:bool)
    n1799 = Greater Or Equal?(x=w331, y=w332) -> (x >= y?=w338:bool)
    n1800 = Greater Or Equal?(x=w1670, y=w1671) -> (x >= y?=w1677:bool)
    n1801 = Increment(x=w1724) -> (x+1=w1723:i32)
    n1802 = Subtract(x=w331, y=w332) -> (x-y=w333:dbl)
    n1803 = Subtract(x=w1670, y=w1671) -> (x-y=w1672:dbl)
    n1804 = case shown="True" w249 {
      tunnel: w256 -> [_ w2036]
      tunnel: w253 -> [_ w2035]
      frame False {
      }
      frame True {
        n1805 = local write "EP"(w2035) -> ()
        n1806 = local write "Optics\nlevel"(w2036) -> ()
      }
    }
    n1807 = Equal?(x=w329, y=3.0) -> (x = y?=w334:bool)
    n1808 = Equal?(x=w1668, y=1.0) -> (x = y?=w1673:bool)
    n1809 = case shown="True" w248 {
      tunnel: w241 -> [_ w2034]
      tunnel: w244 -> [_ w2033]
      frame False {
      }
      frame True {
        n1810 = local write "EP"(w2033) -> ()
        n1811 = local write "Optics\nlevel"(w2034) -> ()
      }
    }
    n1812 = Compound Arithmetic op=AND(w334, "Steamship", w337, w342, w338) -> (w339:bool)
    n1813 = Compound Arithmetic op=AND(w1673, "Farming 2", w1676, w1677) -> (w1678:bool)
    n1814 = Increment(x=w329) -> (x+1=w330:i32)
    n1815 = Increment(x=w1668) -> (x+1=w1669:i32)
    n1816 = case shown="True" w286 {
      tunnel: w279 -> [_ w2038]
      tunnel: w282 -> [_ w2037]
      frame False {
      }
      frame True {
        n1817 = local write "EP"(w2037) -> ()
        n1818 = local write "Optics\nlevel"(w2038) -> ()
      }
    }
    n1819 = case shown="True" w1714 {
      tunnel: w1723 -> [_ w2734]
      tunnel: w1720 -> [_ w2733]
      frame False {
      }
      frame True {
        n1820 = local read "Trading level no mod"() -> (w2732:i32)
        n1821 = local read "warrior b"() -> (w2729:dbl)
        n1822 = local write "EP"(w2733) -> ()
        n1823 = local write "Boat level"(w2734) -> ()
        n1824 = Increment(x=w2732) -> (x+1=w2731:i32)
        n1825 = local write "Trading level no mod"(w2731) -> ()
        n1826 = Add(x=0.5, y=w2729) -> (x+y=w2730:dbl)
        n1827 = local write "warrior b"(w2730) -> ()
      }
    }
    n1828 = local read "Military\nScience level"() -> (w1026:i32)
    n1829 = case shown="True" w339 {
      tunnel: w330 -> [_ w2050]
      tunnel: w333 -> [_ w2049]
      frame False {
      }
      frame True {
        n1830 = local read "Trading level no mod"() -> (w2043:i32)
        n1831 = local write "EP"(w2049) -> ()
        n1832 = local read "warrior b"() -> (w2047:dbl)
        n1833 = local write "Boat level"(w2050) -> ()
        n1834 = Add(x=0.5, y=w2047) -> (x+y=w2048:dbl)
        n1835 = Increment(x=w2043) -> (x+1=w2044:i32)
        n1836 = Increment(x=w2044) -> (x+1=w2045:i32)
        n1837 = local write "Trading level no mod"(w2045) -> ()
        n1838 = local write "warrior b"(w2048) -> ()
      }
    }
    n1839 = case shown="True" w1740 {
      tunnel: w1766 -> [_ w2758]
      tunnel: w1763 -> [_ w2757]
      frame False {
      }
      frame True {
        w2752 = 0.5 ("x")
        n1840 = local read "hunting a"() -> (w2756:dbl)
        n1841 = local read "warrior a"() -> (w2753:dbl)
        n1842 = local write "EP"(w2757) -> ()
        n1843 = local write "Bow level"(w2758) -> ()
        n1844 = Add(x=w2752, y=w2756) -> (x+y=w2755:dbl)
        n1845 = Add(x=w2752, y=w2753) -> (x+y=w2754:dbl)
        n1846 = local write "hunting a"(w2755) -> ()
        n1847 = local write "warrior a"(w2754) -> ()
      }
    }
    n1848 = case shown="True" w1678 {
      tunnel: w1669 -> [_ w2707]
      tunnel: w1672 -> [_ w2706]
      frame False {
      }
      frame True {
        n1849 = local read "hunting b"() -> (w2704:dbl)
        n1850 = local read "hunting a"() -> (w2701:dbl)
        n1851 = local write "EP"(w2706) -> ()
        n1852 = local write "Farming level"(w2707) -> ()
        n1853 = Add(x=1.5, y=w2701) -> (x+y=w2700:dbl)
        n1854 = Add(x=1.5, y=w2704) -> (x+y=w2705:dbl)
        n1855 = local write "hunting b"(w2705) -> ()
        n1856 = local write "hunting a"(w2700) -> ()
      }
    }
    n1857 = local read "Physics level"() -> (w1037:i32)
    n1858 = local read "Governance\nlevel"() -> (w1236:i32)
    n1859 = local read "Governance\nlevel"() -> (w1238:i32)
    n1860 = local read "Physics level"() -> (w1755:i32)
    n1861 = local read "Governance\nlevel"() -> (w1223:i32)
    n1862 = local read "Construction\nlevel"() -> (w1762:i32)
    n1863 = local read "Government"() -> (w1218:string)
    n1864 = local read "Government"() -> (w1231:string)
    n1865 = local read "Government"() -> (w1243:string)
    n1866 = local read "SP"() -> (w1217:dbl)
    n1867 = local read "SP"() -> (w1230:dbl)
    n1868 = local read "SP"() -> (w1244:dbl)
    n1869 = local read "Military\nScience level"() -> (w1802:i32)
    n1870 = Greater Or Equal?(x=w1037, y=4.0) -> (x >= y?=w1039:bool)
    n1871 = local read "Bow level"() -> (w1028:i32)
    n1872 = Greater Or Equal?(x=w1223, y=4) -> (x >= y?=w1214:bool)
    n1873 = Greater Or Equal?(x=w1802, y=2.0) -> (x >= y?=w1803:bool)
    n1874 = Greater Or Equal?(x=w1217, y=5000000) -> (x >= y?=w1215:bool)
    n1875 = Greater Or Equal?(x=w1236, y=4) -> (x >= y?=w1227:bool)
    n1876 = Greater Or Equal?(x=w1238, y=4) -> (x >= y?=w1247:bool)
    n1877 = Greater Or Equal?(x=w1230, y=5000000) -> (x >= y?=w1228:bool)
    n1878 = Greater Or Equal?(x=w1244, y=5000000) -> (x >= y?=w1246:bool)
    n1879 = Greater Or Equal?(x=w1026, y=5.0) -> (x >= y?=w1038:bool)
    n1880 = Not Equal?(x=w1218, y=w1212) -> (x != y?=w1220:bool)
    n1881 = And(x="Bronze\nSpear", y=w1803) -> (x .and. y?=w1799:bool)
    n1882 = Not Equal?(x=w1231, y=w1225) -> (x != y?=w1233:bool)
    n1883 = Not Equal?(x=w1243, y=w1249) -> (x != y?=w1241:bool)
    n1884 = local read "SP"() -> (w1753:dbl)
    n1885 = local read "EP"() -> (w1030:dbl)
    n1886 = local read "Spear level"() -> (w1813:i32)
    n1887 = Power Of 10(x=w1755) -> (10^x=w1750:dbl)
    n1888 = local read "SP"() -> (w1760:dbl)
    n1889 = And(x=w1214, y=w1215) -> (x .and. y?=w1213:bool)
    n1890 = And(x="Confederacy", y=w1213) -> (x .and. y?=w1221:bool)
    n1891 = And(x=w1220, y=w1221) -> (x .and. y?=w1219:bool)
    n1892 = Power Of 10(x=w1762) -> (10^x=w1757:dbl)
    n1893 = case shown="True" w1219 {
      tunnel: w1212 -> [_ w2399]
      frame False {
      }
      frame True {
        n1894 = local write "Government"(w2399) -> ()
        n1895 = local read "SP"() -> (w2396:dbl)
        n1896 = Subtract(x=w2396, y=5000000) -> (x-y=w2398:dbl)
        n1897 = local write "SP"(w2398) -> ()
      }
    }
    n1898 = And(x=w1227, y=w1228) -> (x .and. y?=w1226:bool)
    n1899 = And(x="Republic", y=w1226) -> (x .and. y?=w1234:bool)
    n1900 = And(x=w1233, y=w1234) -> (x .and. y?=w1232:bool)
    n1901 = And(x=w1247, y=w1246) -> (x .and. y?=w1248:bool)
    n1902 = And(x="Kingdom", y=w1248) -> (x .and. y?=w1240:bool)
    n1903 = And(x=w1241, y=w1240) -> (x .and. y?=w1242:bool)
    n1904 = case shown="True" w1232 {
      tunnel: w1225 -> [_ w2395]
      frame False {
      }
      frame True {
        n1905 = local write "Government"(w2395) -> ()
        n1906 = local read "SP"() -> (w2394:dbl)
        n1907 = Subtract(x=w2394, y=5000000) -> (x-y=w2392:dbl)
        n1908 = local write "SP"(w2392) -> ()
      }
    }
    n1909 = case shown="True" w1242 {
      tunnel: w1249 -> [_ w2391]
      frame False {
      }
      frame True {
        n1910 = local write "Government"(w2391) -> ()
        n1911 = local read "SP"() -> (w2388:dbl)
        n1912 = Subtract(x=w2388, y=5000000) -> (x-y=w2390:dbl)
        n1913 = local write "SP"(w2390) -> ()
      }
    }
    n1914 = local read "EP"() -> (w1818:dbl)
    n1915 = Greater Or Equal?(x=w1030, y=w1031) -> (x >= y?=w1040:bool)
    n1916 = Subtract(x=w1030, y=w1031) -> (x-y=w1032:dbl)
    n1917 = Equal?(x=w1028, y=2.0) -> (x = y?=w1033:bool)
    n1918 = Compound Arithmetic op=AND(w1033, "Longbow", w1038, w1039, w1040) -> (w1041:bool)
    n1919 = Increment(x=w1028) -> (x+1=w1029:i32)
    n1920 = Greater Or Equal?(x=w1818, y=w1792) -> (x >= y?=w1819:bool)
    n1921 = And(x=w1799, y=w1819) -> (x .and. y?=w1816:bool)
    n1922 = Increment(x=w1755) -> (x+1=w1543:i32)
    n1923 = Index Array(array=w608, index=w1543) -> (element=w1542:dbl)
    n1924 = Power Of 2(x=w1542) -> (2^x=w1541:dbl)
    n1925 = Compound Arithmetic op=MULTIPLY(w1750, 1000, w1541) -> (w1754:dbl)
    n1926 = Greater?(x=w1753, y=w1754) -> (0:w1752:bool)
    n1927 = And(x="Physics", y=w1752) -> (x .and. y?=w1566:bool)
    n1928 = Equal?(x=w1813, y=2.0) -> (x = y?=w1815:bool)
    n1929 = And(x=w1815, y=w1816) -> (x .and. y?=w1814:bool)
    n1930 = local read "Physics level"() -> (w624:i32)
    n1931 = local read "Physics level"() -> (w651:i32)
    n1932 = local read "Military\nScience level"() -> (w626:i32)
    n1933 = case shown="True" w1041 {
      tunnel: w1029 -> [_ w2317]
      tunnel: w1032 -> [_ w2316]
      frame False {
      }
      frame True {
        n1934 = local write "EP"(w2316) -> ()
        n1935 = local read "warrior a"() -> (w2314:dbl)
        n1936 = local write "Bow level"(w2317) -> ()
        n1937 = Add(x=0.25, y=w2314) -> (x+y=w2315:dbl)
        n1938 = local write "warrior a"(w2315) -> ()
      }
    }
    n1939 = local read "Military\nScience level"() -> (w649:i32)
    n1940 = local read "Physics level"() -> (w656:i32)
    n1941 = local read "Military\nScience level"() -> (w658:i32)
    n1942 = local read "Physics level"() -> (w715:i32)
    n1943 = local read "Military\nScience level"() -> (w672:i32)
    n1944 = local read "Physics level"() -> (w713:i32)
    n1945 = local read "Military\nScience level"() -> (w707:i32)
    n1946 = case shown="True" w1566 {
      tunnel: w1753 -> [_ w2751]
      tunnel: w1754 -> [_ w2750]
      tunnel: w1543 -> [_ w2748]
      tunnel: [0 w2748] -> w1573
      frame False {
      }
      frame True {
        n1947 = Subtract(x=w2751, y=w2750) -> (x-y=w2749:dbl)
        n1948 = local write "SP"(w2749) -> ()
        n1949 = local write "Physics level"(w2748) -> ()
      }
    }
    n1950 = local read "Physics level"() -> (w709:i32)
    n1951 = Increment(x=w1813) -> (x+1=w1812:i32)
    n1952 = local read "Military\nScience level"() -> (w675:i32)
    n1953 = Increment(x=w1762) -> (x+1=w1540:i32)
    n1954 = Index Array(array=w608, index=w1540) -> (element=w1539:dbl)
    n1955 = Power Of 2(x=w1539) -> (2^x=w1538:dbl)
    n1956 = Compound Arithmetic op=MULTIPLY(w1757, 1000, w1538) -> (w1761:dbl)
    n1957 = Greater?(x=w1760, y=w1761) -> (0:w1759:bool)
    n1958 = And(x="Construction", y=w1759) -> (x .and. y?=w1567:bool)
    n1959 = case shown="True" w1567 {
      tunnel: w1760 -> [_ w2746]
      tunnel: w1761 -> [_ w2745]
      tunnel: w1540 -> [_ w2743]
      tunnel: [0 w2743] -> w1572
      frame False {
      }
      frame True {
        n1960 = Subtract(x=w2746, y=w2745) -> (x-y=w2744:dbl)
        n1961 = local write "SP"(w2744) -> ()
        n1962 = local write "Construction\nlevel"(w2743) -> ()
      }
    }
    n1963 = case shown="True" w1814 {
      tunnel: w1818 -> [_ w2776]
      tunnel: w1812 -> [_ w2774]
      tunnel: w1792 -> [_ w2773]
      frame False {
      }
      frame True {
        n1964 = local read "warrior a"() -> (w2778:dbl)
        n1965 = local write "Spear level"(w2774) -> ()
        n1966 = Subtract(x=w2776, y=w2773) -> (x-y=w2775:dbl)
        n1967 = local write "EP"(w2775) -> ()
        n1968 = Add(x=w2778, y=0.5) -> (x+y=w2777:dbl)
        n1969 = local write "warrior a"(w2777) -> ()
      }
    }
    n1970 = local read "Economics\nlevel"() -> (w799:i32)
    n1971 = local read "Economics\nlevel"() -> (w800:i32)
    n1972 = local read "Economics\nlevel"() -> (w796:i32)
    n1973 = local read "Biology\nlevel"() -> (w1070:i32)
    n1974 = local read "Biology\nlevel"() -> (w353:i32)
    n1975 = local read "Biology\nlevel"() -> (w1071:i32)
    n1976 = local read "Construction\nlevel"() -> (w1042:i32)
    n1977 = local read "Construction\nlevel"() -> (w1286:i32)
    n1978 = local read "Biology\nlevel"() -> (w1096:i32)
    n1979 = local read "Construction\nlevel"() -> (w1287:i32)
    n1980 = local read "Military\nScience level"() -> (w1797:i32)
    n1981 = local read "Physics level"() -> (w1053:i32)
    n1982 = local read "Physics level"() -> (w1275:i32)
    n1983 = local read "Physics level"() -> (w1298:i32)
    n1984 = local read "Siege weapon\nlevel"() -> (w629:i32)
    n1985 = local read "Siege weapon\nlevel"() -> (w646:i32)
    n1986 = local read "Siege weapon\nlevel"() -> (w661:i32)
    n1987 = local read "Siege weapon\nlevel"() -> (w687:i32)
    n1988 = local read "Siege weapon\nlevel"() -> (w704:i32)
    n1989 = local read "Siege weapon\nlevel"() -> (w684:i32)
    n1990 = local read "Tax method\nlevel"() -> (w767:i32)
    n1991 = local read "Tax method\nlevel"() -> (w784:i32)
    n1992 = local read "Construction\ntools level"() -> (w1044:i32)
    n1993 = local read "Construction\ntools level"() -> (w1284:i32)
    n1994 = local read "Medicine level"() -> (w1068:i32)
    n1995 = local read "Medicine level"() -> (w355:i32)
    n1996 = Greater Or Equal?(x=w624, y=9.0) -> (x >= y?=w622:bool)
    n1997 = local read "Medicine level"() -> (w1073:i32)
    n1998 = Greater Or Equal?(x=w651, y=9.0) -> (x >= y?=w653:bool)
    n1999 = local read "Tax method\nlevel"() -> (w787:i32)
    n2000 = local read "Governance\nlevel"() -> (w1187:i32)
    n2001 = Greater Or Equal?(x=w656, y=7.0) -> (x >= y?=w654:bool)
    n2002 = local read "Governance\nlevel"() -> (w1185:i32)
    n2003 = local read "Construction\ntools level"() -> (w1289:i32)
    n2004 = Greater Or Equal?(x=w715, y=6.0) -> (x >= y?=w717:bool)
    n2005 = Greater Or Equal?(x=w713, y=5.0) -> (x >= y?=w714:bool)
    n2006 = local read "Medicine level"() -> (w1094:i32)
    n2007 = Greater Or Equal?(x=w709, y=4.0) -> (x >= y?=w711:bool)
    n2008 = Greater Or Equal?(x=w626, y=9.0) -> (x >= y?=w625:bool)
    n2009 = Greater Or Equal?(x=w649, y=8.0) -> (x >= y?=w650:bool)
    n2010 = Greater Or Equal?(x=w658, y=6.0) -> (x >= y?=w657:bool)
    n2011 = Greater Or Equal?(x=w672, y=3.0) -> (x >= y?=w671:bool)
    n2012 = Greater Or Equal?(x=w707, y=4.0) -> (x >= y?=w708:bool)
    n2013 = local read "Governance\nlevel"() -> (w1200:i32)
    n2014 = Greater Or Equal?(x=w675, y=3.0) -> (x >= y?=w670:bool)
    n2015 = local read "Government"() -> (w1205:string)
    n2016 = local read "Government"() -> (w1192:string)
    n2017 = local read "Government"() -> (w1180:string)
    n2018 = local read "Economics\nlevel"() -> (w1704:i32)
    n2019 = Greater Or Equal?(x=w799, y=4.0) -> (x >= y?=w803:bool)
    n2020 = Greater Or Equal?(x=w800, y=6.0) -> (x >= y?=w802:bool)
    n2021 = local read "Biology\nlevel"() -> (w1690:i32)
    n2022 = local read "EP"() -> (w631:dbl)
    n2023 = Greater Or Equal?(x=w796, y=3.0) -> (x >= y?=w804:bool)
    n2024 = local read "EP"() -> (w644:dbl)
    n2025 = Greater Or Equal?(x=w1070, y=4.0) -> (x >= y?=w1060:bool)
    n2026 = Greater Or Equal?(x=w353, y=6.0) -> (x >= y?=w363:bool)
    n2027 = local read "EP"() -> (w663:dbl)
    n2028 = Greater Or Equal?(x=w1071, y=2.0) -> (x >= y?=w1081:bool)
    n2029 = local read "EP"() -> (w689:dbl)
    n2030 = Greater Or Equal?(x=w1053, y=5.0) -> (x >= y?=w1055:bool)
    n2031 = local read "EP"() -> (w702:dbl)
    n2032 = Greater Or Equal?(x=w1275, y=3.0) -> (x >= y?=w1273:bool)
    n2033 = local read "EP"() -> (w682:dbl)
    n2034 = Greater Or Equal?(x=w1797, y=4.0) -> (x >= y?=w1796:bool)
    n2035 = Greater Or Equal?(x=w1298, y=2.0) -> (x >= y?=w1300:bool)
    n2036 = local read "Military\nScience level"() -> (w380:i32)
    n2037 = Greater Or Equal?(x=w1096, y=1.0) -> (x >= y?=w1086:bool)
    n2038 = local read "SP"() -> (w1206:dbl)
    n2039 = local read "EP"() -> (w1066:dbl)
    n2040 = local read "EP"() -> (w357:dbl)
    n2041 = local read "SP"() -> (w1193:dbl)
    n2042 = local read "SP"() -> (w1179:dbl)
    n2043 = local read "Spear level"() -> (w1810:i32)
    n2044 = local read "EP"() -> (w1075:dbl)
    n2045 = local read "EP"() -> (w769:dbl)
    n2046 = Greater Or Equal?(x=w1042, y=5.0) -> (x >= y?=w1054:bool)
    n2047 = local read "EP"() -> (w782:dbl)
    n2048 = Greater Or Equal?(x=w1286, y=3.0) -> (x >= y?=w1274:bool)
    n2049 = local read "EP"() -> (w789:dbl)
    n2050 = Greater Or Equal?(x=w1287, y=2.0) -> (x >= y?=w1299:bool)
    n2051 = local read "EP"() -> (w1092:dbl)
    n2052 = local read "Physics level"() -> (w372:i32)
    n2053 = Greater Or Equal?(x=w631, y=w632) -> (x >= y?=w636:bool)
    n2054 = Greater Or Equal?(x=w644, y=w643) -> (x >= y?=w639:bool)
    n2055 = Subtract(x=w631, y=w632) -> (x-y=w633:dbl)
    n2056 = Subtract(x=w644, y=w643) -> (x-y=w642:dbl)
    n2057 = Equal?(x=w629, y=5.0) -> (x = y?=w634:bool)
    n2058 = local read "EP"() -> (w1046:dbl)
    n2059 = Greater Or Equal?(x=w663, y=w664) -> (x >= y?=w668:bool)
    n2060 = Compound Arithmetic op=AND(w634, "Rocket artillery", w625, w622, w636) -> (w637:bool)
    n2061 = local read "EP"() -> (w1805:dbl)
    n2062 = Equal?(x=w646, y=4.0) -> (x = y?=w641:bool)
    n2063 = Compound Arithmetic op=AND(w641, "Howitzer", w650, w653, w639) -> (w638:bool)
    n2064 = Increment(x=w629) -> (x+1=w630:i32)
    n2065 = local read "EP"() -> (w1282:dbl)
    n2066 = Greater Or Equal?(x=w689, y=w690) -> (x >= y?=w694:bool)
    n2067 = Subtract(x=w663, y=w664) -> (x-y=w665:dbl)
    n2068 = Greater Or Equal?(x=w702, y=w701) -> (x >= y?=w697:bool)
    n2069 = Increment(x=w646) -> (x+1=w645:i32)
    n2070 = Equal?(x=w661, y=3.0) -> (x = y?=w666:bool)
    n2071 = Subtract(x=w689, y=w690) -> (x-y=w691:dbl)
    n2072 = Compound Arithmetic op=AND(w666, "Cannon", w657, w654, w668) -> (w669:bool)
    n2073 = local read "EP"() -> (w1291:dbl)
    n2074 = Greater Or Equal?(x=w682, y=w681) -> (x >= y?=w677:bool)
    n2075 = Subtract(x=w702, y=w701) -> (x-y=w700:dbl)
    n2076 = Equal?(x=w687, y=1.0) -> (x = y?=w692:bool)
    n2077 = Increment(x=w661) -> (x+1=w662:i32)
    n2078 = Compound Arithmetic op=AND(w692, "Catapult", w671, w714, w694) -> (w695:bool)
    n2079 = Equal?(x=w704, y=2.0) -> (x = y?=w699:bool)
    n2080 = And(x="Iron\nSpear", y=w1796) -> (x .and. y?=w1794:bool)
    n2081 = Subtract(x=w682, y=w681) -> (x-y=w680:dbl)
    n2082 = Compound Arithmetic op=AND(w699, "Trebuchet", w708, w717, w697) -> (w696:bool)
    n2083 = Increment(x=w687) -> (x+1=w688:i32)
    n2084 = Equal?(x=w684, y=0.0) -> (x = y?=w679:bool)
    n2085 = Increment(x=w704) -> (x+1=w703:i32)
    n2086 = Compound Arithmetic op=AND(w679, "Ballista", w670, w711, w677) -> (w676:bool)
    n2087 = Increment(x=w684) -> (x+1=w683:i32)
    n2088 = Greater Or Equal?(x=w1066, y=w1065) -> (x >= y?=w1059:bool)
    n2089 = Greater Or Equal?(x=w357, y=w358) -> (x >= y?=w364:bool)
    n2090 = Greater Or Equal?(x=w1200, y=4) -> (x >= y?=w1209:bool)
    n2091 = Greater Or Equal?(x=w1206, y=5000000) -> (x >= y?=w1208:bool)
    n2092 = Subtract(x=w1066, y=w1065) -> (x-y=w1064:dbl)
    n2093 = Subtract(x=w357, y=w358) -> (x-y=w359:dbl)
    n2094 = Greater Or Equal?(x=w1075, y=w1076) -> (x >= y?=w1082:bool)
    n2095 = Equal?(x=w1068, y=2.0) -> (x = y?=w1063:bool)
    n2096 = Equal?(x=w355, y=3.0) -> (x = y?=w360:bool)
    n2097 = Greater Or Equal?(x=w769, y=w770) -> (x >= y?=w774:bool)
    n2098 = Compound Arithmetic op=AND(w1063, "Medicine 3", w1060, w1059) -> (w1058:bool)
    n2099 = Compound Arithmetic op=AND(w360, "Medicine 4", w363, w364) -> (w365:bool)
    n2100 = Greater Or Equal?(x=w1187, y=4) -> (x >= y?=w1196:bool)
    n2101 = Subtract(x=w1075, y=w1076) -> (x-y=w1077:dbl)
    n2102 = Greater Or Equal?(x=w1185, y=4) -> (x >= y?=w1176:bool)
    n2103 = Increment(x=w1068) -> (x+1=w1067:i32)
    n2104 = Increment(x=w355) -> (x+1=w356:i32)
    n2105 = Greater Or Equal?(x=w782, y=w781) -> (x >= y?=w777:bool)
    n2106 = Subtract(x=w769, y=w770) -> (x-y=w771:dbl)
    n2107 = Greater Or Equal?(x=w1193, y=5000000) -> (x >= y?=w1195:bool)
    n2108 = Equal?(x=w1073, y=1.0) -> (x = y?=w1078:bool)
    n2109 = Greater Or Equal?(x=w1179, y=5000000) -> (x >= y?=w1177:bool)
    n2110 = Compound Arithmetic op=AND(w1078, "Medicine 2", w1081, w1082) -> (w1083:bool)
    n2111 = Equal?(x=w767, y=2.0) -> (x = y?=w772:bool)
    n2112 = Subtract(x=w782, y=w781) -> (x-y=w780:dbl)
    n2113 = Compound Arithmetic op=AND(w772, "Income tax", w802, w774) -> (w775:bool)
    n2114 = Increment(x=w1073) -> (x+1=w1074:i32)
    n2115 = Greater Or Equal?(x=w789, y=w790) -> (x >= y?=w794:bool)
    n2116 = Equal?(x=w784, y=1.0) -> (x = y?=w779:bool)
    n2117 = Increment(x=w767) -> (x+1=w768:i32)
    n2118 = Compound Arithmetic op=AND(w779, "Sales tax", w803, w777) -> (w776:bool)
    n2119 = Greater Or Equal?(x=w1092, y=w1091) -> (x >= y?=w1085:bool)
    n2120 = Subtract(x=w789, y=w790) -> (x-y=w791:dbl)
    n2121 = Increment(x=w784) -> (x+1=w783:i32)
    n2122 = Equal?(x=w787, y=0.0) -> (x = y?=w792:bool)
    n2123 = Subtract(x=w1092, y=w1091) -> (x-y=w1090:dbl)
    n2124 = Compound Arithmetic op=AND(w792, "Tariffs", w804, w794) -> (w795:bool)
    n2125 = Not Equal?(x=w1205, y=w1211) -> (x != y?=w1203:bool)
    n2126 = Equal?(x=w1094, y=0.0) -> (x = y?=w1089:bool)
    n2127 = Increment(x=w787) -> (x+1=w788:i32)
    n2128 = Compound Arithmetic op=AND(w1089, "Medicine 1", w1086, w1085) -> (w1084:bool)
    n2129 = Greater Or Equal?(x=w1805, y=w1793) -> (x >= y?=w1804:bool)
    n2130 = And(x=w1794, y=w1804) -> (x .and. y?=w1807:bool)
    n2131 = Increment(x=w1094) -> (x+1=w1093:i32)
    n2132 = Not Equal?(x=w1192, y=w1198) -> (x != y?=w1190:bool)
    n2133 = Not Equal?(x=w1180, y=w1174) -> (x != y?=w1182:bool)
    n2134 = Greater Or Equal?(x=w1046, y=w1047) -> (x >= y?=w1056:bool)
    n2135 = Greater Or Equal?(x=w1282, y=w1281) -> (x >= y?=w1272:bool)
    n2136 = Subtract(x=w1046, y=w1047) -> (x-y=w1048:dbl)
    n2137 = case shown="True" w637 {
      tunnel: w630 -> [_ w2175]
      tunnel: w633 -> [_ w2174]
      frame False {
      }
      frame True {
        n2138 = local write "EP"(w2174) -> ()
        n2139 = local read "warrior b"() -> (w2171:dbl)
        n2140 = local write "Siege weapon\nlevel"(w2175) -> ()
        n2141 = Add(x=w2171, y=1.0) -> (x+y=w2172:dbl)
        n2142 = local write "warrior b"(w2172) -> ()
      }
    }
    n2143 = Equal?(x=w1044, y=2.0) -> (x = y?=w1049:bool)
    n2144 = case shown="True" w676 {
      tunnel: w683 -> [_ w2200]
      tunnel: w680 -> [_ w2199]
      frame False {
      }
      frame True {
        n2145 = local write "Siege weapon\nlevel"(w2200) -> ()
        n2146 = local write "EP"(w2199) -> ()
        n2147 = local read "warrior b"() -> (w2198:dbl)
        n2148 = Add(x=w2198, y=0.25) -> (x+y=w2197:dbl)
        n2149 = local write "warrior b"(w2197) -> ()
      }
    }
    n2150 = Subtract(x=w1282, y=w1281) -> (x-y=w1280:dbl)
    n2151 = Compound Arithmetic op=AND(w1049, "Advanced\nmetal\ntools", w1054, w1055, w1056) -> (w1057:bool)
    n2152 = case shown="True" w638 {
      tunnel: w645 -> [_ w2180]
      tunnel: w642 -> [_ w2179]
      frame False {
      }
      frame True {
        n2153 = local write "EP"(w2179) -> ()
        n2154 = local read "warrior b"() -> (w2176:dbl)
        n2155 = local write "Siege weapon\nlevel"(w2180) -> ()
        n2156 = Add(x=w2176, y=1.0) -> (x+y=w2177:dbl)
        n2157 = local write "warrior b"(w2177) -> ()
      }
    }
    n2158 = Greater Or Equal?(x=w1291, y=w1292) -> (x >= y?=w1301:bool)
    n2159 = Equal?(x=w1284, y=1.0) -> (x = y?=w1279:bool)
    n2160 = Increment(x=w1044) -> (x+1=w1045:i32)
    n2161 = Compound Arithmetic op=AND(w1279, "Basic\nmetal\ntools", w1274, w1273, w1272) -> (w1271:bool)
    n2162 = Subtract(x=w1291, y=w1292) -> (x-y=w1293:dbl)
    n2163 = case shown="True" w669 {
      tunnel: w662 -> [_ w2185]
      tunnel: w665 -> [_ w2184]
      frame False {
      }
      frame True {
        n2164 = local write "EP"(w2184) -> ()
        n2165 = local read "warrior b"() -> (w2181:dbl)
        n2166 = local write "Siege weapon\nlevel"(w2185) -> ()
        n2167 = Add(x=w2181, y=1.0) -> (x+y=w2182:dbl)
        n2168 = local write "warrior b"(w2182) -> ()
      }
    }
    n2169 = Increment(x=w1284) -> (x+1=w1283:i32)
    n2170 = Equal?(x=w1289, y=0.0) -> (x = y?=w1294:bool)
    n2171 = Equal?(x=w1810, y=3.0) -> (x = y?=w1808:bool)
    n2172 = And(x=w1808, y=w1807) -> (x .and. y?=w1809:bool)
    n2173 = Compound Arithmetic op=AND(w1294, "Stone tools", w1299, w1300, w1301) -> (w1302:bool)
    n2174 = case shown="True" w695 {
      tunnel: w688 -> [_ w2195]
      tunnel: w691 -> [_ w2194]
      frame False {
      }
      frame True {
        n2175 = local write "EP"(w2194) -> ()
        n2176 = local read "warrior b"() -> (w2191:dbl)
        n2177 = local write "Siege weapon\nlevel"(w2195) -> ()
        n2178 = Add(x=w2191, y=0.5) -> (x+y=w2192:dbl)
        n2179 = local write "warrior b"(w2192) -> ()
      }
    }
    n2180 = case shown="True" w1058 {
      tunnel: w1067 -> [_ w2325]
      tunnel: w1064 -> [_ w2324]
      frame False {
      }
      frame True {
        n2181 = local write "EP"(w2324) -> ()
        n2182 = local write "Medicine level"(w2325) -> ()
        n2183 = local write "Medicine dissent mod"(0.9 ("Medicine dissent mod")) -> ()
      }
    }
    n2184 = case shown="True" w365 {
      tunnel: w356 -> [_ w2063]
      tunnel: w359 -> [_ w2062]
      frame False {
      }
      frame True {
        n2185 = local write "EP"(w2062) -> ()
        n2186 = local write "Medicine level"(w2063) -> ()
        n2187 = local write "Medicine dissent mod"(0.85 ("Medicine dissent mod")) -> ()
      }
    }
    n2188 = case shown="True" w696 {
      tunnel: w703 -> [_ w2190]
      tunnel: w700 -> [_ w2189]
      frame False {
      }
      frame True {
        n2189 = local write "EP"(w2189) -> ()
        n2190 = local read "warrior b"() -> (w2188:dbl)
        n2191 = local write "Siege weapon\nlevel"(w2190) -> ()
        n2192 = Add(x=w2188, y=0.5) -> (x+y=w2187:dbl)
        n2193 = local write "warrior b"(w2187) -> ()
      }
    }
    n2194 = Increment(x=w1289) -> (x+1=w1290:i32)
    n2195 = case shown="True" w1083 {
      tunnel: w1074 -> [_ w2328]
      tunnel: w1077 -> [_ w2327]
      frame False {
      }
      frame True {
        n2196 = local write "EP"(w2327) -> ()
        n2197 = local write "Medicine level"(w2328) -> ()
        n2198 = local write "Medicine dissent mod"(0.95 ("Medicine dissent mod")) -> ()
      }
    }
    n2199 = And(x=w1209, y=w1208) -> (x .and. y?=w1210:bool)
    n2200 = And(x="Feudalism", y=w1210) -> (x .and. y?=w1202:bool)
    n2201 = And(x=w1203, y=w1202) -> (x .and. y?=w1204:bool)
    n2202 = And(x=w1196, y=w1195) -> (x .and. y?=w1197:bool)
    n2203 = And(x="Caste system", y=w1197) -> (x .and. y?=w1189:bool)
    n2204 = And(x=w1190, y=w1189) -> (x .and. y?=w1191:bool)
    n2205 = And(x=w1176, y=w1177) -> (x .and. y?=w1175:bool)
    n2206 = And(x="Senate", y=w1175) -> (x .and. y?=w1183:bool)
    n2207 = And(x=w1182, y=w1183) -> (x .and. y?=w1181:bool)
    n2208 = case shown="True" w795 {
      tunnel: w788 -> [_ w2220]
      tunnel: w791 -> [_ w2219]
      frame False {
      }
      frame True {
        n2209 = local write "EP"(w2219) -> ()
        n2210 = local write "Tax method\nlevel"(w2220) -> ()
      }
    }
    n2211 = case shown="True" w1204 {
      tunnel: w1211 -> [_ w2387]
      frame False {
      }
      frame True {
        n2212 = local write "Government"(w2387) -> ()
        n2213 = local read "SP"() -> (w2384:dbl)
        n2214 = Subtract(x=w2384, y=5000000) -> (x-y=w2386:dbl)
        n2215 = local write "SP"(w2386) -> ()
      }
    }
    n2216 = case shown="True" w1084 {
      tunnel: w1093 -> [_ w2331]
      tunnel: w1090 -> [_ w2330]
      frame False {
      }
      frame True {
        n2217 = local write "EP"(w2330) -> ()
        n2218 = local write "Medicine level"(w2331) -> ()
        n2219 = local write "Medicine dissent mod"(0.97 ("Medicine dissent mod")) -> ()
      }
    }
    n2220 = local read "SP"() -> (w1688:dbl)
    n2221 = case shown="True" w775 {
      tunnel: w768 -> [_ w2216]
      tunnel: w771 -> [_ w2215]
      frame False {
      }
      frame True {
        n2222 = local write "EP"(w2215) -> ()
        n2223 = local write "Tax method\nlevel"(w2216) -> ()
      }
    }
    n2224 = local read "SP"() -> (w1706:dbl)
    n2225 = case shown="True" w1191 {
      tunnel: w1198 -> [_ w2383]
      frame False {
      }
      frame True {
        n2226 = local write "Government"(w2383) -> ()
        n2227 = local read "SP"() -> (w2382:dbl)
        n2228 = Subtract(x=w2382, y=5000000) -> (x-y=w2380:dbl)
        n2229 = local write "SP"(w2380) -> ()
      }
    }
    n2230 = case shown="True" w1181 {
      tunnel: w1174 -> [_ w2379]
      frame False {
      }
      frame True {
        n2231 = local write "Government"(w2379) -> ()
        n2232 = local read "SP"() -> (w2376:dbl)
        n2233 = Subtract(x=w2376, y=5000000) -> (x-y=w2378:dbl)
        n2234 = local write "SP"(w2378) -> ()
      }
    }
    n2235 = case shown="True" w776 {
      tunnel: w783 -> [_ w2218]
      tunnel: w780 -> [_ w2217]
      frame False {
      }
      frame True {
        n2236 = local write "EP"(w2217) -> ()
        n2237 = local write "Tax method\nlevel"(w2218) -> ()
      }
    }
    n2238 = Power Of 10(x=w1690) -> (10^x=w1685:dbl)
    n2239 = Power Of 10(x=w1704) -> (10^x=w1710:dbl)
    n2240 = Increment(x=w1810) -> (x+1=w1811:i32)
    n2241 = case shown="True" w1302 {
      tunnel: w1290 -> [_ w2411]
      tunnel: w1293 -> [_ w2410]
      frame False {
      }
      frame True {
        n2242 = local read "Construction multiplier"() -> (w2408:dbl)
        n2243 = local write "Construction\ntools level"(w2411) -> ()
        n2244 = local write "EP"(w2410) -> ()
        n2245 = Add(x=w2408, y=0.5) -> (x+y=w2407:dbl)
        n2246 = local write "Construction multiplier"(w2407) -> ()
      }
    }
    n2247 = case shown="True" w1809 {
      tunnel: w1805 -> [_ w2769]
      tunnel: w1811 -> [_ w2767]
      tunnel: w1793 -> [_ w2766]
      frame False {
      }
      frame True {
        n2248 = local read "warrior a"() -> (w2771:dbl)
        n2249 = local write "Spear level"(w2767) -> ()
        n2250 = Subtract(x=w2769, y=w2766) -> (x-y=w2768:dbl)
        n2251 = local write "EP"(w2768) -> ()
        n2252 = Add(x=w2771, y=0.5) -> (x+y=w2770:dbl)
        n2253 = local write "warrior a"(w2770) -> ()
      }
    }
    n2254 = case shown="True" w1057 {
      tunnel: w1045 -> [_ w2322]
      tunnel: w1048 -> [_ w2321]
      frame False {
      }
      frame True {
        n2255 = local read "Construction multiplier"() -> (w2319:dbl)
        n2256 = local write "Construction\ntools level"(w2322) -> ()
        n2257 = local write "EP"(w2321) -> ()
        n2258 = Add(x=w2319, y=1.0) -> (x+y=w2320:dbl)
        n2259 = local write "Construction multiplier"(w2320) -> ()
      }
    }
    n2260 = case shown="True" w1271 {
      tunnel: w1283 -> [_ w2406]
      tunnel: w1280 -> [_ w2405]
      frame False {
      }
      frame True {
        n2261 = local read "Construction multiplier"() -> (w2403:dbl)
        n2262 = local write "Construction\ntools level"(w2406) -> ()
        n2263 = local write "EP"(w2405) -> ()
        n2264 = Add(x=w2403, y=0.5) -> (x+y=w2404:dbl)
        n2265 = local write "Construction multiplier"(w2404) -> ()
      }
    }
    n2266 = Greater Or Equal?(x=w372, y=5.0) -> (x >= y?=w370:bool)
    n2267 = local read "Bow level"() -> (w367:i32)
    n2268 = Greater Or Equal?(x=w380, y=6.0) -> (x >= y?=w371:bool)
    n2269 = Increment(x=w1690) -> (x+1=w1534:i32)
    n2270 = Index Array(array=w608, index=w1534) -> (element=w1533:dbl)
    n2271 = Power Of 2(x=w1533) -> (2^x=w1532:dbl)
    n2272 = Compound Arithmetic op=MULTIPLY(w1685, 1000, w1532) -> (w1689:dbl)
    n2273 = Greater?(x=w1688, y=w1689) -> (0:w1687:bool)
    n2274 = And(x="Biology", y=w1687) -> (x .and. y?=w1569:bool)
    n2275 = local read "EP"() -> (w378:dbl)
    n2276 = Increment(x=w1704) -> (x+1=w1537:i32)
    n2277 = Index Array(array=w608, index=w1537) -> (element=w1536:dbl)
    n2278 = Power Of 2(x=w1536) -> (2^x=w1535:dbl)
    n2279 = Compound Arithmetic op=MULTIPLY(w1710, 1000, w1535) -> (w1705:dbl)
    n2280 = Greater?(x=w1706, y=w1705) -> (0:w1708:bool)
    n2281 = And(x="Economics", y=w1708) -> (x .and. y?=w1707:bool)
    n2282 = case shown="True" w1569 {
      tunnel: w1688 -> [_ w2712]
      tunnel: w1689 -> [_ w2711]
      tunnel: w1534 -> [_ w2709]
      tunnel: [0 w2709] -> w1570
      frame False {
      }
      frame True {
        n2283 = Subtract(x=w2712, y=w2711) -> (x-y=w2710:dbl)
        n2284 = local write "SP"(w2710) -> ()
        n2285 = local write "Biology\nlevel"(w2709) -> ()
      }
    }
    n2286 = case shown="True" w1707 {
      selector: w1707 -> [w2721 w2724]
      tunnel: w1706 -> [_ w2727]
      tunnel: w1705 -> [_ w2726]
      tunnel: w1537 -> [_ w2723]
      tunnel: [w2721 w2724] -> w1568
      tunnel: [0 w2723] -> w1571
      frame False {
      }
      frame True {
        n2287 = Subtract(x=w2727, y=w2726) -> (x-y=w2725:dbl)
        n2288 = local write "SP"(w2725) -> ()
        n2289 = local write "Economics\nlevel"(w2723) -> ()
      }
    }
    n2290 = Compound Arithmetic op=OR(w1564, w1565, w1566, w1567, w1568, w1569) -> (w1576:bool)
    n2291 = Greater Or Equal?(x=w378, y=w313) -> (x >= y?=w369:bool)
    n2292 = Subtract(x=w378, y=w313) -> (x-y=w377:dbl)
    n2293 = Equal?(x=w367, y=3.0) -> (x = y?=w376:bool)
    n2294 = Compound Arithmetic op=AND(w376, "Crossbow", w371, w370, w369) -> (w368:bool)
    n2295 = Increment(x=w367) -> (x+1=w366:i32)
    n2296 = case shown="True" w368 {
      tunnel: w366 -> [_ w2068]
      tunnel: w377 -> [_ w2067]
      frame False {
      }
      frame True {
        n2297 = local write "EP"(w2067) -> ()
        n2298 = local read "warrior a"() -> (w2065:dbl)
        n2299 = local write "Bow level"(w2068) -> ()
        n2300 = Add(x=0.25, y=w2065) -> (x+y=w2066:dbl)
        n2301 = local write "warrior a"(w2066) -> ()
      }
    }
    n2302 = local read "Military\nScience level"() -> (w810:i32)
    n2303 = local read "Military\nScience level"() -> (w809:i32)
    n2304 = local read "Biology\nlevel"() -> (w821:i32)
    n2305 = local read "Biology\nlevel"() -> (w816:i32)
    n2306 = local read "Physics level"() -> (w720:i32)
    n2307 = local read "Military\nScience level"() -> (w763:i32)
    n2308 = local read "Physics level"() -> (w722:i32)
    n2309 = local read "Military\nScience level"() -> (w813:i32)
    n2310 = local read "Biology\nlevel"() -> (w819:i32)
    n2311 = local read "Physics level"() -> (w726:i32)
    n2312 = local read "Military\nScience level"() -> (w760:i32)
    n2313 = local read "Economics\nlevel"() -> (w728:i32)
    n2314 = local read "Production\nlevel"() -> (w611:i32)
    n2315 = local read "Animal\ndomestication\nlevel"() -> (w854:i32)
    n2316 = local read "Animal\ndomestication\nlevel"() -> (w871:i32)
    n2317 = local read "Animal\ndomestication\nlevel"() -> (w874:i32)
    n2318 = local read "Writing level"() -> (w911:i32)
    n2319 = local read "Writing level"() -> (w344:i32)
    n2320 = local read "Writing level"() -> (w894:i32)
    n2321 = local read "Writing level"() -> (w891:i32)
    n2322 = local read "Sword level"() -> (w851:i32)
    n2323 = local read "Sword level"() -> (w834:i32)
    n2324 = local read "Chariot level"() -> (w748:i32)
    n2325 = local read "Chariot level"() -> (w731:i32)
    n2326 = local read "Sword level"() -> (w831:i32)
    n2327 = local read "Chariot level"() -> (w751:i32)
    n2328 = Greater Or Equal?(x=w821, y=1.0) -> (x >= y?=w820:bool)
    n2329 = Greater Or Equal?(x=w816, y=3.0) -> (x >= y?=w814:bool)
    n2330 = Greater Or Equal?(x=w720, y=4.0) -> (x >= y?=w718:bool)
    n2331 = Greater Or Equal?(x=w722, y=4.0) -> (x >= y?=w721:bool)
    n2332 = Greater Or Equal?(x=w819, y=2.0) -> (x >= y?=w815:bool)
    n2333 = Greater Or Equal?(x=w726, y=3.0) -> (x >= y?=w724:bool)
    n2334 = Greater Or Equal?(x=w810, y=4.0) -> (x >= y?=w806:bool)
    n2335 = Greater Or Equal?(x=w809, y=6.0) -> (x >= y?=w807:bool)
    n2336 = Greater Or Equal?(x=w763, y=3.0) -> (x >= y?=w764:bool)
    n2337 = Greater Or Equal?(x=w728, y=4.0) -> (x >= y?=w727:bool)
    n2338 = local read "EP"() -> (w909:dbl)
    n2339 = local read "EP"() -> (w346:dbl)
    n2340 = Greater Or Equal?(x=w813, y=3.0) -> (x >= y?=w805:bool)
    n2341 = local read "EP"() -> (w896:dbl)
    n2342 = local read "SP"() -> (w613:dbl)
    n2343 = local read "EP"() -> (w889:dbl)
    n2344 = Greater Or Equal?(x=w760, y=3.0) -> (x >= y?=w765:bool)
    n2345 = Power Of 10(x=w611) -> (10^x=w616:dbl)
    n2346 = local read "EP"() -> (w856:dbl)
    n2347 = local read "EP"() -> (w869:dbl)
    n2348 = local read "EP"() -> (w876:dbl)
    n2349 = local read "EP"() -> (w849:dbl)
    n2350 = local read "EP"() -> (w836:dbl)
    n2351 = local read "EP"() -> (w829:dbl)
    n2352 = local read "EP"() -> (w746:dbl)
    n2353 = local read "EP"() -> (w733:dbl)
    n2354 = local read "EP"() -> (w753:dbl)
    n2355 = Greater Or Equal?(x=w909, y=w908) -> (x >= y?=w904:bool)
    n2356 = Greater Or Equal?(x=w346, y=w347) -> (x >= y?=w351:bool)
    n2357 = Greater Or Equal?(x=w896, y=w897) -> (x >= y?=w901:bool)
    n2358 = Subtract(x=w909, y=w908) -> (x-y=w907:dbl)
    n2359 = Subtract(x=w346, y=w347) -> (x-y=w348:dbl)
    n2360 = Equal?(x=w911, y=2.0) -> (x = y?=w906:bool)
    n2361 = Equal?(x=w344, y=3.0) -> (x = y?=w349:bool)
    n2362 = Subtract(x=w896, y=w897) -> (x-y=w898:dbl)
    n2363 = Compound Arithmetic op=AND(w906, "Movable typeset", w904) -> (w903:bool)
    n2364 = Compound Arithmetic op=AND(w349, "Printing\nPress", w351) -> (w352:bool)
    n2365 = Greater Or Equal?(x=w889, y=w888) -> (x >= y?=w884:bool)
    n2366 = Equal?(x=w894, y=1.0) -> (x = y?=w899:bool)
    n2367 = Increment(x=w911) -> (x+1=w910:i32)
    n2368 = Increment(x=w344) -> (x+1=w345:i32)
    n2369 = Compound Arithmetic op=AND(w899, "Paper", w901) -> (w902:bool)
    n2370 = Subtract(x=w889, y=w888) -> (x-y=w887:dbl)
    n2371 = Greater Or Equal?(x=w856, y=w857) -> (x >= y?=w861:bool)
    n2372 = Increment(x=w894) -> (x+1=w895:i32)
    n2373 = Equal?(x=w891, y=0.0) -> (x = y?=w886:bool)
    n2374 = Compound Arithmetic op=AND(w886, "Parchment", w884) -> (w883:bool)
    n2375 = Greater Or Equal?(x=w869, y=w868) -> (x >= y?=w864:bool)
    n2376 = Increment(x=w891) -> (x+1=w890:i32)
    n2377 = Equal?(x=w854, y=2.0) -> (x = y?=w859:bool)
    n2378 = Subtract(x=w856, y=w857) -> (x-y=w858:dbl)
    n2379 = Subtract(x=w869, y=w868) -> (x-y=w867:dbl)
    n2380 = Compound Arithmetic op=AND(w859, "Selective\nbreeding", w814, w861) -> (w862:bool)
    n2381 = Greater Or Equal?(x=w876, y=w877) -> (x >= y?=w881:bool)
    n2382 = Equal?(x=w871, y=1.0) -> (x = y?=w866:bool)
    n2383 = Increment(x=w854) -> (x+1=w855:i32)
    n2384 = Compound Arithmetic op=AND(w866, "Horses", w864, w815) -> (w863:bool)
    n2385 = Subtract(x=w876, y=w877) -> (x-y=w878:dbl)
    n2386 = Increment(x=w871) -> (x+1=w870:i32)
    n2387 = Equal?(x=w874, y=0.0) -> (x = y?=w879:bool)
    n2388 = Compound Arithmetic op=AND(w879, "Livestock", w881, w820) -> (w882:bool)
    n2389 = Increment(x=w611) -> (x+1=w618:i32)
    n2390 = Index Array(array=w608, index=w618) -> (element=w619:dbl)
    n2391 = Power Of 2(x=w619) -> (2^x=w620:dbl)
    n2392 = Compound Arithmetic op=MULTIPLY(w616, 1000, w620) -> (w612:dbl)
    n2393 = Greater?(x=w613, y=w612) -> (0:w614:bool)
    n2394 = And(x="Production", y=w614) -> (x .and. y?=w609:bool)
    n2395 = Increment(x=w874) -> (x+1=w875:i32)
    n2396 = Greater Or Equal?(x=w849, y=w848) -> (x >= y?=w844:bool)
    n2397 = Greater Or Equal?(x=w836, y=w837) -> (x >= y?=w841:bool)
    n2398 = Subtract(x=w849, y=w848) -> (x-y=w847:dbl)
    n2399 = Equal?(x=w851, y=2.0) -> (x = y?=w846:bool)
    n2400 = Subtract(x=w836, y=w837) -> (x-y=w838:dbl)
    n2401 = Compound Arithmetic op=AND(w846, "Steel sword", w807, w844) -> (w843:bool)
    n2402 = Greater Or Equal?(x=w829, y=w828) -> (x >= y?=w824:bool)
    n2403 = Equal?(x=w834, y=1.0) -> (x = y?=w839:bool)
    n2404 = Increment(x=w851) -> (x+1=w850:i32)
    n2405 = Compound Arithmetic op=AND(w839, "Iron sword", w806, w841) -> (w842:bool)
    n2406 = Subtract(x=w829, y=w828) -> (x-y=w827:dbl)
    n2407 = Greater Or Equal?(x=w746, y=w745) -> (x >= y?=w741:bool)
    n2408 = Increment(x=w834) -> (x+1=w835:i32)
    n2409 = Greater Or Equal?(x=w733, y=w734) -> (x >= y?=w738:bool)
    n2410 = Equal?(x=w831, y=0.0) -> (x = y?=w826:bool)
    n2411 = Compound Arithmetic op=AND(w826, "Bronze sword", w805, w824) -> (w823:bool)
    n2412 = Subtract(x=w746, y=w745) -> (x-y=w744:dbl)
    n2413 = Greater Or Equal?(x=w753, y=w754) -> (x >= y?=w758:bool)
    n2414 = Subtract(x=w733, y=w734) -> (x-y=w735:dbl)
    n2415 = Increment(x=w831) -> (x+1=w830:i32)
    n2416 = Equal?(x=w748, y=1.0) -> (x = y?=w743:bool)
    n2417 = Compound Arithmetic op=AND(w743, "Reinforced\nchariot", w764, w721, w741) -> (w740:bool)
    n2418 = Equal?(x=w731, y=2.0) -> (x = y?=w736:bool)
    n2419 = Subtract(x=w753, y=w754) -> (x-y=w755:dbl)
    n2420 = Compound Arithmetic op=AND(w736, "Caravan", w727, w718, w738) -> (w739:bool)
    n2421 = case shown="True" w883 {
      tunnel: w890 -> [_ w2262]
      tunnel: w887 -> [_ w2261]
      frame False {
      }
      frame True {
        n2422 = local write "EP"(w2261) -> ()
        n2423 = local write "Writing level"(w2262) -> ()
      }
    }
    n2424 = Increment(x=w748) -> (x+1=w747:i32)
    n2425 = Equal?(x=w751, y=0.0) -> (x = y?=w756:bool)
    n2426 = Increment(x=w731) -> (x+1=w732:i32)
    n2427 = Compound Arithmetic op=AND(w756, "Simple\nchariot", w765, w724, w758) -> (w759:bool)
    n2428 = Increment(x=w751) -> (x+1=w752:i32)
    n2429 = case shown="True" w882 {
      tunnel: w875 -> [_ w2256]
      tunnel: w878 -> [_ w2255]
      frame False {
      }
      frame True {
        n2430 = local write "Animal\ndomestication\nlevel"(w2256) -> ()
        n2431 = local read "hunting b"() -> (w2254:dbl)
        n2432 = local write "EP"(w2255) -> ()
        n2433 = Add(x=w2254, y=0.25) -> (x+y=w2253:dbl)
        n2434 = local write "hunting b"(w2253) -> ()
      }
    }
    n2435 = case shown="True" w903 {
      tunnel: w910 -> [_ w2258]
      tunnel: w907 -> [_ w2257]
      frame False {
      }
      frame True {
        n2436 = local write "EP"(w2257) -> ()
        n2437 = local write "Writing level"(w2258) -> ()
      }
    }
    n2438 = case shown="True" w352 {
      tunnel: w345 -> [_ w2060]
      tunnel: w348 -> [_ w2059]
      frame False {
      }
      frame True {
        n2439 = local write "EP"(w2059) -> ()
        n2440 = local write "Writing level"(w2060) -> ()
      }
    }
    n2441 = case shown="True" w862 {
      tunnel: w855 -> [_ w2243]
      tunnel: w858 -> [_ w2242]
      frame False {
      }
      frame True {
        n2442 = local write "Animal\ndomestication\nlevel"(w2243) -> ()
        n2443 = local read "warrior a"() -> (w2239:dbl)
        n2444 = local read "Construction multiplier"() -> (w2237:dbl)
        n2445 = local write "EP"(w2242) -> ()
        n2446 = Add(x=w2237, y=0.5) -> (x+y=w2238:dbl)
        n2447 = Add(x=w2239, y=0.25) -> (x+y=w2241:dbl)
        n2448 = local write "Construction multiplier"(w2238) -> ()
        n2449 = local write "warrior a"(w2241) -> ()
      }
    }
    n2450 = case shown="True" w902 {
      tunnel: w895 -> [_ w2260]
      tunnel: w898 -> [_ w2259]
      frame False {
      }
      frame True {
        n2451 = local write "EP"(w2259) -> ()
        n2452 = local write "Writing level"(w2260) -> ()
      }
    }
    n2453 = case shown="True" w863 {
      tunnel: w870 -> [_ w2251]
      tunnel: w867 -> [_ w2250]
      frame False {
      }
      frame True {
        n2454 = local write "Animal\ndomestication\nlevel"(w2251) -> ()
        n2455 = local write "EP"(w2250) -> ()
        n2456 = local read "warrior b"() -> (w2247:dbl)
        n2457 = local read "Construction multiplier"() -> (w2245:dbl)
        n2458 = Add(x=w2245, y=0.5) -> (x+y=w2244:dbl)
        n2459 = Add(x=w2247, y=0.25) -> (x+y=w2248:dbl)
        n2460 = local write "Construction multiplier"(w2244) -> ()
        n2461 = local write "warrior b"(w2248) -> ()
      }
    }
    n2462 = case shown="True" w609 {
      tunnel: w613 -> [_ w2170]
      tunnel: w612 -> [_ w2169]
      tunnel: w618 -> [_ w2167]
      tunnel: [0 w2167] -> w610
      frame False {
      }
      frame True {
        n2463 = Subtract(x=w2170, y=w2169) -> (x-y=w2168:dbl)
        n2464 = local write "SP"(w2168) -> ()
        n2465 = local write "Production\nlevel"(w2167) -> ()
      }
    }
    n2466 = case shown="True" w1576 {
      tunnel: w1575 -> [_ w2495]
      tunnel: w1574 -> [_ w2498]
      tunnel: w1573 -> [_ w2501]
      tunnel: w1572 -> [_ w2504]
      tunnel: w1571 -> [_ w2507]
      tunnel: w1570 -> [_ w2510]
      tunnel: w1569 -> [_ w2509]
      tunnel: w1568 -> [_ w2506]
      tunnel: w1567 -> [_ w2503]
      tunnel: w1566 -> [_ w2500]
      tunnel: w1565 -> [_ w2497]
      tunnel: w1564 -> [_ w2494]
      tunnel: w610 -> [_ w2483]
      tunnel: w609 -> [_ w2482]
      frame False {
      }
      frame True {
        n2467 = Boolean To (0,1)(Boolean=w2494) -> (0, 1=w2493:i16)
        n2468 = Boolean To (0,1)(Boolean=w2497) -> (0, 1=w2496:i16)
        n2469 = Boolean To (0,1)(Boolean=w2500) -> (0, 1=w2499:i16)
        n2470 = Boolean To (0,1)(Boolean=w2509) -> (0, 1=w2508:i16)
        n2471 = Boolean To (0,1)(Boolean=w2503) -> (0, 1=w2502:i16)
        n2472 = Boolean To (0,1)(Boolean=w2506) -> (0, 1=w2505:i16)
        n2473 = Boolean To (0,1)(Boolean=w2482) -> (0, 1=w2485:i16)
        n2474 = Multiply(x=w2493, y=w2495) -> (x*y=w2492:i32)
        n2475 = Multiply(x=w2496, y=w2498) -> (x*y=w2491:i32)
        n2476 = Multiply(x=w2499, y=w2501) -> (x*y=w2490:i32)
        n2477 = Multiply(x=w2508, y=w2510) -> (x*y=w2487:i32)
        n2478 = Multiply(x=w2502, y=w2504) -> (x*y=w2489:i32)
        n2479 = Multiply(x=w2505, y=w2507) -> (x*y=w2488:i32)
        n2480 = Multiply(x=w2485, y=w2483) -> (x*y=w2484:i32)
        n2481 = Compound Arithmetic op=ADD(w2492, w2491, w2490, w2489, w2488, w2487, w2484) -> (w2486:i32)
        n2482 = case shown="1" w2486 {
          frame 0, Default {
          }
          frame 1 {
            n2483 = local read "# of level 1 sciences"() -> (w2512:i32)
            n2484 = Increment(x=w2512) -> (x+1=w2511:i32)
            n2485 = local write "# of level 1 sciences"(w2511) -> ()
          }
          frame 2 {
            n2486 = local read "# of level 2 sciences"() -> (w2514:i32)
            n2487 = Increment(x=w2514) -> (x+1=w2513:i32)
            n2488 = local write "# of level 2 sciences"(w2513) -> ()
          }
          frame 3 {
            n2489 = local read "# of level 3 sciences"() -> (w2516:i32)
            n2490 = Increment(x=w2516) -> (x+1=w2515:i32)
            n2491 = local write "# of level 3 sciences"(w2515) -> ()
          }
          frame 4 {
            n2492 = local read "# of level 4 sciences"() -> (w2518:i32)
            n2493 = Increment(x=w2518) -> (x+1=w2517:i32)
            n2494 = local write "# of level 4 sciences"(w2517) -> ()
          }
          frame 5 {
            n2495 = local read "# of level 5 sciences"() -> (w2520:i32)
            n2496 = Increment(x=w2520) -> (x+1=w2519:i32)
            n2497 = local write "# of level 5 sciences"(w2519) -> ()
          }
          frame 6 {
            n2498 = local read "# of level 6 sciences"() -> (w2522:i32)
            n2499 = Increment(x=w2522) -> (x+1=w2521:i32)
            n2500 = local write "# of level 6 sciences"(w2521) -> ()
          }
          frame 7 {
            n2501 = local read "# of level 7 sciences"() -> (w2524:i32)
            n2502 = Increment(x=w2524) -> (x+1=w2523:i32)
            n2503 = local write "# of level 7 sciences"(w2523) -> ()
          }
          frame 8 {
            n2504 = local read "# of level 8 sciences"() -> (w2526:i32)
            n2505 = Increment(x=w2526) -> (x+1=w2525:i32)
            n2506 = local write "# of level 8 sciences"(w2525) -> ()
          }
          frame 9 {
            n2507 = local read "# of level 9 sciences"() -> (w2528:i32)
            n2508 = Increment(x=w2528) -> (x+1=w2527:i32)
            n2509 = local write "# of level 9 sciences"(w2527) -> ()
          }
          frame 10 {
            n2510 = local read "# of level 10 sciences"() -> (w2530:i32)
            n2511 = Increment(x=w2530) -> (x+1=w2529:i32)
            n2512 = local write "# of level 10 sciences"(w2529) -> ()
          }
        }
      }
    }
    n2513 = case shown="True" w823 {
      tunnel: w830 -> [_ w2235]
      tunnel: w827 -> [_ w2234]
      frame False {
      }
      frame True {
        n2514 = local write "EP"(w2234) -> ()
        n2515 = local read "warrior b"() -> (w2233:dbl)
        n2516 = local write "Sword level"(w2235) -> ()
        n2517 = Add(x=w2233, y=0.25) -> (x+y=w2231:dbl)
        n2518 = local write "warrior b"(w2231) -> ()
      }
    }
    n2519 = case shown="True" w843 {
      tunnel: w850 -> [_ w2225]
      tunnel: w847 -> [_ w2224]
      frame False {
      }
      frame True {
        n2520 = local read "warrior a"() -> (w2221:dbl)
        n2521 = local write "EP"(w2224) -> ()
        n2522 = local write "Sword level"(w2225) -> ()
        n2523 = Add(x=w2221, y=0.25) -> (x+y=w2223:dbl)
        n2524 = local write "warrior a"(w2223) -> ()
      }
    }
    n2525 = case shown="True" w759 {
      tunnel: w752 -> [_ w2214]
      tunnel: w755 -> [_ w2213]
      frame False {
      }
      frame True {
        n2526 = local write "EP"(w2213) -> ()
        n2527 = local read "warrior b"() -> (w2212:dbl)
        n2528 = local write "Chariot level"(w2214) -> ()
        n2529 = Add(x=w2212, y=0.25) -> (x+y=w2211:dbl)
        n2530 = local write "warrior b"(w2211) -> ()
      }
    }
    n2531 = case shown="True" w842 {
      tunnel: w835 -> [_ w2230]
      tunnel: w838 -> [_ w2229]
      frame False {
      }
      frame True {
        n2532 = local write "EP"(w2229) -> ()
        n2533 = local read "warrior a"() -> (w2226:dbl)
        n2534 = local write "Sword level"(w2230) -> ()
        n2535 = Add(x=w2226, y=0.25) -> (x+y=w2227:dbl)
        n2536 = local write "warrior a"(w2227) -> ()
      }
    }
    n2537 = case shown="True" w740 {
      tunnel: w747 -> [_ w2209]
      tunnel: w744 -> [_ w2208]
      frame False {
      }
      frame True {
        n2538 = local write "EP"(w2208) -> ()
        n2539 = local read "warrior a"() -> (w2205:dbl)
        n2540 = local write "Chariot level"(w2209) -> ()
        n2541 = Add(x=w2205, y=0.25) -> (x+y=w2206:dbl)
        n2542 = local write "warrior a"(w2206) -> ()
      }
    }
    n2543 = case shown="True" w739 {
      tunnel: w732 -> [_ w2204]
      tunnel: w735 -> [_ w2203]
      frame False {
      }
      frame True {
        n2544 = local read "Trading level no mod"() -> (w2202:i32)
        n2545 = local write "EP"(w2203) -> ()
        n2546 = local write "Chariot level"(w2204) -> ()
        n2547 = Increment(x=w2202) -> (x+1=w2201:i32)
        n2548 = local write "Trading level no mod"(w2201) -> ()
      }
    }
  }
  "warrior a" <- 1.0 ("warrior a")
  "hunting b" <- 2.0 ("hunting b")
  "hunting a" <- 1.0 ("hunting a")
  "warrior b" <- 1.0 ("warrior b")
  "Food" <- 0.0
  "People" <- 10
  "Permanent\nland" <- 5.0 ("Permanent\nland")
  "Conquered\nland" <- 0.0 ("Temporary\nland")
  "warrior c" <- 2.0 ("Numeric")
  "Hunters" <- 10 ("Hunters")
  "Unassigned workers" <- 0 ("Unassigned workers")
  "Builders" <- 0 ("Builders")
  "Warriors" <- 0 ("Warriors")
  "Scientists" <- 0 ("Hunters")
  "Crafters" <- 0 ("Builders")
  "Engineers" <- 0 ("Warriors")
  "EP" <- 0.0 ("Engineering\nPoints")
  "Spear level" <- 0 ("Spear level")
  "Net level" <- 0 ("Net level")
  "SP" <- 0.0 ("Numeric")
  "Military\nScience level" <- 0 ("Military level")
  "Dissent" <- 0.0 ("Dissent")
  "Government" <- "Tribe" ("String")
  "Governance\nlevel" <- 0 ("Numeric")
  "Warrior b Gov mult" <- 1 ("Warrior a Gov mult")
  "Land conv mult" <- 0 ("Land conv mult")
  "Temp land change/s" <- 0 ("Temp land captured/s")
  "1-Dissent/100" <- 1.0 ("1-Dissent/100")
  "Bow level" <- 0 ("Numeric")
  "Military Modifier" <- 1.0 ("Military Modifier")
  "Physics level" <- 0 ("Military level")
  "Construction\nlevel" <- 0 ("Numeric")
  "Boat level" <- 0 ("Spear level")
  "Trading level no mod" <- 0 ("Spear level")
  "Economics\nlevel" <- 0 ("Economic\nlevel")
  "Gold dbl" <- 0.0 ("Gold")
  "Taxation\nlevel" <- 0.0 ("Numeric")
  "Taxation\nModifier" <- 1.0 ("Numeric")
  "Farming level" <- 0 ("Numeric")
  "Biology\nlevel" <- 0 ("Numeric")
  "Hut level" <- 0 ("Numeric")
  "Road level" <- 0 ("Numeric")
  "Brick house level" <- 0 ("Numeric")
  "Build points" <- 0 ("Numeric")
  "Non-land production multiplier" <- 1 ("Numeric")
  "Dissent \nmultiplication\nmodifier" <- 1.0 ("Dissent multiplication modifiers")
  "Hut non-land prod mod" <- 1 ("Numeric")
  "Hut upkeep" <- 0 ("Numeric")
  "Hut dissent mod" <- 1 ("Numeric")
  "Road land prod mod" <- 1 ("Numeric")
  "Road upkeep" <- 0 ("Numeric")
  "Road expansion bonus" <- 0 ("Numeric")
  "Trading level" <- 0 ("Spear level")
  "Gov building\nupkeep mod" <- 1 ("Numeric")
  "BP upkeep" <- 0.0 ("BP/s")
  "# of level 1 sciences" <- 0 ("Numeric")
  "# of level 2 sciences" <- 0 ("Numeric")
  "# of level 3 sciences" <- 0 ("Numeric")
  "# of level 4 sciences" <- 0 ("Numeric")
  "# of level 5 sciences" <- 0 ("Numeric")
  "# of level 6 sciences" <- 0 ("Numeric")
  "# of level 7 sciences" <- 0 ("Numeric")
  "# of level 8 sciences" <- 0 ("Numeric")
  "# of level 9 sciences" <- 0 ("Numeric")
  "# of level 10 sciences" <- 0 ("Numeric")
  "Hut invested points" <- 0 ("Numeric")
  "Road invested points" <- 0 ("Numeric")
  "Taxes dissent mod" <- 0 ("Numeric")
  "Gold income/s" <- 0.0 ("Gold income/s")
  "Barracks level" <- 0 ("Numeric")
  "Barracks military bonus" <- 1 ("Numeric")
  "Barracks upkeep" <- 0 ("Numeric")
  "Walls level" <- 0 ("Numeric")
  "Wall warrior % equivalent" <- 0 ("Numeric")
  "Wall upkeep" <- 0 ("Numeric")
  "Wall dissent mod" <- 1 ("Numeric")
  "Barracks\ninvested points" <- 0 ("Numeric")
  "Wall invested points" <- 0 ("Numeric")
  "Construction\ntools level" <- 0 ("Numeric")
  "Gold upkeep" <- 0 ("Land conv mult")
  "Construction multiplier" <- 1 ("Construction multiplier")
  "BP income" <- 0.0 ("Construction multiplier")
  "School level" <- 0 ("Numeric")
  "School engineer equivalent" <- 0 ("Numeric")
  "School upkeep" <- 0 ("Numeric")
  "School dissent mod" <- 1 ("Numeric")
  "School invested points" <- 0 ("Numeric")
  "School SP/EP multiplier" <- 1 ("Numeric")
  "Medicine level" <- 0 ("Spear level")
  "Medicine dissent mod" <- 1 ("Spear level")
  "University level" <- 0 ("Numeric")
  "University scientist equivalent" <- 0 ("Numeric")
  "University upkeep" <- 0 ("Numeric")
  "University dissent mod" <- 1 ("Numeric")
  "University\ninvested points" <- 0 ("Numeric")
  "University SP multiplier" <- 1 ("Numeric")
  "Gov populist\nbuildings mod" <- 1 ("Numeric")
  "Gov elitist\nbuildings mod" <- 1 ("Numeric")
  "Dissent mult per\nmilitary building" <- 1 ("Numeric")
  "Gov Economy\nbuildings mod" <- 1 ("Numeric")
  "Food dissent mod" <- 1 ("Numeric")
  "Food consumption\nmultiplier" <- 1 ("Numeric")
  "Food income" <- 0 ("food check")
  "EP income" <- 0.0 ("Construction multiplier")
  "SP income" <- 0.0 ("Construction multiplier")
  "Animal\ndomestication\nlevel" <- 0 ("Numeric")
  "Sword level" <- 0 ("Numeric")
  "Tax method\nlevel" <- 0 ("Numeric")
  "Chariot level" <- 0 ("Numeric")
  "Siege weapon\nlevel" <- 0 ("Numeric")
  "Writing level" <- 0 ("Numeric")
  "Aqueduct level" <- 0 ("Numeric")
  "Aqueduct upkeep" <- 0 ("Numeric")
  "Aqueduct dissent mod" <- 1 ("Numeric")
  "Aqueduct\ninvested points" <- 0 ("Numeric")
  "Mansion level" <- 0 ("Numeric")
  "Mansion upkeep" <- 0 ("Numeric")
  "Mansion dissent mod" <- 1 ("Numeric")
  "Mansion\ninvested points" <- 0 ("Numeric")
  "Harbor level" <- 0 ("Numeric")
  "Harbor upkeep" <- 0 ("Numeric")
  "Harbor expansion bonus" <- 0 ("Numeric")
  "Harbor\ninvested points" <- 0 ("Numeric")
  "Circus/arena level" <- 0 ("Numeric")
  "Circus upkeep" <- 0 ("Numeric")
  "Circus dissent mod" <- 1 ("Numeric")
  "Circus\ninvested points" <- 0 ("Numeric")
  "Temple level" <- 0 ("Numeric")
  "Temple upkeep" <- 0 ("Numeric")
  "Temple dissent mod" <- 1 ("Numeric")
  "Temple\ninvested points" <- 0 ("Numeric")
  "SP/EP multiplier" <- 0.0 ("Construction multiplier")
  "Harbor military mod" <- 1 ("Numeric")
  "Production\nlevel" <- 0 ("Numeric")
  "Tier 1\nproducts" <- 0.0 ("Gold")
  "Tier 2\nproducts" <- 0.0 ("Gold")
  "Tier 3\nproducts" <- 0.0 ("Gold")
  "Tier 4\nproducts" <- 0.0 ("Gold")
  "Tier 1\nproducts\nupkeep" <- 0.0 ("Gold")
  "Tier 2\nproducts\nupkeep" <- 0.0 ("Gold")
  "Tier 3\nproducts\nupkeep" <- 0.0 ("Gold")
  "Tier 4\nproducts\nupkeep" <- 0.0 ("Gold")
  "Temple SP/EP multiplier" <- 1 ("Numeric")
  "Aqueduct food multiplier" <- 1 ("Numeric")
  "Gold" <- 0 ("Gold")
  "Optics\nlevel" <- 0 ("Optics\nlevel")
  "Electronics\nlevel" <- 0 ("Optics\nlevel")
  "Vehicle\nlevel" <- 0 ("Optics\nlevel")
